vi "UNITEST MAIN v01.1.vi"() -> ()   [LabVIEW 2025]
uses:
  controls/LAB-IQ UI Data.ctl
  HEAVE vi's/Heave Write enum.ctl
  HEAVE vi's/Heave Right enum.ctl
  d081153b-36ca-4bc4-8478-749476f82ba4.vi
  02c5850b-52e8-4ed5-91f8-6f0ad62f4994.vi
  1223eb78-e4c4-4b69-bf80-185c82055158.vi
  e5651a45-6a49-4a3f-b503-ff1eaf449b4a.vi
  4095ce77-506c-41ec-8143-cc58e62a390f.vi
  support/Message Queue/Enqueue Message (Single).vi
  <vilib>/Utility/error.llb/Error Cluster From Error Code.vi
  <vilib>/ErrorRing/Error Ring.xnode
  support/Message Queue/LAB-IQ Message Queue.lvlib
  support/User Event - Stop/LAB-IQ User Event - Stop.lvlib
  SWAY vi's/Sway Write enum.ctl
  1202965f-721d-4349-8d61-5de826f379ef.vi
  SWAY vi's/Sway Right enum.ctl
panel:
  out "HEAVE ENABLE":bool
  in  "SPARE  5":u8
  in  "Manual Write SWAY":bool
  out "SWAY WRITE":string
  in  "SPARE  4":u8
  in  "SPARE  3":u8
  in  "SPARE 2":u8
  in  "SPARE 1":u8
  out "Spare 15":u8
  out "Spare 14":u8
  out "Spare 13":u8
  out "Spare 12":u8
  out "Spare 11":u8
  out "Spare 10":u8
  out "Spare 9":u8
  out "Spare 8":u8
  out "Spare 7":u8
  out "Spare 6":u8
  out "Spare 5":u8
  out "Spare 4":u8
  out "Spare 3":u8
  out "Spare 2":u8
  out "Spare 1":u8
  out "Node Id":u8
  out "Read SWAY Temp":bool
  out "fwMinor":u8
  out "fwMajor":u8
  out "faultCode":u16
  out "Rotary POSE":sgl format="%#.6f"
  out "SWAY POSE":sgl format="%#.6f"
  out "Homed":u8
  out "State":u8
  out "Ack ID":u16
  in  "SPEED":sgl=10000.0
  in  "Distance":sgl=10000.0
  in  "Mode Command":u8=2
  out "Sequence ID":u16
  out "error out Read SWAY":errorcluster
  out "error out Write  SWAY":errorcluster
  out "SWAY READ":string
  in  "min_finetune_floor":dbl=0.15
  in  "min_deadband_floor":dbl=0.05
  in  "fine_tune_pct":dbl=100.0
  out "Start Test Temp":bool
  in  "STOP":bool
  in  "AppLoadSeq scratch":bool
  out "Pulse delta":dbl
  in  "Fine Tune Zone":dbl=10.0
  in  "PID Delay (sec)":dbl=1.0 format="%#_6p"
  in  "Max_pos_limit":dbl=50000000.0
  in  "Min_pos_limit":dbl
  in  "i_limit":dbl=10.0
  in  "Max Step Linit":dbl=10.0
  in  "Init Step":dbl=10.0
  in  "pct_scale":dbl=100.0
  in  "Deadband":dbl=0.1
  in  "Kd":dbl
  in  "Ki":dbl
  in  "Kp":dbl=1.0
  out "Current Position":dbl
  in  "Set Load":dbl
  in  "Current Load":dbl
  in  "Manual Write Heave & Surge":bool
  out "Heave and Surge Write":string
  in  "Heave Loop Delay":dbl
  in  "Heave PID Speed":dbl=15.0
  in  "Surge Jog Speed":dbl=1.0 format="%.4f"
  in  "Heave Jog Speed":dbl=15.0
  in  "SPARE 4":u8
  in  "SPARE 3":u8
  in  "SPARE 2":u8
  in  "SPARE 1":u8
  out "Spare 15":u8
  out "Spare 14":u8
  out "Spare 13":u8
  out "Spare 12":u8
  out "Spare 11":u8
  out "Spare 10":u8
  out "Spare 9":u8
  out "Spare 8":u8
  out "Spare 7":u8
  out "Spare 6":u8
  out "Spare 5":u8
  out "Spare 4":u8
  out "Spare 3":u8
  out "Spare 2":u8
  out "Spare 1":u8
  out "Node Id":u8
  out "Read Heave Temp":bool
  out "fwMinor":u8
  out "fwMajor":u8
  out "faultCode":u16
  out "SURGE POSE":sgl format="%#.6f"
  out "HEAVE POSE":sgl format="%#.6f"
  out "Homed":u8
  out "State":u8
  out "Ack ID":u16
  in  "SPEED":sgl=10000.0
  in  "Distance":sgl=10000.0
  in  "Mode Command":u8=2
  out "Sequence ID":u16
  out "error out Read":errorcluster
  out "error out Write":errorcluster
  out "Heave and Surge Read":string
  out "Load Cell Temp":bool
  in  "Stop Scratch":bool
  in  "Enter Fixed SRR 2":dbl min=0.0 max=0.0 format="%.3f"
  in  "E.Velocity 2":bool=TRUE caption="SRR"
  out "Message":string="Load Entered is out of range!!!"
  in  "Tab Control 3":T1(tab)
  in  "Tab Control 5":enum32{""}(tab)
  in  "Tab Control 14":T2(tab)=enum."Motor Load"
  in  "Ramp MulFac":dbl=2.0
  in  "pulses LoadDiffRamp(2..10)":dbl=9.0
  in  "PulseControlRamp(diff<=3N)":dbl=5.0 min=1.0 max=1000.0 step=1.0 format="%#.1f"
  in  "SetLoadDeadband(%) Load(0-10N)":dbl=0.1 min=0.0001 max=100.0 step=0.0001 format="%#.6f"
  in  "PID gains out delay (microForce)":T3={"proportional gain (Kc)"=300.0, "integral time (Ti, min)"=0.00011, "derivative time (Td, min)"=0.0} {"derivative time (Td, min)" format="%.3f"; "integral time (Ti, min)" min=1e-05 max=100.0 step=1e-06 format="%.6f"; "proportional gain (Kc)" format="%.3f"}
  in  "Ramp":bool
  in  "Gain 2":dbl=0.016
  in  "pulses LoadDiff(2..10)":dbl=10.0
  in  "pulses LoadDiff(11..50)":dbl=40.0
  in  "PulseControl(diff<=3N)":dbl=1.0 min=1.0 max=1000.0 step=1.0 format="%#.1f"
  out "SetLoadDeadband(%)  2":dbl=1.0 min=0.001 max=100.0 step=0.001 format="%#.6f"
  in  "Dummy Run":bool
  out "Vertical load (N)":dbl format="%#.3f"
  in  "AutoTune":bool
  in  "Offset  3":dbl=1.5
  in  "apply load":bool
  in  "Enter ByPass Load":dbl
  in  "reinit 3":bool=TRUE
  in  "output range delay":cluster{"output high":dbl, "output low":dbl}={"output high"=100.0, "output low"=-100.0} {"output low" format="%.2f"; "output high" format="%.2f"}
  in  "PID gains out delay":T3={"proportional gain (Kc)"=30.0, "integral time (Ti, min)"=0.00101, "derivative time (Td, min)"=0.0} {"derivative time (Td, min)" format="%.3f"; "integral time (Ti, min)" min=1e-05 max=100.0 step=0.0001 format="%.4f"; "proportional gain (Kc)" format="%.3f"}
  in  "Bypass Load":bool
  in  "pulsesSent":dbl=200.0
  out "pulses":dbl
  out "actpid":dbl
  out "gFF Rot 7":cluster{dbl, dbl, dbl}(graph)
  in  "pulses LoadDiff(21..1000)":dbl=40.0
  in  "Delay":dbl=1.5 min=0.001 max=5.0 step=0.001 format="%#.6f"
  in  "deadband":dbl=0.2
  in  "Tab Control 26":enum32{"Page 1", "Page 2"}(tab)
  in  "ClearAll":bool
  out "Mz(Nm)":dbl[](array[numeric])
  out "My(Nm)":dbl[](array[numeric])
  out "Mx(Nm)":dbl[](array[numeric])
  in  "Save Dwell":dbl=0.015 caption="Save Dwell (sec)" min=0.0 max=5.0 step=0.001 format="%.3f"
  out "Mx":dbl[](graph)
  out "My":dbl[](graph)
  out "Mz":dbl[](graph)
  out "Fx(N)":dbl[](graph)
  out "Fy(N)":dbl[](graph)
  out "Fz(N)":dbl[](graph)
  in  "ZeroAll":bool
  in  "Acq Delay (ms)":dbl=10.0
  in  "Burst Delay (ms)":dbl=10.0
  out "model":string
  out "SN":i32
  out "FFx(N)":dbl[](array[numeric])
  in  "Sensor IP":string="192.168.1.100"
  in  "Port":i32=8080
  out "FFy(N)":dbl[](array[numeric])
  out "Load(N)":dbl[](array[numeric])
  out "AE":bool
  in  "delete Handle":bool
  in  "Create Handle":bool=TRUE
  out "ft_data":dbl[](array[numeric])=[1.0, 1.0, 1.0, 1.0, 1.0, 1.0]
  out "ft_range":dbl[](array[numeric])=[1.0, 1.0, 1.0, 1.0, 1.0, 1.0]
  in  "stop 6":bool
  out "running_flag":bool
  out "ft_udp_handle":i32
  out "get-data-return":i32
  out "get-range-return":i32
  out "zero-return":i32
  out "filter-return":i32
  out "initial-return":i32
  out "deleteHandle-result":i32
  in  "Tab Control 19":enum32{"Platform COM", "Config ", "DevInfo"}(tab)=enum."Config "
  in  "SAMPLES":dbl=100.0
  in  "Re-initilaize":bool
  in  "Filter ON/OFF":bool=TRUE
  in  "TracHomeSurgeOffsetCounts 10MM":dbl=505100.0
  in  "TracHomeSwayOffsetCounts 10MM":dbl=1432.0
  in  "Acoustic Emission:":dbl=1.0 min=0.0001 max=200.0 step=0.0001 format="%.4f"
  in  "Apply Filter (FF)":bool
  in  "Filter% 2":dbl=50.0 min=50.0 max=100.0 step=0.1 format="%.1f"
  in  "Apply Filter (Load)":bool=TRUE
  in  "Filter%":dbl=80.0 min=50.0 max=100.0 step=0.1 format="%.1f"
  in  "Sway distance (mm)":dbl=245.0
  in  "Surge distance (mm)":dbl=370.0
  in  "DataSavingLoopDelay(ms)":dbl=15.0
  in  "SAVE  2":bool
  in  "Enter Distance":bool caption="Enter Counts"
  in  "Sway Counts:":dbl=100.0 min=0.0 max=100000000.0 step=1.0 format="%.2f"
  in  "Distance (mm): 3":dbl=100.0 caption="Distance (mm):" min=0.0 max=1500.0 step=0.001 format="%.5f"
  in  "Surge Counts:":dbl=100.0 min=0.0 max=100000000.0 step=1.0 format="%.1f"
  in  "Distance (mm): 2":dbl=100.0 caption="Distance (mm):" min=0.0 max=1500.0 step=0.0001 format="%.3f"
  in  "Distance (mm):":dbl=100.0 min=0.0 max=1500.0 step=0.001 format="%.5f"
  in  "Heave Counts:":dbl=100.0 min=0.0 max=100000000.0 step=1.0
  in  "LRMHomeSurgeOffsetCounts":dbl=307197.0
  in  "LRMHomeSwayOffsetCounts":dbl=26880.0
  in  "TracHomeSurgeOffsetCounts 20MM":dbl=505100.0
  in  "TracHomeSwayOffsetCounts 20MM":dbl=1432.0
  in  "RotHomeSwayOffsetCounts":dbl=14656.0
  in  "RotHomeSurgeOffsetCounts":dbl=311465.0
  in  "Heave distance":dbl=340.0
  out "Zmm":dbl=1600.0
  out "Heave Pulses/mm":dbl=1600.0
  out "Surge Pulses/mm":dbl=1600.0
  out "Sway Pulses/mm":dbl=320.0
  in  "Heave Pitch":dbl=4.0
  in  "Surge Pitch":dbl=3.0
  in  "Sway Pitch":dbl=2.0
  in  "Heave PPR":dbl=6400.0
  in  "Surge PPR":dbl=6400.0
  in  "Sway PPR":dbl=6400.0
  in  "GUI":T4(tab)
  in  "Platform Settings":bool caption="Password"
  in  "Configure":bool caption="Password"
  in  "Home":bool caption="Password"
  in  "EXIT":bool
  in  "Analysis":bool caption="Password"
  in  "service 2":bool caption="Password"
  in  "MainPage":T5(tab)=enum."HOME"
  in  "Select Load Head":bool
  in  "Notes :":string
  in  "FILE":string
  in  "Sample ID :":string
  in  "Operator ID :":string
  in  "Operator Name :":string
  in  "Auto":bool caption="Power Status"
  out "mm/s  Surge":dbl=7.0 caption="Jog" min=0.001 max=50.0 step=0.0001 format="%.2f"
  in  "Update Surge Speed":bool
  out "Drive Error":string
  in  "Disable Axis Jog Soft Limits":bool
  out "mm/s  Sway":dbl=7.0 caption="Jog" min=0.001 max=50.0 step=0.0001 format="%.2f"
  out "Sway and Surge COM Status":bool=TRUE caption="Load COM Status"
  out "Heave COM Status":bool=TRUE caption="Load COM Status"
  in  "Enable Platform":bool
  in  "Surge Forward Main":bool
  in  "Surge Backward Main":bool
  in  "Sway Right Main":bool
  in  "Sway Left Main":bool
  in  "Heave Down Main":bool
  in  "Heave Up main":bool
  in  "Update Sway Speed":bool
  in  "Update Heave Speed":bool
  out "mm/s Heave":dbl=7.0 caption="Jog" min=0.001 max=30.0 step=0.0001 format="%.2f"
  in  "mm/sec":dbl=1.0 caption="Jog" min=0.001 max=50.0 step=0.001 format="%.2f"
  in  "mm":dbl=0.001 caption="Jog" min=0.001 max=200.0 step=0.0001 format="%#.3f"
  in  "Surface Analysis":bool
  in  "Imaging":bool
  in  "Image Analysis":bool
  in  "Post Analysis":bool
  in  "SSP 0.75":bool
  in  "SSP 0.5":bool
  in  "SSP 0.3":bool
  in  "Warning":enum32{"Page 2"}(tab)
  in  "gui GIF":enum32{"Check", "Deca", "kilo", "Micro"}(tab)
  out "Communication is established":bool=TRUE caption="Load COM Status"
  in  "Reference Sample":u16(ring) items=["None", "Brass", "Aluminium", "Mild Steel"]
  out "Load Cell Communication Slide":u8(slide)=1 min=1 max=10 step=1 scale=0.0..10.0
  in  "com 3":bool
  out "com":bool
  out "DecaForce COM Status":bool caption="Load COM Status"
  in  "Loading Mode":u16(ring) items=["Constant", "Ramp", "Steps", "Indentation"]
  in  "Enter the CoF Trip":dbl=1.0
  in  "Enter the Friction Force Trip":dbl=520.0 min=500.0 max=500.0 step=1.0 format="%#.1f"
  in  "Enter the Normal load Trip":dbl=520.0 min=500.0 max=500.0 step=0.001 format="%.3f"
  in  "KiloForce":bool
  in  "DecaForce":bool
  in  "MicroForce":bool
  in  "LHBack":bool
  in  "LHNext":bool
  in  "Load Selection":T6(tab)
  in  "Enter the Load  (N)":dbl=2.0 caption="Enter the Load (N)" min=2.0 max=50.0 step=0.1 format="%#.4f"
  in  "Enter the Final Load (N)":dbl=1.0 min=0.0 max=500.0 step=1.0 format="%#.0f"
  in  "Update":bool
  in  "Enter the Loading Rate (N/min)":dbl=60.0 min=60.0 max=1200.0 step=0.1 format="%.2f"
  out "Warning 2":bool
  in  "Stribeck Table  For loading":string[][](table)=[["", "", ""], ["", "", ""], ["", "", ""], ["", "", ""]]
  in  "Stribeck table":bool
  in  "seq":bool=TRUE
  in  "Clear 3":bool
  in  "Indentation":string[][](table)=[["Detection", "5", "2"], ["Unload", "0", "5"], ["Load", "10", "2"], ["Unload", "0", "5"], ["Detection", "5", "2"], ["Unload", "0", "5"]]
  in  "Multipoint":bool caption="Singlepoint"
  in  "AppLoad 4":bool
  in  "zNL":bool
  out "NL disp":dbl caption="Normal Load ( N )" min=-2000.0 max=2000.0 step=0.0001 format="%.1f"
  in  "Traction":bool
  in  "Surge Forward MM":bool
  in  "Surge Backward MM":bool
  in  "M3 Image":enum32{"Page 1", "Page 2"}(tab)
  in  "String 39":string="Jog heave to bring the upper sample closer to the lower sample within 1mm."
  in  "Sway Left MM":bool
  in  "Sway Right MM":bool
  in  "Disable Axis Jog Soft Limits":bool
  in  "mm":dbl=0.001 caption="Jog" min=0.001 max=5.0 step=0.0001 format="%#.3f"
  in  "Heave Down MM":bool
  in  "Heave Up MM":bool
  in  "Wear Track Diameter (mm)":dbl=5.0 caption="Wear Track Diameter (mm):" min=1.0 max=30.0 step=1.0 format="%.2f"
  in  "Set WTD":bool
  in  "HomeScratch":bool
  in  "HomeRot":bool
  in  "PlaceModule":bool
  in  "Motion Mode:":u16(ring) items=["Uniform Rotation", "Angular Oscillation", "Stribeck ", "Steps"]
  in  "LR Sway":bool
  in  "Rot Hor":bool
  in  "Rot Ver":bool
  in  "Scratch":bool
  in  "LR Cam":bool
  in  "MMBack":bool
  in  "MMNext":bool
  in  "Rotary Module Selection":T7(tab)
  in  "SPEED SELECTION :":enum32{"Speed in RPM", "Speed in m/sec"}(radio)=enum."Speed in m/sec"
  in  "TEST SELECTION":enum32{"Time", "Cycle"}(radio)
  in  "Enter the Speed(mm/sec)":dbl=1.0 min=0.1 max=10.0 step=0.1 format="%.1f"
  in  "Enter the Speed(RPM)":dbl=45.0 min=5.0 max=300.0 step=1.0
  in  "Enter the Frequency (Hz)":dbl=1.0 min=0.1 max=10.0 step=0.1 format="%.1f"
  in  "Enter the Angle (Deg)":dbl=45.0 min=5.0 max=300.0 step=1.0
  in  "Angular Oscillation Set":bool
  in  "Rotary Tab":enum32{"Page 1", "Page 2"}(tab)
  out "e.v/ssr 2":enum32{"E.V", "SSR"}(tab)
  in  "Enter the Final E.Velocity (m/s) 2":dbl=1.0 min=0.001 max=4.0 step=0.001 format="%.3f"
  in  "Enter initial E.Velocity (m/s) 2":dbl=2.0 min=0.001 max=4.0 step=0.001 format="%.3f"
  in  "Enter Fixed E.Velocity 2":dbl=1.0 min=0.001 max=2.0 step=0.001 format="%.3f"
  in  "Enter Final SRR 2":dbl=1.0 min=0.001 max=1.0 step=0.001 format="%.2f"
  in  "Enter initial SRR 2":dbl=1.0 min=0.001 max=1.0 step=0.001 format="%.2f"
  out "Final Speed (RPM) 3":dbl=1.0 min=0.1 max=3000.0 step=0.1 format="%.1f"
  out "Initial Speed (RPM) 2":dbl=100.0 min=0.1 max=3000.0 step=0.1 format="%.1f"
  in  "Enter the Final Velocity (m/s) 3":dbl=1.0 min=0.001 max=2.0 step=0.001 format="%.3f"
  in  "Enter initial Velocity (m/s)  3":dbl=2.0 min=0.001 max=2.0 step=0.001 format="%.3f"
  out "Ramp Up 2":bool caption="Ramp Down"
  in  "File Path :  2":path
  in  "Import 2":bool
  in  "Save 2":bool
  in  "SPEED SELECTION : rotary":enum32{"Speed in Rpm", "Speed in m/sec"}(radio)=enum."Speed in m/sec"
  in  "calculate rotary":bool
  in  "String 45":string="File Path Location : C:-->LAB-IQ 150 --> User Defined\n                                       Protocol-->File.txt"
  in  "Step Speed":enum32{"Step Speed", "Step (load-Speed)"}(tab)
  in  "StepTable For Speed":string[][](table)=[["", "", ""], ["", "", ""], ["", "", ""], ["", "", ""]]
  in  "StepTable For Load-Speed":string[][](table)=[["", "", ""], ["", "", ""], ["", "", ""], ["", "", ""]]
  in  "StepTable For Speed 3":string[][](table)=[["", "", ""], ["", "", ""], ["", "", ""], ["", "", ""]]
  in  "Motion Direction:  3":u16(ring) items=["Clockwise", "Counter Clockwise"]
  out "Humidity  Status  3":bool caption="Communication Status"
  out "Low Temp  Status  2":bool caption="Communication Status"
  out "TK4 status 2":bool caption="Communication Status"
  in  "String 40":string="Before selecting Acoustic make sure the sensor output pin is connected to A4."
  in  "Stage Temperature":dbl[](array[numeric])=[150.0, 230.0, 300.0, 350.0, 400.0, 450.0, 500.0]
  in  "Sample Temperature":dbl[](array[numeric])=[100.0, 150.0, 200.0, 250.0, 300.0, 350.0, 400.0]
  in  "Humidity (Amb)":bool
  in  "Clear List":bool
  out "Sensors Picked":string
  in  "Add to list":bool
  in  "Wear":bool
  in  "Vibration":bool
  in  "Humidity (Chamber)":bool
  in  "Temperature (Chamber)":bool
  in  "ECR":bool
  in  "Temperature (Amb)":bool
  in  "Microphone":bool
  in  "Acoustic Emission 3":bool
  in  "SNext":bool
  in  "APBack":bool
  in  "Enter the Temperature (°C):":dbl
  in  "Enter the Stage \nTemperature (°C):":dbl=20.0 min=20.0 max=150.0 step=1.0 format="%#.0f"
  in  "Enter the Humidity (%Rh):":dbl=30.0 min=30.0 max=85.0 step=1.0
  in  "Low Temp":bool
  in  "High Temp":bool
  in  "Humidity":bool
  in  "Main Screen Tab":T8(tab)
  in  "ClrLog":bool
  out "Trip Log":string
  in  "Start Test":bool
  out "Test status":bool caption="Test Status"
  out "AR Led":bool caption="AR"
  out "Data":bool=TRUE
  out "Health":bool=TRUE
  out "Sway COM Status":bool=TRUE caption="Load COM Status"
  out "Heave COM Status":bool=TRUE caption="Load COM Status"
  in  "Grp Tab":enum32{"Rot/LRM", "FBT"}(tab)
  in  "Sub Graph":T9(tab)
  in  "Speed Reset Graph":bool
  in  "Speed Tab":enum32{" Rotary Disc", "MTM Ball", "MTM Disc"}(tab)
  out "speed mm/sec":dbl(graph)=0.13298760003255525
  out "MTM BALL SPEED":dbl(graph)=0.13298760003255525
  out "MTM DISC  SPEED":dbl(graph)=0.13298760003255525
  in  "Temperature Reset":bool
  out "Temperature (deg c)":dbl(graph)=0.13298760003255525
  in  "ECR RESET":bool
  out "ECR":dbl(graph)=0.13298760003255525
  out "Acoustic Emission (mV)":dbl min=0.0 max=5000.0 step=0.1
  in  "Aqucostic Reset Graph":bool
  out "gACQUOS":dbl(graph)=0.13298760003255525
  in  "Humidity Reset Graph":bool
  out "HumrGp":dbl(graph)=0.13298760003255525
  out "SD (mm)":dbl caption="Sliding Distance ( mm )" min=-200.0 max=200.0 step=0.1 format="%.4f"
  in  "Siliding distance Reset Graph":bool
  out "SDGp":dbl(graph)=0.13298760003255525
  out "Hymidity":bool
  in  "Humidity Disable trip":bool=TRUE
  in  "CoF Trip  2":dbl=540.0 min=100.0 max=540.0 step=1.0
  out "Depth Trip":dbl=600.0
  in  "Depth Trip":bool=TRUE
  out "Weart Deapth":bool
  in  "Depth Reset Graph":bool
  out "Weart":bool
  in  "Depthz":bool
  out "Depth (µm)":dbl min=-200.0 max=200.0 step=0.1 format="%.1f"
  out "WearGp":dbl(graph)=0.13298760003255525
  out "NL Trip 2":dbl=600.0
  out "Load pid":bool
  in  "Load Disable Trip":bool=TRUE
  in  "Load Reset Graph":bool
  out "NL Display 4":dbl caption="Normal Load ( N )" min=-2000.0 max=2000.0 step=0.0001 format="%.1f"
  out "Main Chart 3":cluster{dbl, "NL disp":dbl, dbl}(graph)
  in  "FF Tab":T10(tab)
  in  "COF Reset Graph":bool
  in  "COF Disable Trip":bool=TRUE
  out "COF TRIP":dbl=600.0
  out "COF MAIN CHART":cluster{dbl, "NL disp":dbl, dbl}(graph)
  out "Friction Force (N)":dbl min=-2000.0 max=2000.0 step=0.0001 format="%.1f"
  in  "FF Reset Graph":bool
  in  "FF Disable Trip":bool=TRUE
  out "FF TRIP":dbl=600.0
  out "FF MAIN CHART":cluster{dbl, "NL disp":dbl, dbl}(graph)
  in  "BACK":bool
  out "Ambient \nTemperature":dbl min=0.0 max=5000.0 step=0.1 format="%.1f"
  out "Ambient\n Humidity":dbl min=0.0 max=5000.0 step=0.1 format="%.2f"
  out "NL disp 2":dbl caption="Normal Load ( N )" min=-2000.0 max=2000.0 step=0.0001 format="%.1f"
  out "Set Humidity":dbl caption="Set Humidity  (% Rh)" min=-2000.0 max=2000.0 step=1.0 format="%.1f"
  out "humidity disp":dbl caption="Humidity (% Rh)" min=-2000.0 max=2000.0 step=1.0 format="%.1f"
  in  "Humidity On":bool
  in  "zNL 2":bool
  out "NLt":bool
  in  "Load En":bool
  out "Freq (Hz)":dbl min=0.0 max=5000.0 step=0.1 format="%.4f"
  out "HumCOMStatus":bool caption="Communication Status"
  out "Load Communication":bool
  in  "Temp Tabs":enum32{"Low Temp", "High Temp"}(tab)=enum."High Temp"
  out "Controller  Status":bool
  out "ChamberTemp":dbl format="%#.1f"
  in  "SetTmp":dbl=-190.0 caption="Set Temperature (Deg C)" min=-190.0 max=100.0 step=1.0 format="%.1f"
  in  "Cooling":bool
  in  "Heater":bool
  out "TK4 status":bool caption="Controller  Status"
  out "ChamberTemp":dbl format="%#.1f"
  in  "SetTmp":dbl caption="Set Temperature (Deg C)" min=0.0 max=1000.0 step=1.0 format="%.1f"
  in  "Set Load (N)":dbl=100.0 min=0.01 max=1500.0 step=0.01 format="%.1f"
  in  "Time Tab":enum32{"cycles", "duration"}(tab)=enum."duration"
  out "Test Duration 4":dbl=600.0 caption="Test Duration\n(HH:MM:SS)" min=0.0083 max=180000.0 step=0.0001 format="%<%H:%M:%S>t"
  out "TEST CYCLE":dbl min=0.0 max=5000.0 step=0.01 format="%.2f"
  in  "TOTAL CYCLES":dbl min=0.0 max=5000.0 step=0.1 format="%.4f"
  out "Time ( HH:MM:SS ) 2":dbl min=0.0 max=144000.0 step=1.0 format="%<%H:%M:%S>t"
  in  "Test Duration":dbl=600.0 caption="Test Duration\n(HH:MM:SS)" min=0.0083 max=180000.0 step=0.0001 format="%<%H:%M:%S>t"
  in  "Main Speed Tab":enum32{"ROTARY", "TRACTION"}(tab)
  in  "SPEED TAB":enum32{"RPM", "m/sec"}(tab)
  out "Speed (RPM)":dbl min=0.0 max=5000.0 step=0.1 format="%.1f"
  out "Set Speed":dbl caption="Set Speed (RPM)" min=0.0 max=1500.0 step=0.1 format="%.1f"
  out "Speed (m/sec)":dbl min=0.0 max=5000.0 step=0.001 format="%.4f"
  out "Set Speed (m/sec)":dbl min=0.0 max=1500.0 step=0.001 format="%.4f"
  in  "MTM MOTOR DISPLAY":enum32{"MTM RPM", "MTM m/sec"}(tab)
  out "Disc Speed (RPM)":dbl min=0.0 max=1500.0 step=0.1 format="%.1f"
  out "Ball Speed (RPM)":dbl min=0.0 max=1500.0 step=0.1 format="%.1f"
  out "Disc Speed (m/sec)":dbl min=0.0 max=1500.0 step=0.1 format="%.1f"
  out "Ball Speed (m/sec)":dbl min=0.0 max=1500.0 step=0.1 format="%.1f"
  in  "Angle and Frequency":enum32{"angular", "lrm"}(tab)
  out "Angle (Deg)":dbl min=0.0 max=5000.0 step=0.01 format="%.2f"
  out "Stroke (mm)":dbl min=0.0 max=5000.0 step=0.01 format="%.2f"
  in  "Analysis Home":bool
  in  "Password":string
  in  "Home Service":bool
  in  "Advanced Setting":bool
  in  "About Tab":enum32{"Primary"}(tab)
  in  "ECR Port:":refnum<visa-resource-name>="COM10"
  in  "Ramp Port:":refnum<visa-resource-name>="COM10"
  in  "Installation/Replacement completed":bool
  in  "Loahead":bool
  in  "Heave and Surge COM Port:":refnum<visa-resource-name>="COM9"
  in  "Sway COM Port:":refnum<visa-resource-name>="COM10"
  in  "Temp Modbus:":refnum<visa-resource-name>="COM14"
  in  "Humidity Port:":refnum<visa-resource-name>="COM10"
  in  "Edit Gain Constants":bool
  in  "Save Gain Constants":bool
  in  "Service About":bool
  # "load Aquisition off"
  # "load Aquisition On"
  # "Configuration"
  # "Limits for Heave Surge and Sway"
  # "Modules Offset Parameters"
  # "Counts-Distance Calculator"
  # "File Name :"
  # "Ensure the traction module is aligned\n horizontally with the stage before ENABLE."
  # "SET JOG SPEED"
  # "JOG MODE"
  # "Module Selection"
  # "Positioning Control"
  # "Connect the controller\ncable to M3"
  # "Environment"
  # "Sensors"
  # "Data Points"
  # "Data Points"
  # "Data Points"
  # "Data Points"
  # "ohms"
  # "Data Points"
  # "Data Points"
  # "Data Points"
  # "LAB-IQ 150 / UNITEST / WO2456 / UT150  v05 / AUGUST 2025"
  # "NOTE: This operation needs to be done only when the machine is ON."
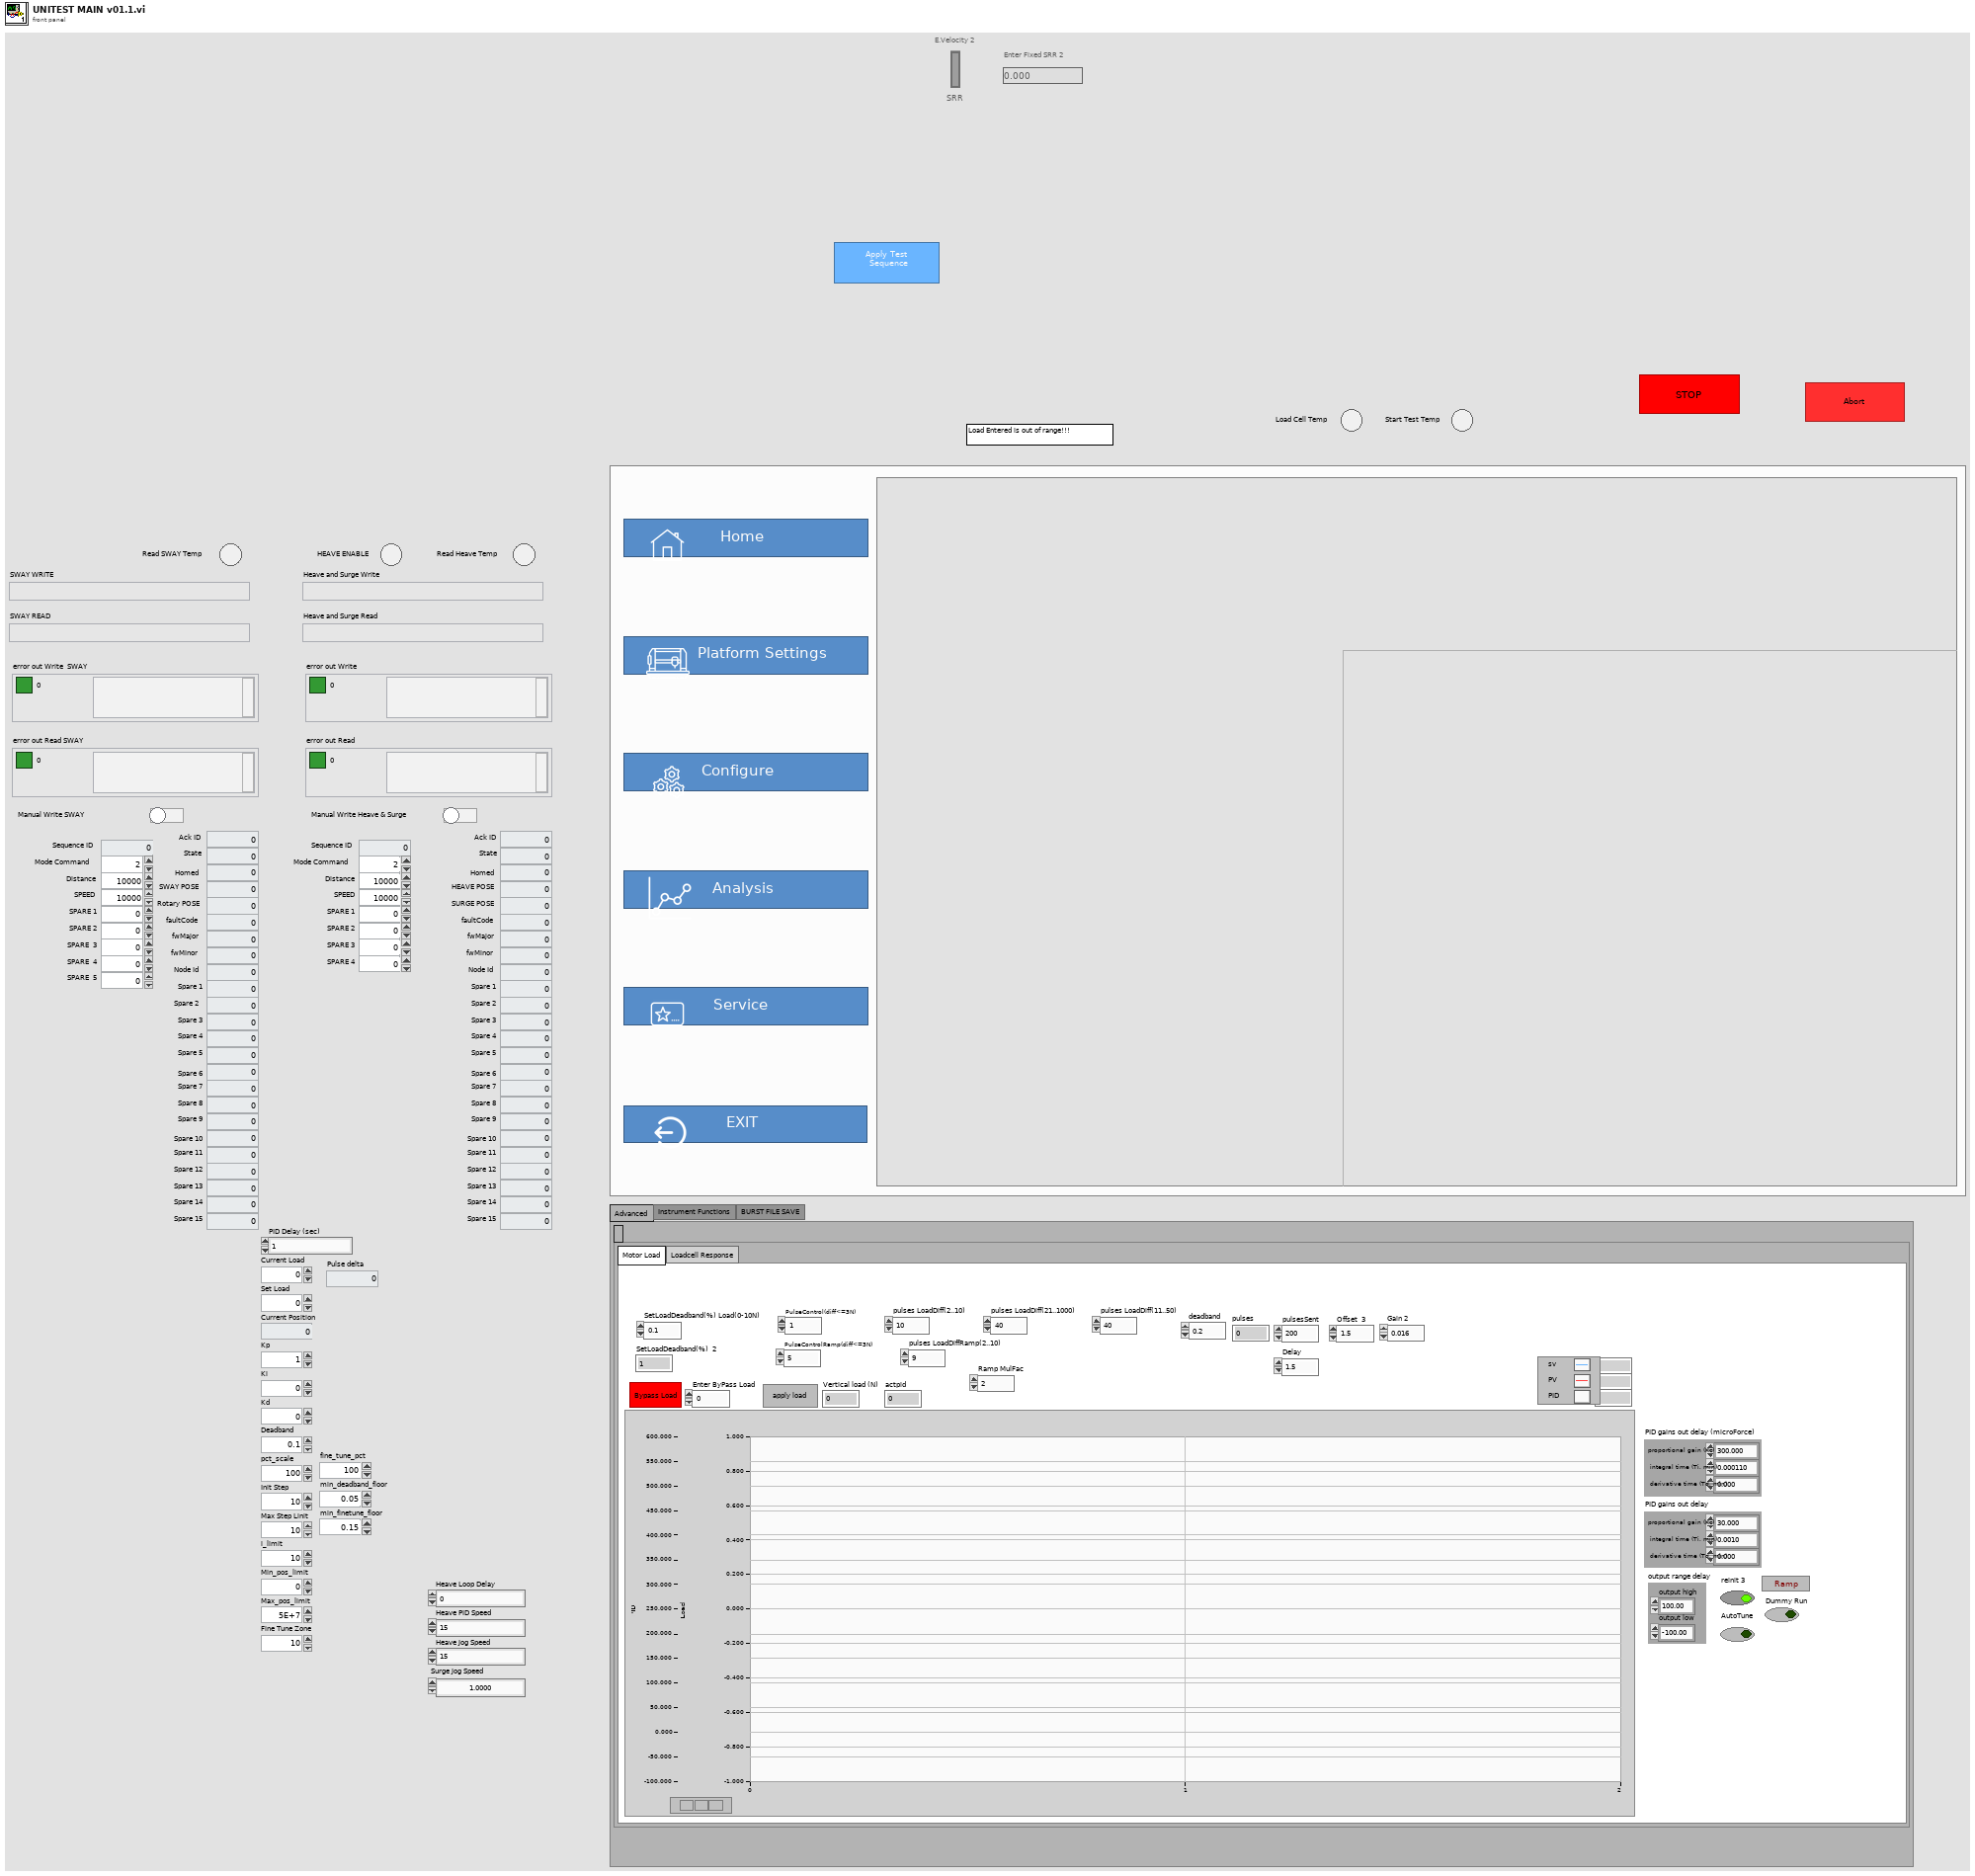
[diagram p1: front panel]
types:
  T1 = enum32{"Advanced", "Motor", "Depth_graph", "UIO Communicator", "Add to list parametrs", "Instrument Functions", "BURST FILE SAVE"}
  T2 = enum32{"LRM heating", "FBT_Heating", "Motor Load", "Loadcell Response", "Voice Load", "Step loading and speed ", "Depth"}
  T3 = cluster{"proportional gain (Kc)":dbl, "integral time (Ti, min)":dbl, "derivative time (Td, min)":dbl}
  T4 = enum32{"Setup", "Load Head", "Motion Module", "Environment", "Begin"}
  T5 = enum32{"Details", "PlatformSetting", "Analysis", "HOME"}
  T6 = enum32{"Constant", "Ramp", "Step", "Indentation"}
  T7 = enum32{"Uniform Rotation", "Angular Oscillation", "Speed Ramp", "Speed Step"}
  T8 = enum32{"  Acquire  ", "Compare Files Rot", "About", "Service"}
  T9 = enum32{"Speed", "Temperature", "ECR", "Acoustic Emission", "Humidity", "Sliding Distance"}
  T10 = enum32{"Coefficient of Friction ", "Friction Force (N)"}
  T11 = typedef "LAB-IQ UI Data.ctl" = cluster{"Main Home Screen":cluster{"GUI":refnum<vi>, "Platform Settings":refnum<vi>, "Configure":refnum<vi>, "Home":refnum<vi>, "EXIT":refnum<vi>, "service 2":refnum<vi>, "MainPage":refnum<vi>, "Analysis":refnum<vi>}, "Platform Settings":cluster{"mm/s  Surge":refnum<vi>, "Update Surge Speed":refnum<vi>, "Drive Error":refnum<vi>, "Disable Axis Jog Soft Limits":refnum<vi>, "mm/s  Sway":refnum<vi>, "Sway and Surge COM Status":refnum<vi>, "Heave COM Status":refnum<vi>, "Enable Platform":refnum<vi>, "Surge Forward Main":refnum<vi>, "Sway Right Main":refnum<vi>, "Sway Left Main":refnum<vi>, "Heave Down Main":refnum<vi>, "Heave Up main":refnum<vi>, "Update Sway Speed":refnum<vi>, "Update Heave Speed":refnum<vi>, "mm/s Heave":refnum<vi>, "mm/sec":refnum<vi>, "mm":refnum<vi>, "Surge Backward Main":refnum<vi>}, "Analysis Screen":cluster{"Analysis Home":refnum<vi>, "Surface Analysis":refnum<vi>, "Imaging":refnum<vi>, "Image Analysis":refnum<vi>, "Post Analysis":refnum<vi>}, "Config Screen":cluster{"Select Load Head":refnum<vi>, "Notes :":refnum<vi>, "FILE":refnum<vi>, "Sample ID :":refnum<vi>, "Operator ID :":refnum<vi>, "Operator Name :":refnum<vi>, "Auto":refnum<vi>}, "Motion Module":cluster{"zNL":refnum<vi>, "NL disp":refnum<vi>, "Rotary Tab":refnum<vi>, "Motion Direction:  3":refnum<vi>, "E.Velocity 2":refnum<vi>, "e.v/ssr 2":refnum<vi>, "Enter Fixed E.Velocity 2":refnum<vi>, "Enter Final SRR 2":refnum<vi>, "Enter initial SRR 2":refnum<vi>, "Enter Fixed SRR 2":refnum<vi>, "Enter the Final E.Velocity (m/s) 2":refnum<vi>, "Enter initial E.Velocity (m/s) 2":refnum<vi>, "Final Speed (RPM) 3":refnum<vi>, "Initial Speed (RPM) 2":refnum<vi>, "Enter the Final Velocity (m/s) 3":refnum<vi>, "Enter initial Velocity (m/s)  3":refnum<vi>, "Ramp Up 2":refnum<vi>, "TEST SELECTION":refnum<vi>, "SPEED SELECTION : ":refnum<vi>, "Angular Oscillation Set":refnum<vi>, "Traction":refnum<vi>, "Step Speed":refnum<vi>, "StepTable For Load-Speed":refnum<vi>, "StepTable For Speed":refnum<vi>, "Surge Forward MM":refnum<vi>, "Surge Backward MM":refnum<vi>, "M3 Image":refnum<vi>, "String 39":refnum<vi>, "Sway Left MM":refnum<vi>, "Sway Right MM":refnum<vi>, "Disable Axis Jog Soft Limits":refnum<vi>, "mm":refnum<vi>, "Heave Down MM":refnum<vi>, "Heave Up MM":refnum<vi>, "Wear Track Diameter (mm)":refnum<vi>, "Set WTD":refnum<vi>, "HomeScratch":refnum<vi>, "HomeRot":refnum<vi>, "PlaceModule":refnum<vi>, "Enter the Angle (Deg)":refnum<vi>, "Enter the Frequency (Hz)":refnum<vi>, "Motion Mode:":refnum<vi>, "LR Sway":refnum<vi>, "Rot Hor":refnum<vi>, "Scratch":refnum<vi>, "LR Cam":refnum<vi>, "MMBack":refnum<vi>, "MMNext":refnum<vi>, "Rot Ver":refnum<vi>, "Rotary Module Selection":refnum<vi>, "calculate rotary":refnum<vi>, "SPEED SELECTION : rotary":refnum<vi>, "Import 2":refnum<vi>, "Save 2":refnum<vi>, "File Path :  2":refnum<vi>, "String 45":refnum<vi>, "StepTable For Speed 3":refnum<vi>, "Enter the Speed(mm/sec)":refnum<vi>, "Enter the Speed(RPM)":refnum<vi>}, "Environmental control":cluster{"Humidity  Status  3":refnum<vi>, "Low Temp  Status  2":refnum<vi>, "TK4 status 2":refnum<vi>, "Stage Temperature":refnum<vi>, "Sample Temperature":refnum<vi>, "Humidity (Amb)":refnum<vi>, "Clear List":refnum<vi>, "Add to list":refnum<vi>, "Wear":refnum<vi>, "Vibration":refnum<vi>, "Humidity (Chamber)":refnum<vi>, "Temperature (Chamber)":refnum<vi>, "ECR ":refnum<vi>, "Temperature (Amb)":refnum<vi>, "Microphone":refnum<vi>, "Acoustic Emission 3":refnum<vi>, "SNext":refnum<vi>, "APBack":refnum<vi>, "Enter the Temperature (°C):":refnum<vi>, "Enter the Stage \nTemperature (°C):":refnum<vi>, "Enter the Humidity (%Rh):":refnum<vi>, "Low Temp":refnum<vi>, "High Temp":refnum<vi>, "Humidity":refnum<vi>, "Sensors Picked":refnum<vi>}, "About Screen":cluster{"Password":refnum<vi>, "Home Service":refnum<vi>, "Advanced Setting":refnum<vi>, "About Tab":refnum<vi>, "ECR Port:":refnum<vi>, "Ramp Port:":refnum<vi>, "Installation/Replacement completed":refnum<vi>, "Loahead":refnum<vi>, "Heave and Surge COM Port:":refnum<vi>, "Sway COM Port:":refnum<vi>, "Temp Modbus:":refnum<vi>, "Humidity Port:":refnum<vi>, "Edit Gain Constants":refnum<vi>, "Save Gain Constants":refnum<vi>}, "Main Screen":cluster{"Main Screen Tab":refnum<vi>, "Angle and Frequency":refnum<vi>, "Stroke (mm)":refnum<vi>, "Angle (Deg)":refnum<vi>, "Main Speed Tab":refnum<vi>, "MTM MOTOR DISPLAY":refnum<vi>, "Disc Speed (m/sec)":refnum<vi>, "Ball Speed (m/sec)":refnum<vi>, "Disc Speed (RPM)":refnum<vi>, "Ball Speed (RPM)":refnum<vi>, "SPEED TAB":refnum<vi>, "Speed (m/sec)":refnum<vi>, "Set Speed (m/sec)":refnum<vi>, "Speed (RPM)":refnum<vi>, "Set Speed":refnum<vi>, "Time Tab":refnum<vi>, "Time ( HH:MM:SS ) 2":refnum<vi>, "Test Duration":refnum<vi>, "Test Duration 4":refnum<vi>, "TEST CYCLE":refnum<vi>, "TOTAL CYCLES":refnum<vi>, "Set Load (N)":refnum<vi>, "Temp Tabs":refnum<vi>, "Heater":refnum<vi>, "TK4 status":refnum<vi>, "ChamberTemp":refnum<vi>, "SetTmp":refnum<vi>, "Controller  Status":refnum<vi>, "ChamberTemp 2":refnum<vi>, "SetTmp 2":refnum<vi>, "Controller  Status 2":refnum<vi>, "ChamberTemp 3":refnum<vi>, "SetTmp 3":refnum<vi>, "Cooling":refnum<vi>, "Load Communication":refnum<vi>, "Ambient \nTemperature":refnum<vi>, "HumCOMStatus":refnum<vi>, "Ambient\n Humidity":refnum<vi>, "Freq (Hz)":refnum<vi>, "Load En":refnum<vi>, "NLt":refnum<vi>, "zNL 2":refnum<vi>, "Humidity On":refnum<vi>, "humidity disp":refnum<vi>, "Set Humidity":refnum<vi>, "NL disp 2":refnum<vi>, "Humidity On 2":refnum<vi>, "humidity disp 2":refnum<vi>, "Set Humidity 2":refnum<vi>, "NL disp 3":refnum<vi>, "AppLoadSeq scratch":refnum<vi>, "Stop Scratch":refnum<vi>, "ClrLog":refnum<vi>, "Trip Log":refnum<vi>, "STOP":refnum<vi>, "Start Test":refnum<vi>, "Test status":refnum<vi>, "AR Led":refnum<vi>, "Data":refnum<vi>, "Health":refnum<vi>, "Sway COM Status":refnum<vi>, "Heave COM Status":refnum<vi>, "Grp Tab":refnum<vi>, "Sub Graph":refnum<vi>, "SD (mm)":refnum<vi>, "Siliding distance Reset Graph":refnum<vi>, "SDGp":refnum<vi>, "Humidity Reset Graph":refnum<vi>, "HumrGp":refnum<vi>, "Acoustic Emission (mV)":refnum<vi>, "Aqucostic Reset Graph":refnum<vi>, "gACQUOS":refnum<vi>, "ECR RESET":refnum<vi>, "ECR":refnum<vi>, "Temperature Reset":refnum<vi>, "Acoustic Emission (mV) 2":refnum<vi>, "Aqucostic Reset Graph 2":refnum<vi>, "gACQUOS 2":refnum<vi>, "ECR RESET 2":refnum<vi>, "ECR 2":refnum<vi>, "Temperature Reset 2":refnum<vi>, "Temperature (deg c)":refnum<vi>, "Speed Reset Graph":refnum<vi>, "Speed Tab":refnum<vi>, "MTM DISC  SPEED":refnum<vi>, "MTM BALL SPEED":refnum<vi>, "speed mm/sec":refnum<vi>, "Hymidity":refnum<vi>, "Humidity Disable trip":refnum<vi>, "CoF Trip  2":refnum<vi>, "Depth Trip":refnum<vi>, "Weart Deapth":refnum<vi>, "Depth Reset Graph":refnum<vi>, "Weart":refnum<vi>, "Depthz":refnum<vi>, "Depth (µm)":refnum<vi>, "WearGp":refnum<vi>, "NL Trip 2":refnum<vi>, "Load pid":refnum<vi>, "Load Disable Trip":refnum<vi>, "Load Reset Graph":refnum<vi>, "NL Display 4":refnum<vi>, "Main Chart 3":refnum<vi>, "BACK":refnum<vi>, "Depth Trip 2":refnum<vi>, "COF TRIP ":refnum<vi>, "Friction Force (N)":refnum<vi>, "FF Reset Graph":refnum<vi>, "FF Disable Trip":refnum<vi>, "FF TRIP":refnum<vi>, "FF MAIN CHART":refnum<vi>, "COF Disable Trip":refnum<vi>, "COF Reset Graph":refnum<vi>, "COF MAIN CHART":refnum<vi>, "FF Tab":refnum<vi>, "Start Test Temp":refnum<vi>}, "Loading":cluster{"Indentation":refnum<vi>, "Reference Sample":refnum<vi>, "Load Cell Communication Slide":refnum<vi>, "com 3":refnum<vi>, "com":refnum<vi>, "DecaForce COM Status":refnum<vi>, "Update":refnum<vi>, "Clear 3":refnum<vi>, "seq":refnum<vi>, "Stribeck table":refnum<vi>, "Stribeck Table  For loading":refnum<vi>, "Loading Mode":refnum<vi>, "Enter the Final Load (N)":refnum<vi>, "Enter the CoF Trip":refnum<vi>, "Enter the Friction Force Trip":refnum<vi>, "Enter the Normal load Trip":refnum<vi>, "Enter the Load  (N)":refnum<vi>, "KiloForce":refnum<vi>, "DecaForce ":refnum<vi>, "MicroForce":refnum<vi>, "LHBack":refnum<vi>, "LHNext":refnum<vi>, "Enter the Loading Rate (N/min)":refnum<vi>, "Message":refnum<vi>, "Warning 2":refnum<vi>, "SSP 0.75":refnum<vi>, "SSP 0.5":refnum<vi>, "SSP 0.3":refnum<vi>, "Warning":refnum<vi>, "gui GIF":refnum<vi>, "Communication is established":refnum<vi>, "AppLoad 4":refnum<vi>, "Multipoint":refnum<vi>, "Load Selection":refnum<vi>}, "PID":cluster{"Ramp MulFac":refnum<vi>, "pulses LoadDiffRamp(2..10)":refnum<vi>, "PulseControlRamp(diff<=3N)":refnum<vi>, "SetLoadDeadband(%) Load(0-10N)":refnum<vi>, "PID gains out delay (microForce)":refnum<vi>, "Ramp":refnum<vi>, "Gain 2":refnum<vi>, "pulses LoadDiff(2..10)":refnum<vi>, "pulses LoadDiff(11..50)":refnum<vi>, "PulseControl(diff<=3N)":refnum<vi>, "SetLoadDeadband(%)  2":refnum<vi>, "Dummy Run":refnum<vi>, "Vertical load (N)":refnum<vi>, "AutoTune":refnum<vi>, "Offset 3 ":refnum<vi>, "apply load":refnum<vi>, "Offset  3":refnum<vi>, "apply load 2":refnum<vi>, "Enter ByPass Load":refnum<vi>, "reinit 3":refnum<vi>, "output range delay":refnum<vi>, "PID gains out delay":refnum<vi>, "Bypass Load":refnum<vi>, "pulsesSent":refnum<vi>, "pulses ":refnum<vi>, "actpid":refnum<vi>, "gFF Rot":refnum<vi>, "pulses LoadDiff(21..1000)":refnum<vi>, "Delay":refnum<vi>, "deadband":refnum<vi>}, "Config Parameters":cluster{"Tab Control 3":refnum<vi>, "Tab Control 19":refnum<vi>, "SAMPLES":refnum<vi>, "Re-initilaize":refnum<vi>, "Filter ON/OFF":refnum<vi>, "TracHomeSurgeOffsetCounts 10MM":refnum<vi>, "TracHomeSwayOffsetCounts 10MM":refnum<vi>, "Acoustic Emission:":refnum<vi>, "Apply Filter (FF)":refnum<vi>, "Filter% 2":refnum<vi>, "Apply Filter (Load)":refnum<vi>, "Filter% ":refnum<vi>, "Sway distance (mm)":refnum<vi>, "Surge distance (mm)":refnum<vi>, "DataSavingLoopDelay(ms)":refnum<vi>, "SAVE 2":refnum<vi>, "Enter Distance":refnum<vi>, "Sway Counts:":refnum<vi>, "Distance (mm): 3":refnum<vi>, "Surge Counts:":refnum<vi>, "Distance (mm): 2":refnum<vi>, "Distance (mm):":refnum<vi>, "Heave Counts:":refnum<vi>, "LRMHomeSurgeOffsetCounts":refnum<vi>, "LRMHomeSwayOffsetCounts":refnum<vi>, "TracHomeSurgeOffsetCounts 20MM":refnum<vi>, "TracHomeSwayOffsetCounts 20MM":refnum<vi>, "RotHomeSwayOffsetCounts":refnum<vi>, "RotHomeSurgeOffsetCounts":refnum<vi>, "Heave distance":refnum<vi>, "Zmm":refnum<vi>, "Heave Pulses/mm":refnum<vi>, "Surge Pulses/mm":refnum<vi>, "Sway Pulses/mm":refnum<vi>, "Heave Pitch":refnum<vi>, "Surge Pitch":refnum<vi>, "Sway Pitch":refnum<vi>, "Heave PPR":refnum<vi>, "Surge PPR":refnum<vi>, "Sway PPR":refnum<vi>, "Tab Control 5":refnum<vi>, "Tab Control 14":refnum<vi>, "Tab Control 26":refnum<vi>, "AE":refnum<vi>, "Heave Loop Delay":refnum<vi>, "Heave PID Speed":refnum<vi>, "Surge Jog Speed":refnum<vi>, "Heave Jog Speed":refnum<vi>}, "Loading Com Port":cluster{"ClearAll":refnum<vi>, "Mz(Nm)":refnum<vi>, "My(Nm)":refnum<vi>, "Mx(Nm)":refnum<vi>, "Save Dwell":refnum<vi>, "Mx ":refnum<vi>, "My ":refnum<vi>, "Mz":refnum<vi>, "Fx(N)":refnum<vi>, "Fy(N)":refnum<vi>, "Fz(N)":refnum<vi>, "ZeroAll":refnum<vi>, "Acq Delay (ms)":refnum<vi>, "Burst Delay (ms)":refnum<vi>, "model":refnum<vi>, "SN":refnum<vi>, "FFx(N)":refnum<vi>, "Sensor IP":refnum<vi>, "Port":refnum<vi>, "FFy(N)":refnum<vi>, "Load(N)":refnum<vi>, "delete Handle":refnum<vi>, "Create Handle":refnum<vi>, "ft_data":refnum<vi>, "ft_range":refnum<vi>, "ft_data 2":refnum<vi>, "stop 6":refnum<vi>, "running_flag":refnum<vi>, "ft_udp_handle":refnum<vi>, "get-data-return":refnum<vi>, "get-range-return":refnum<vi>, "zero-return":refnum<vi>, "filter-return":refnum<vi>, "initial-return":refnum<vi>, "deleteHandle-result":refnum<vi>, "Load Cell Temp":refnum<vi>}, "Heave AND Surge":cluster{"SURGE POSE":refnum<vi>, "error out Read":refnum<vi>, "HEAVE POSE":refnum<vi>, "State":refnum<vi>, "Homed":refnum<vi>, "Sequence ID":refnum<vi>, "error out Write":refnum<vi>, "faultCode":refnum<vi>, "Ack ID":refnum<vi>, "SPEED":refnum<vi>, "Distance":refnum<vi>, "Mode Command":refnum<vi>, "Heave and Surge Read":refnum<vi>, "Read Heave Temp":refnum<vi>, "Spare 15":refnum<vi>, "Spare 14":refnum<vi>, "Spare 13":refnum<vi>, "Spare 12":refnum<vi>, "Spare 11":refnum<vi>, "Spare 10":refnum<vi>, "Spare 9":refnum<vi>, "Spare 8":refnum<vi>, "Spare 7":refnum<vi>, "Spare 6":refnum<vi>, "Spare 5":refnum<vi>, "Spare 4":refnum<vi>, "Spare 2":refnum<vi>, "Spare 1":refnum<vi>, "Node Id":refnum<vi>, "Spare 3":refnum<vi>, "SPARE 4":refnum<vi>, "SPARE 3":refnum<vi>, "SPARE 2":refnum<vi>, "SPARE 1":refnum<vi>, "fwMajor":refnum<vi>, "fwMinor":refnum<vi>, "Manual Write":refnum<vi>, "Heave and Surge Write":refnum<vi>}, "New PID LOGIC":cluster{"Fine Tune Zone":refnum<vi>, "PID SDelay":refnum<vi>, "Max_pos_limit":refnum<vi>, "Min_pos_limit":refnum<vi>, "i_limit":refnum<vi>, "pct_scale":refnum<vi>, "Deadband":refnum<vi>, "Kd":refnum<vi>, "Ki":refnum<vi>, "Kp":refnum<vi>, "Current Position":refnum<vi>, "Set Load":refnum<vi>, "Current Load":refnum<vi>, "Pulse delta":refnum<vi>, "Init Step":refnum<vi>, "Max Step Linit":refnum<vi>}, "SWAY ":cluster{"fwMajor":refnum<vi>, "Homed":refnum<vi>, "Rotary POSE":refnum<vi>, "State":refnum<vi>, "SWAY POSE":refnum<vi>, "Ack ID":refnum<vi>, "faultCode":refnum<vi>, "Node Id":refnum<vi>, "fwMinor":refnum<vi>, "Spare 6":refnum<vi>, "Spare 5":refnum<vi>, "Spare 4":refnum<vi>, "Spare 3":refnum<vi>, "Spare 2":refnum<vi>, "Spare 1":refnum<vi>, "Spare 7":refnum<vi>, "SPARE  5":refnum<vi>, "error out Write  SWAY ":refnum<vi>, "error out Read SWAY ":refnum<vi>, "Manual Write SWAY ":refnum<vi>, "SWAY WRITE":refnum<vi>, "SPARE  4":refnum<vi>, "SPARE  3":refnum<vi>, "SPARE 2":refnum<vi>, "SPARE 1":refnum<vi>, "Spare 15":refnum<vi>, "Spare 14":refnum<vi>, "Spare 13":refnum<vi>, "Spare 12":refnum<vi>, "Spare 11":refnum<vi>, "Spare 9":refnum<vi>, "Spare 8":refnum<vi>, "SPEED":refnum<vi>, "Distance":refnum<vi>, "Mode Command":refnum<vi>, "Sequence ID":refnum<vi>, "SWAY READ":refnum<vi>, "Spare 10":refnum<vi>, "Read SWAY Temp":refnum<vi>}}
  T12 = typedef "init queue out loop.ctl" = cluster{"UI Loop":refnum<queue>, "LOAD COM LOOP ":refnum<queue>, "SWAY MOTOR COM LOOP":refnum<queue>, "HEAVE MOTOR COM LOOP":refnum<queue>, "TEMPERATURE COM LOOP":refnum<queue>, "RAMP MOTOR COM LOOP":refnum<queue>, "ECR PORT":refnum<queue>, "HUMIDITY COM PORT":refnum<queue>, "PROGRAM LOOP":refnum<queue>, "MONITOR LOOP":refnum<queue>, "REPORT":refnum<queue>, "LOAD PID":refnum<queue>}
  T13 = enum8{"Enabled", "Disabled", "Disabled and Grayed Out"}
  T14 = enum16{"INIT", "SETLOWPASSFILTER", "SETZERO", "GETSENSORINFO", "GETRANGE", "ZEROALL", "READDATA", "UNINITIAL", "DELETEHANDLE"}
  T15 = typedef "Heave Write enum.ctl" = enum16{"INIT", "WRITE", "CLOSE", "REINIT"}
  T16 = typedef "Sway Write enum.ctl" = enum16{"INIT", "WRITE", "CLOSE", "REINIT"}
  T17 = typedef "Sway Right enum.ctl" = enum16{"INIT", "READ", "CLOSE", "REINIT", ""}
  T18 = typedef "Heave Right enum.ctl" = enum16{"INIT", "READ", "CLOSE", "REINIT", ""}
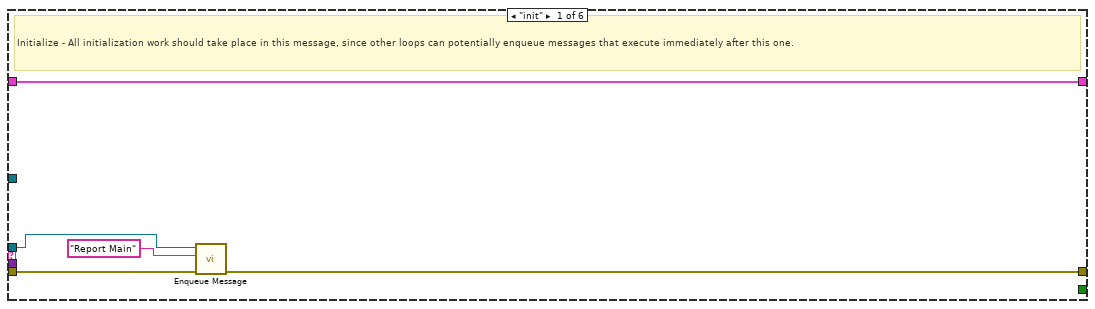
[diagram p2: hidden frame]
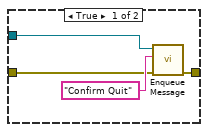
[diagram p3: hidden frame]
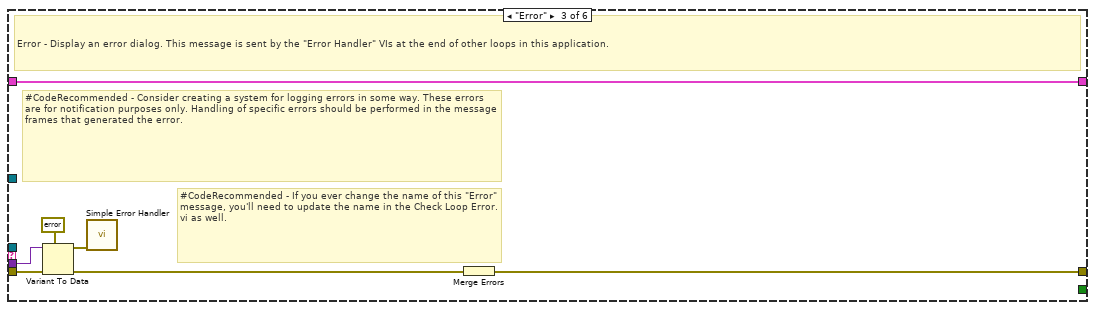
[diagram p4: hidden frame]
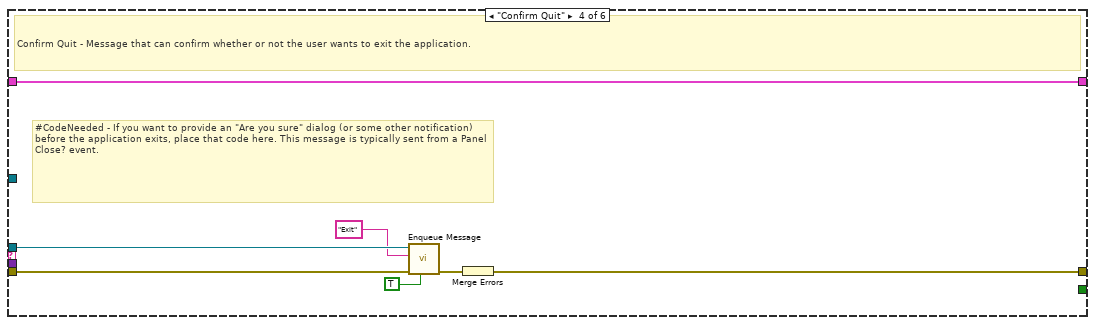
[diagram p5: hidden frame]
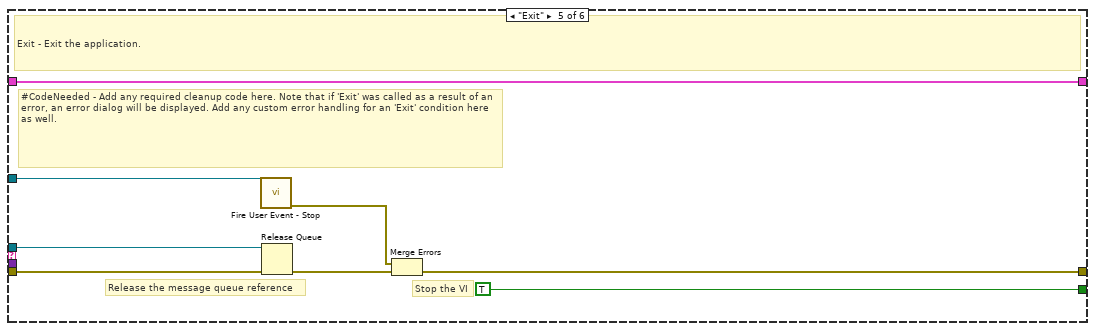
[diagram p6: hidden frame]
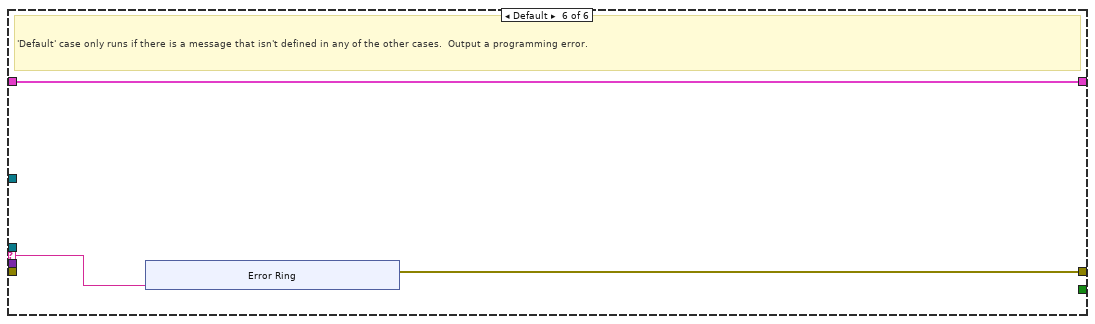
[diagram p7: hidden frame]
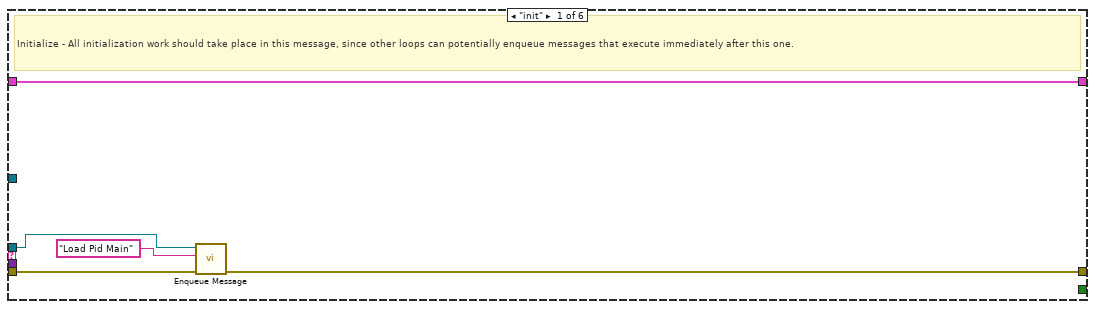
[diagram p8: hidden frame]
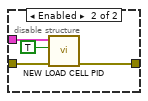
[diagram p10: hidden frame]
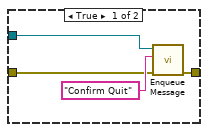
[diagram p11: hidden frame]
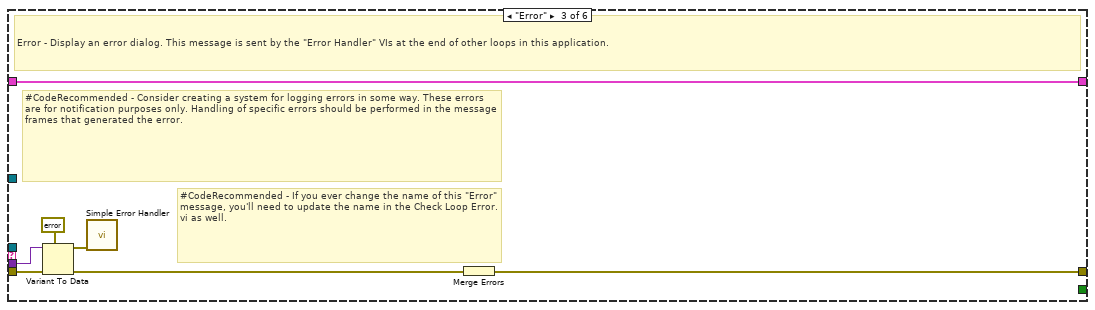
[diagram p12: hidden frame]
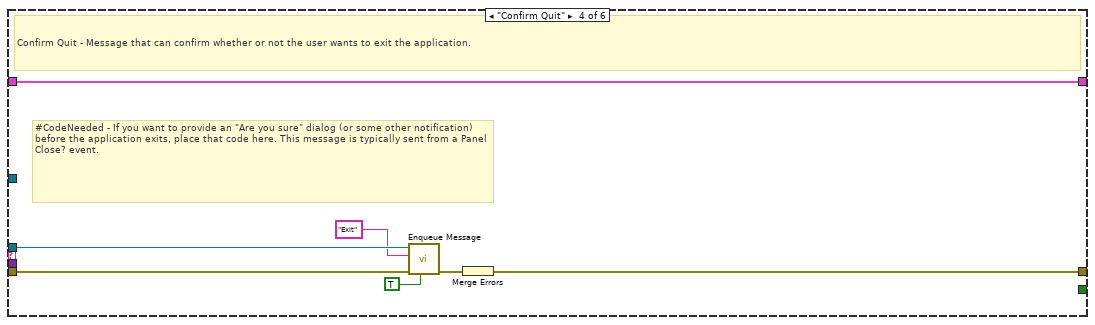
[diagram p13: hidden frame]
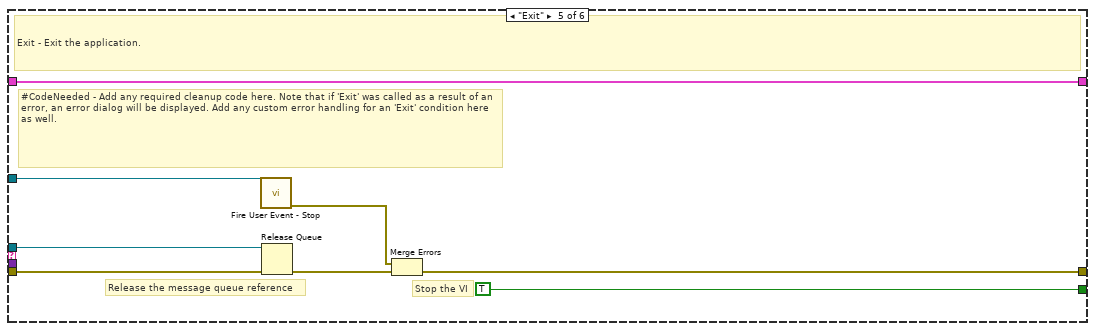
[diagram p14: hidden frame]
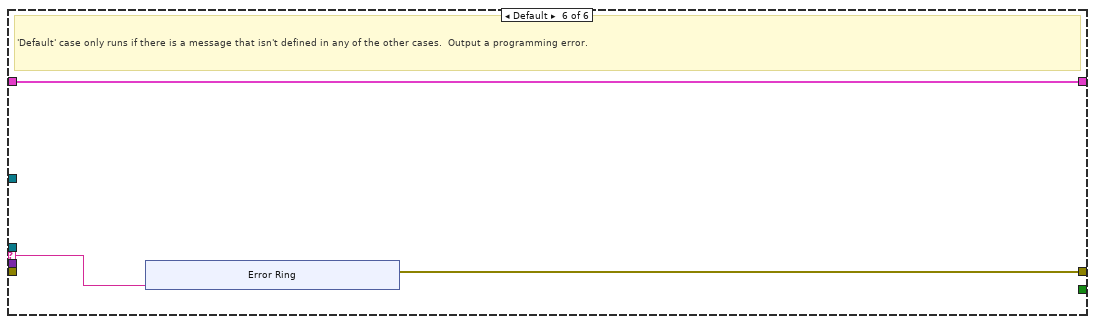
[diagram p15: hidden frame]
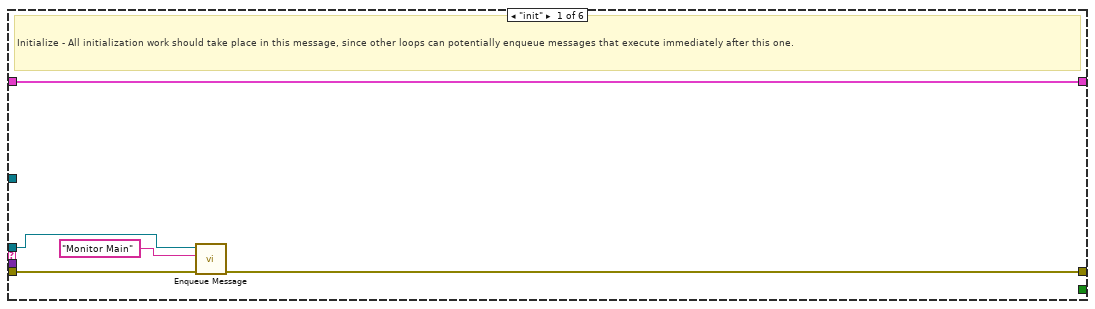
[diagram p16: hidden frame]
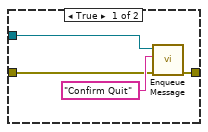
[diagram p17: hidden frame]
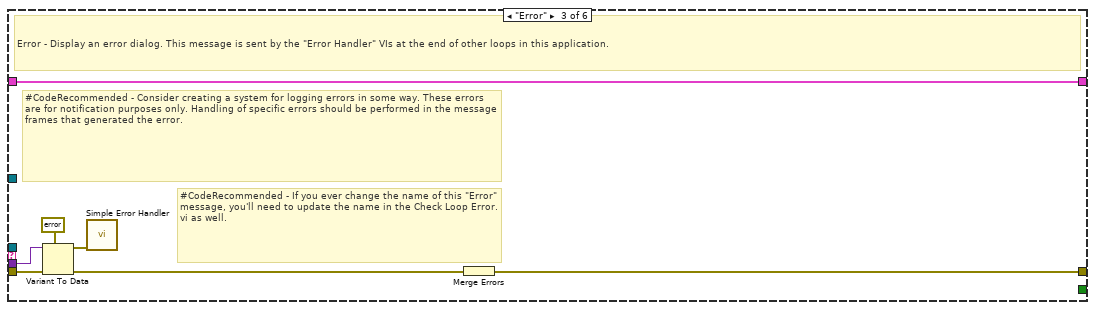
[diagram p18: hidden frame]
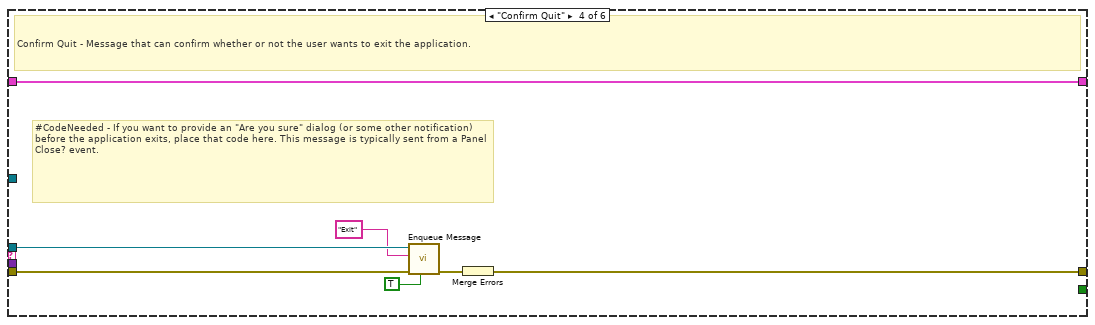
[diagram p19: hidden frame]
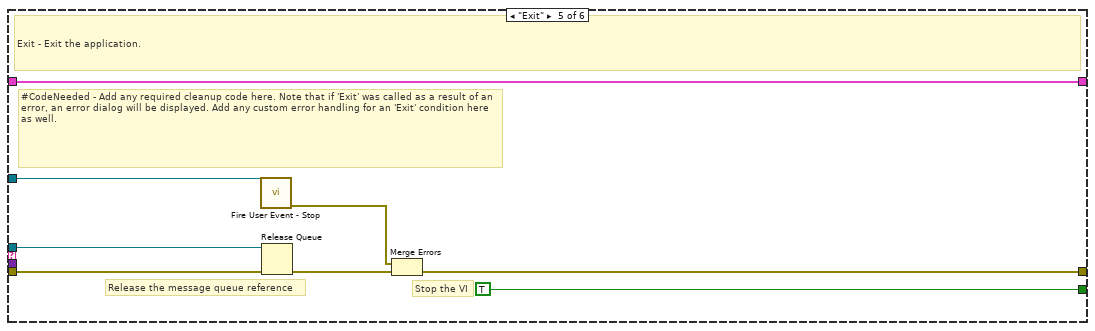
[diagram p20: hidden frame]
diagram:
  n1 = flat-sequence {
    tunnel: [w55] -> w42
    tunnel: T11 {"Main Home Screen"={"GUI"=refnum, "Platform Settings"=refnum, "Configure"=refnum, "Home"=refnum, "EXIT"=refnum, "service 2"=refnum, "MainPage"=refnum, "Analysis"=refnum}, "Platform Settings"={"mm/s  Surge"=refnum, "Update Surge Speed"=refnum, "Drive Error"=refnum, "Disable Axis Jog Soft Limits"=refnum, "mm/s  Sway"=refnum, "Sway and Surge COM Status"=refnum, "Heave COM Status"=refnum, "Enable Platform"=refnum, "Surge Forward Main"=refnum, "Sway Right Main"=refnum, "Sway Left Main"=refnum, "Heave Down Main"=refnum, "Heave Up main"=refnum, "Update Sway Speed"=refnum, "Update Heave Speed"=refnum, "mm/s Heave"=refnum, "mm/sec"=refnum, "mm"=refnum, "Surge Backward Main"=refnum}, "Analysis Screen"={"Analysis Home"=refnum, "Surface Analysis"=refnum, "Imaging"=refnum, "Image Analysis"=refnum, "Post Analysis"=refnum}, "Config Screen"={"Select Load Head"=refnum, "Notes :"=refnum, "FILE"=refnum, "Sample ID :"=refnum, "Operator ID :"=refnum, "Operator Name :"=refnum, "Auto"=refnum}, "Motion Module"={"zNL"=refnum, "NL disp"=refnum, "Rotary Tab"=refnum, "Motion Direction:  3"=refnum, "E.Velocity 2"=refnum, "e.v/ssr 2"=refnum, "Enter Fixed E.Velocity 2"=refnum, "Enter Final SRR 2"=refnum, "Enter initial SRR 2"=refnum, "Enter Fixed SRR 2"=refnum, "Enter the Final E.Velocity (m/s) 2"=refnum, "Enter initial E.Velocity (m/s) 2"=refnum, "Final Speed (RPM) 3"=refnum, "Initial Speed (RPM) 2"=refnum, "Enter the Final Velocity (m/s) 3"=refnum, "Enter initial Velocity (m/s)  3"=refnum, "Ramp Up 2"=refnum, "TEST SELECTION"=refnum, "SPEED SELECTION : "=refnum, "Angular Oscillation Set"=refnum, "Traction"=refnum, "Step Speed"=refnum, "StepTable For Load-Speed"=refnum, "StepTable For Speed"=refnum, "Surge Forward MM"=refnum, "Surge Backward MM"=refnum, "M3 Image"=refnum, "String 39"=refnum, "Sway Left MM"=refnum, "Sway Right MM"=refnum, "Disable Axis Jog Soft Limits"=refnum, "mm"=refnum, "Heave Down MM"=refnum, "Heave Up MM"=refnum, "Wear Track Diameter (mm)"=refnum, "Set WTD"=refnum, "HomeScratch"=refnum, "HomeRot"=refnum, "PlaceModule"=refnum, "Enter the Angle (Deg)"=refnum, "Enter the Frequency (Hz)"=refnum, "Motion Mode:"=refnum, "LR Sway"=refnum, "Rot Hor"=refnum, "Scratch"=refnum, "LR Cam"=refnum, "MMBack"=refnum, "MMNext"=refnum, "Rot Ver"=refnum, "Rotary Module Selection"=refnum, "calculate rotary"=refnum, "SPEED SELECTION : rotary"=refnum, "Import 2"=refnum, "Save 2"=refnum, "File Path :  2"=refnum, "String 45"=refnum, "StepTable For Speed 3"=refnum, "Enter the Speed(mm/sec)"=refnum, "Enter the Speed(RPM)"=refnum}, "Environmental control"={"Humidity  Status  3"=refnum, "Low Temp  Status  2"=refnum, "TK4 status 2"=refnum, "Stage Temperature"=refnum, "Sample Temperature"=refnum, "Humidity (Amb)"=refnum, "Clear List"=refnum, "Add to list"=refnum, "Wear"=refnum, "Vibration"=refnum, "Humidity (Chamber)"=refnum, "Temperature (Chamber)"=refnum, "ECR "=refnum, "Temperature (Amb)"=refnum, "Microphone"=refnum, "Acoustic Emission 3"=refnum, "SNext"=refnum, "APBack"=refnum, "Enter the Temperature (°C):"=refnum, "Enter the Stage \nTemperature (°C):"=refnum, "Enter the Humidity (%Rh):"=refnum, "Low Temp"=refnum, "High Temp"=refnum, "Humidity"=refnum, "Sensors Picked"=refnum}, "About Screen"={"Password"=refnum, "Home Service"=refnum, "Advanced Setting"=refnum, "About Tab"=refnum, "ECR Port:"=refnum, "Ramp Port:"=refnum, "Installation/Replacement completed"=refnum, "Loahead"=refnum, "Heave and Surge COM Port:"=refnum, "Sway COM Port:"=refnum, "Temp Modbus:"=refnum, "Humidity Port:"=refnum, "Edit Gain Constants"=refnum, "Save Gain Constants"=refnum}, "Main Screen"={"Main Screen Tab"=refnum, "Angle and Frequency"=refnum, "Stroke (mm)"=refnum, "Angle (Deg)"=refnum, "Main Speed Tab"=refnum, "MTM MOTOR DISPLAY"=refnum, "Disc Speed (m/sec)"=refnum, "Ball Speed (m/sec)"=refnum, "Disc Speed (RPM)"=refnum, "Ball Speed (RPM)"=refnum, "SPEED TAB"=refnum, "Speed (m/sec)"=refnum, "Set Speed (m/sec)"=refnum, "Speed (RPM)"=refnum, "Set Speed"=refnum, "Time Tab"=refnum, "Time ( HH:MM:SS ) 2"=refnum, "Test Duration"=refnum, "Test Duration 4"=refnum, "TEST CYCLE"=refnum, "TOTAL CYCLES"=refnum, "Set Load (N)"=refnum, "Temp Tabs"=refnum, "Heater"=refnum, "TK4 status"=refnum, "ChamberTemp"=refnum, "SetTmp"=refnum, "Controller  Status"=refnum, "ChamberTemp 2"=refnum, "SetTmp 2"=refnum, "Controller  Status 2"=refnum, "ChamberTemp 3"=refnum, "SetTmp 3"=refnum, "Cooling"=refnum, "Load Communication"=refnum, "Ambient \nTemperature"=refnum, "HumCOMStatus"=refnum, "Ambient\n Humidity"=refnum, "Freq (Hz)"=refnum, "Load En"=refnum, "NLt"=refnum, "zNL 2"=refnum, "Humidity On"=refnum, "humidity disp"=refnum, "Set Humidity"=refnum, "NL disp 2"=refnum, "Humidity On 2"=refnum, "humidity disp 2"=refnum, "Set Humidity 2"=refnum, "NL disp 3"=refnum, "AppLoadSeq scratch"=refnum, "Stop Scratch"=refnum, "ClrLog"=refnum, "Trip Log"=refnum, "STOP"=refnum, "Start Test"=refnum, "Test status"=refnum, "AR Led"=refnum, "Data"=refnum, "Health"=refnum, "Sway COM Status"=refnum, "Heave COM Status"=refnum, "Grp Tab"=refnum, "Sub Graph"=refnum, "SD (mm)"=refnum, "Siliding distance Reset Graph"=refnum, "SDGp"=refnum, "Humidity Reset Graph"=refnum, "HumrGp"=refnum, "Acoustic Emission (mV)"=refnum, "Aqucostic Reset Graph"=refnum, "gACQUOS"=refnum, "ECR RESET"=refnum, "ECR"=refnum, "Temperature Reset"=refnum, "Acoustic Emission (mV) 2"=refnum, "Aqucostic Reset Graph 2"=refnum, "gACQUOS 2"=refnum, "ECR RESET 2"=refnum, "ECR 2"=refnum, "Temperature Reset 2"=refnum, "Temperature (deg c)"=refnum, "Speed Reset Graph"=refnum, "Speed Tab"=refnum, "MTM DISC  SPEED"=refnum, "MTM BALL SPEED"=refnum, "speed mm/sec"=refnum, "Hymidity"=refnum, "Humidity Disable trip"=refnum, "CoF Trip  2"=refnum, "Depth Trip"=refnum, "Weart Deapth"=refnum, "Depth Reset Graph"=refnum, "Weart"=refnum, "Depthz"=refnum, "Depth (µm)"=refnum, "WearGp"=refnum, "NL Trip 2"=refnum, "Load pid"=refnum, "Load Disable Trip"=refnum, "Load Reset Graph"=refnum, "NL Display 4"=refnum, "Main Chart 3"=refnum, "BACK"=refnum, "Depth Trip 2"=refnum, "COF TRIP "=refnum, "Friction Force (N)"=refnum, "FF Reset Graph"=refnum, "FF Disable Trip"=refnum, "FF TRIP"=refnum, "FF MAIN CHART"=refnum, "COF Disable Trip"=refnum, "COF Reset Graph"=refnum, "COF MAIN CHART"=refnum, "FF Tab"=refnum, "Start Test Temp"=refnum}, "Loading"={"Indentation"=refnum, "Reference Sample"=refnum, "Load Cell Communication Slide"=refnum, "com 3"=refnum, "com"=refnum, "DecaForce COM Status"=refnum, "Update"=refnum, "Clear 3"=refnum, "seq"=refnum, "Stribeck table"=refnum, "Stribeck Table  For loading"=refnum, "Loading Mode"=refnum, "Enter the Final Load (N)"=refnum, "Enter the CoF Trip"=refnum, "Enter the Friction Force Trip"=refnum, "Enter the Normal load Trip"=refnum, "Enter the Load  (N)"=refnum, "KiloForce"=refnum, "DecaForce "=refnum, "MicroForce"=refnum, "LHBack"=refnum, "LHNext"=refnum, "Enter the Loading Rate (N/min)"=refnum, "Message"=refnum, "Warning 2"=refnum, "SSP 0.75"=refnum, "SSP 0.5"=refnum, "SSP 0.3"=refnum, "Warning"=refnum, "gui GIF"=refnum, "Communication is established"=refnum, "AppLoad 4"=refnum, "Multipoint"=refnum, "Load Selection"=refnum}, "PID"={"Ramp MulFac"=refnum, "pulses LoadDiffRamp(2..10)"=refnum, "PulseControlRamp(diff<=3N)"=refnum, "SetLoadDeadband(%) Load(0-10N)"=refnum, "PID gains out delay (microForce)"=refnum, "Ramp"=refnum, "Gain 2"=refnum, "pulses LoadDiff(2..10)"=refnum, "pulses LoadDiff(11..50)"=refnum, "PulseControl(diff<=3N)"=refnum, "SetLoadDeadband(%)  2"=refnum, "Dummy Run"=refnum, "Vertical load (N)"=refnum, "AutoTune"=refnum, "Offset 3 "=refnum, "apply load"=refnum, "Offset  3"=refnum, "apply load 2"=refnum, "Enter ByPass Load"=refnum, "reinit 3"=refnum, "output range delay"=refnum, "PID gains out delay"=refnum, "Bypass Load"=refnum, "pulsesSent"=refnum, "pulses "=refnum, "actpid"=refnum, "gFF Rot"=refnum, "pulses LoadDiff(21..1000)"=refnum, "Delay"=refnum, "deadband"=refnum}, "Config Parameters"={"Tab Control 3"=refnum, "Tab Control 19"=refnum, "SAMPLES"=refnum, "Re-initilaize"=refnum, "Filter ON/OFF"=refnum, "TracHomeSurgeOffsetCounts 10MM"=refnum, "TracHomeSwayOffsetCounts 10MM"=refnum, "Acoustic Emission:"=refnum, "Apply Filter (FF)"=refnum, "Filter% 2"=refnum, "Apply Filter (Load)"=refnum, "Filter% "=refnum, "Sway distance (mm)"=refnum, "Surge distance (mm)"=refnum, "DataSavingLoopDelay(ms)"=refnum, "SAVE 2"=refnum, "Enter Distance"=refnum, "Sway Counts:"=refnum, "Distance (mm): 3"=refnum, "Surge Counts:"=refnum, "Distance (mm): 2"=refnum, "Distance (mm):"=refnum, "Heave Counts:"=refnum, "LRMHomeSurgeOffsetCounts"=refnum, "LRMHomeSwayOffsetCounts"=refnum, "TracHomeSurgeOffsetCounts 20MM"=refnum, "TracHomeSwayOffsetCounts 20MM"=refnum, "RotHomeSwayOffsetCounts"=refnum, "RotHomeSurgeOffsetCounts"=refnum, "Heave distance"=refnum, "Zmm"=refnum, "Heave Pulses/mm"=refnum, "Surge Pulses/mm"=refnum, "Sway Pulses/mm"=refnum, "Heave Pitch"=refnum, "Surge Pitch"=refnum, "Sway Pitch"=refnum, "Heave PPR"=refnum, "Surge PPR"=refnum, "Sway PPR"=refnum, "Tab Control 5"=refnum, "Tab Control 14"=refnum, "Tab Control 26"=refnum, "AE"=refnum, "Heave Loop Delay"=refnum, "Heave PID Speed"=refnum, "Surge Jog Speed"=refnum, "Heave Jog Speed"=refnum}, "Loading Com Port"={"ClearAll"=refnum, "Mz(Nm)"=refnum, "My(Nm)"=refnum, "Mx(Nm)"=refnum, "Save Dwell"=refnum, "Mx "=refnum, "My "=refnum, "Mz"=refnum, "Fx(N)"=refnum, "Fy(N)"=refnum, "Fz(N)"=refnum, "ZeroAll"=refnum, "Acq Delay (ms)"=refnum, "Burst Delay (ms)"=refnum, "model"=refnum, "SN"=refnum, "FFx(N)"=refnum, "Sensor IP"=refnum, "Port"=refnum, "FFy(N)"=refnum, "Load(N)"=refnum, "delete Handle"=refnum, "Create Handle"=refnum, "ft_data"=refnum, "ft_range"=refnum, "ft_data 2"=refnum, "stop 6"=refnum, "running_flag"=refnum, "ft_udp_handle"=refnum, "get-data-return"=refnum, "get-range-return"=refnum, "zero-return"=refnum, "filter-return"=refnum, "initial-return"=refnum, "deleteHandle-result"=refnum, "Load Cell Temp"=refnum}, "Heave AND Surge"={"SURGE POSE"=refnum, "error out Read"=refnum, "HEAVE POSE"=refnum, "State"=refnum, "Homed"=refnum, "Sequence ID"=refnum, "error out Write"=refnum, "faultCode"=refnum, "Ack ID"=refnum, "SPEED"=refnum, "Distance"=refnum, "Mode Command"=refnum, "Heave and Surge Read"=refnum, "Read Heave Temp"=refnum, "Spare 15"=refnum, "Spare 14"=refnum, "Spare 13"=refnum, "Spare 12"=refnum, "Spare 11"=refnum, "Spare 10"=refnum, "Spare 9"=refnum, "Spare 8"=refnum, "Spare 7"=refnum, "Spare 6"=refnum, "Spare 5"=refnum, "Spare 4"=refnum, "Spare 2"=refnum, "Spare 1"=refnum, "Node Id"=refnum, "Spare 3"=refnum, "SPARE 4"=refnum, "SPARE 3"=refnum, "SPARE 2"=refnum, "SPARE 1"=refnum, "fwMajor"=refnum, "fwMinor"=refnum, "Manual Write"=refnum, "Heave and Surge Write"=refnum}, "New PID LOGIC"={"Fine Tune Zone"=refnum, "PID SDelay"=refnum, "Max_pos_limit"=refnum, "Min_pos_limit"=refnum, "i_limit"=refnum, "pct_scale"=refnum, "Deadband"=refnum, "Kd"=refnum, "Ki"=refnum, "Kp"=refnum, "Current Position"=refnum, "Set Load"=refnum, "Current Load"=refnum, "Pulse delta"=refnum, "Init Step"=refnum, "Max Step Linit"=refnum}, "SWAY "={"fwMajor"=refnum, "Homed"=refnum, "Rotary POSE"=refnum, "State"=refnum, "SWAY POSE"=refnum, "Ack ID"=refnum, "faultCode"=refnum, "Node Id"=refnum, "fwMinor"=refnum, "Spare 6"=refnum, "Spare 5"=refnum, "Spare 4"=refnum, "Spare 3"=refnum, "Spare 2"=refnum, "Spare 1"=refnum, "Spare 7"=refnum, "SPARE  5"=refnum, "error out Write  SWAY "=refnum, "error out Read SWAY "=refnum, "Manual Write SWAY "=refnum, "SWAY WRITE"=refnum, "SPARE  4"=refnum, "SPARE  3"=refnum, "SPARE 2"=refnum, "SPARE 1"=refnum, "Spare 15"=refnum, "Spare 14"=refnum, "Spare 13"=refnum, "Spare 12"=refnum, "Spare 11"=refnum, "Spare 9"=refnum, "Spare 8"=refnum, "SPEED"=refnum, "Distance"=refnum, "Mode Command"=refnum, "Sequence ID"=refnum, "SWAY READ"=refnum, "Spare 10"=refnum, "Read SWAY Temp"=refnum}} ("Data Cluster") -> [w54]
    tunnel: w42 -> [w84]
    tunnel: [w64] -> w41
    tunnel: w41 -> [w91]
    tunnel: [w85] -> w40
    tunnel: w40 -> [w100]
    tunnel: [w99] -> w39
    tunnel: w39 -> [w136]
    tunnel: [w135] -> w37
    tunnel: w37 -> [w197]
    tunnel: [w196] -> w36
    tunnel: w36 -> [w224]
    tunnel: [w223] -> w35
    tunnel: w35 -> [w240]
    tunnel: [w239] -> w34
    tunnel: w34 -> [w345]
    tunnel: [w344] -> w9
    tunnel: w9 -> [w375]
    tunnel: [w374] -> w8
    tunnel: w8 -> [w425]
    tunnel: [w424] -> w7
    tunnel: w7 -> [w462]
    tunnel: [w461] -> w6
    tunnel: w6 -> [w502]
    tunnel: [w501] -> w3
    tunnel: w3 -> [w520]
    tunnel: [w519] -> w2
    tunnel: [w560] -> w14
    tunnel: w2 -> [w561]
    frame #0 {
      n2 = control-ref of="GUI"() -> (w63:refnum<vi>)
      n3 = control-ref of="MainPage"() -> (w57:refnum<vi>)
      n4 = control-ref of="Platform Settings"() -> (w62:refnum<vi>)
      n5 = control-ref of="Configure"() -> (w61:refnum<vi>)
      n6 = control-ref of="Home"() -> (w60:refnum<vi>)
      n7 = control-ref of="EXIT"() -> (w59:refnum<vi>)
      n8 = control-ref of="service 2"() -> (w58:refnum<vi>)
      n9 = control-ref of="Analysis"() -> (w56:refnum<vi>)
      n10 = Bundle By Name(cluster=w54, "Main Home Screen.GUI"=w63, "Main Home Screen.Platform Settings"=w62, "Main Home Screen.Configure"=w61, "Main Home Screen.Home"=w60, "Main Home Screen.EXIT"=w59, "Main Home Screen.service 2"=w58, "Main Home Screen.MainPage"=w57, "Main Home Screen.Analysis"=w56) -> (w55:T11)
    }
    frame #1 {
      n11 = control-ref of="Sway Right Main"() -> (w74:refnum<vi>)
      n12 = control-ref of="Sway Left Main"() -> (w73:refnum<vi>)
      n13 = control-ref of="Heave Down Main"() -> (w72:refnum<vi>)
      n14 = control-ref of="Heave Up main"() -> (w71:refnum<vi>)
      n15 = control-ref of="Update Sway Speed"() -> (w70:refnum<vi>)
      n16 = control-ref of="Update Heave Speed"() -> (w69:refnum<vi>)
      n17 = control-ref of="Surge Backward Main"() -> (w65:refnum<vi>)
      n18 = control-ref of="Update Surge Speed"() -> (w82:refnum<vi>)
      n19 = control-ref of="Disable Axis Jog Soft Limits"() -> (w80:refnum<vi>)
      n20 = control-ref of="Sway and Surge COM Status"() -> (w78:refnum<vi>)
      n21 = control-ref of="Heave COM Status"() -> (w77:refnum<vi>)
      n22 = control-ref of="Enable Platform"() -> (w76:refnum<vi>)
      n23 = control-ref of="Surge Forward Main"() -> (w75:refnum<vi>)
      n24 = control-ref of="mm/s Heave"() -> (w68:refnum<vi>)
      n25 = control-ref of="mm/sec"() -> (w67:refnum<vi>)
      n26 = control-ref of="mm"() -> (w66:refnum<vi>)
      n27 = control-ref of="mm/s  Surge"() -> (w83:refnum<vi>)
      n28 = control-ref of="mm/s  Sway"() -> (w79:refnum<vi>)
      n29 = control-ref of="Drive Error"() -> (w81:refnum<vi>)
      n30 = Bundle By Name(cluster=w84, "Platform Settings.mm/s  Surge"=w83, "Platform Settings.Update Surge Speed"=w82, "Platform Settings.Drive Error"=w81, "Platform Settings.Disable Axis Jog Soft Limits"=w80, "Platform Settings.mm/s  Sway"=w79, "Platform Settings.Sway and Surge COM Status"=w78, "Platform Settings.Heave COM Status"=w77, "Platform Settings.Enable Platform"=w76, "Platform Settings.Surge Forward Main"=w75, "Platform Settings.Sway Right Main"=w74, "Platform Settings.Sway Left Main"=w73, "Platform Settings.Heave Down Main"=w72, "Platform Settings.Heave Up main"=w71, "Platform Settings.Update Sway Speed"=w70, "Platform Settings.Update Heave Speed"=w69, "Platform Settings.mm/s Heave"=w68, "Platform Settings.mm/sec"=w67, "Platform Settings.mm"=w66, "Platform Settings.Surge Backward Main"=w65) -> (w64:T11)
    }
    frame #2 {
      n31 = control-ref of="Analysis Home"() -> (w90:refnum<vi>)
      n32 = control-ref of="Surface Analysis"() -> (w89:refnum<vi>)
      n33 = control-ref of="Imaging"() -> (w88:refnum<vi>)
      n34 = control-ref of="Image Analysis"() -> (w87:refnum<vi>)
      n35 = control-ref of="Post Analysis"() -> (w86:refnum<vi>)
      n36 = Bundle By Name(cluster=w91, "Analysis Screen.Analysis Home"=w90, "Analysis Screen.Surface Analysis"=w89, "Analysis Screen.Imaging"=w88, "Analysis Screen.Image Analysis"=w87, "Analysis Screen.Post Analysis"=w86) -> (w85:T11)
    }
    frame #3 {
      n37 = control-ref of="Select Load Head"() -> (w98:refnum<vi>)
      n38 = control-ref of="Auto"() -> (w92:refnum<vi>)
      n39 = control-ref of="Notes :"() -> (w97:refnum<vi>)
      n40 = control-ref of="FILE"() -> (w96:refnum<vi>)
      n41 = control-ref of="Sample ID :"() -> (w95:refnum<vi>)
      n42 = control-ref of="Operator ID :"() -> (w94:refnum<vi>)
      n43 = control-ref of="Operator Name :"() -> (w93:refnum<vi>)
      n44 = Bundle By Name(cluster=w100, "Config Screen.Select Load Head"=w98, "Config Screen.Notes :"=w97, "Config Screen.FILE"=w96, "Config Screen.Sample ID :"=w95, "Config Screen.Operator ID :"=w94, "Config Screen.Operator Name :"=w93, "Config Screen.Auto"=w92) -> (w99:T11)
    }
    frame #4 {
      n45 = control-ref of="Warning"() -> (w128:refnum<vi>)
      n46 = control-ref of="gui GIF"() -> (w127:refnum<vi>)
      n47 = control-ref of="Load Selection"() -> (w101:refnum<vi>)
      n48 = control-ref of="Warning 2"() -> (w132:refnum<vi>)
      n49 = control-ref of="SSP 0.75"() -> (w131:refnum<vi>)
      n50 = control-ref of="SSP 0.5"() -> (w130:refnum<vi>)
      n51 = control-ref of="SSP 0.3"() -> (w129:refnum<vi>)
      n52 = control-ref of="Communication is established"() -> (w126:refnum<vi>)
      n53 = control-ref of="AppLoad 4"() -> (w125:refnum<vi>)
      n54 = control-ref of="Multipoint"() -> (w124:refnum<vi>)
      n55 = control-ref of="com 3"() -> (w120:refnum<vi>)
      n56 = control-ref of="com"() -> (w119:refnum<vi>)
      n57 = control-ref of="DecaForce COM Status"() -> (w118:refnum<vi>)
      n58 = control-ref of="Update"() -> (w117:refnum<vi>)
      n59 = control-ref of="Clear 3"() -> (w116:refnum<vi>)
      n60 = control-ref of="seq"() -> (w115:refnum<vi>)
      n61 = control-ref of="Stribeck table"() -> (w114:refnum<vi>)
      n62 = control-ref of="KiloForce"() -> (w106:refnum<vi>)
      n63 = control-ref of="DecaForce"() -> (w105:refnum<vi>)
      n64 = control-ref of="MicroForce"() -> (w104:refnum<vi>)
      n65 = control-ref of="LHBack"() -> (w103:refnum<vi>)
      n66 = control-ref of="LHNext"() -> (w102:refnum<vi>)
      n67 = control-ref of="Enter the Loading Rate (N/min)"() -> (w134:refnum<vi>)
      n68 = control-ref of="Enter the Final Load (N)"() -> (w111:refnum<vi>)
      n69 = control-ref of="Enter the CoF Trip"() -> (w110:refnum<vi>)
      n70 = control-ref of="Enter the Friction Force Trip"() -> (w109:refnum<vi>)
      n71 = control-ref of="Enter the Normal load Trip"() -> (w108:refnum<vi>)
      n72 = control-ref of="Enter the Load  (N)"() -> (w107:refnum<vi>)
      n73 = control-ref of="Message"() -> (w133:refnum<vi>)
      n74 = control-ref of="Indentation"() -> (w123:refnum<vi>)
      n75 = control-ref of="Stribeck Table  For loading"() -> (w113:refnum<vi>)
      n76 = control-ref of="Reference Sample"() -> (w122:refnum<vi>)
      n77 = control-ref of="Load Cell Communication Slide"() -> (w121:refnum<vi>)
      n78 = control-ref of="Loading Mode"() -> (w112:refnum<vi>)
      n79 = Bundle By Name(cluster=w136, "Loading.Enter the Loading Rate (N/min)"=w134, "Loading.Message"=w133, "Loading.Warning 2"=w132, "Loading.SSP 0.75"=w131, "Loading.SSP 0.5"=w130, "Loading.SSP 0.3"=w129, "Loading.Warning"=w128, "Loading.gui GIF"=w127, "Loading.Communication is established"=w126, "Loading.AppLoad 4"=w125, "Loading.Multipoint"=w124, "Loading.Indentation"=w123, "Loading.Reference Sample"=w122, "Loading.Load Cell Communication Slide"=w121, "Loading.com 3"=w120, "Loading.com"=w119, "Loading.DecaForce COM Status"=w118, "Loading.Update"=w117, "Loading.Clear 3"=w116, "Loading.seq"=w115, "Loading.Stribeck table"=w114, "Loading.Stribeck Table  For loading"=w113, "Loading.Loading Mode"=w112, "Loading.Enter the Final Load (N)"=w111, "Loading.Enter the CoF Trip"=w110, "Loading.Enter the Friction Force Trip"=w109, "Loading.Enter the Normal load Trip"=w108, "Loading.Enter the Load  (N)"=w107, "Loading.KiloForce"=w106, "Loading.DecaForce"=w105, "Loading.MicroForce"=w104, "Loading.LHBack"=w103, "Loading.LHNext"=w102, "Loading.Load Selection"=w101) -> (w135:T11)
    }
    frame #5 {
      n80 = control-ref of="TEST SELECTION"() -> (w178:refnum<vi>)
      n81 = control-ref of="SPEED SELECTION :"() -> (w177:refnum<vi>)
      n82 = control-ref of="SPEED SELECTION : rotary"() -> (w144:refnum<vi>)
      n83 = control-ref of="Rotary Tab"() -> (w193:refnum<vi>)
      n84 = control-ref of="e.v/ssr 2"() -> (w190:refnum<vi>)
      n85 = control-ref of="Step Speed"() -> (w174:refnum<vi>)
      n86 = control-ref of="M3 Image"() -> (w169:refnum<vi>)
      n87 = control-ref of="Rotary Module Selection"() -> (w146:refnum<vi>)
      n88 = control-ref of="zNL"() -> (w195:refnum<vi>)
      n89 = control-ref of="E.Velocity 2"() -> (w191:refnum<vi>)
      n90 = control-ref of="Ramp Up 2"() -> (w179:refnum<vi>)
      n91 = control-ref of="Angular Oscillation Set"() -> (w176:refnum<vi>)
      n92 = control-ref of="Traction"() -> (w175:refnum<vi>)
      n93 = control-ref of="Surge Forward MM"() -> (w171:refnum<vi>)
      n94 = control-ref of="Surge Backward MM"() -> (w170:refnum<vi>)
      n95 = control-ref of="Sway Left MM"() -> (w167:refnum<vi>)
      n96 = control-ref of="Sway Right MM"() -> (w166:refnum<vi>)
      n97 = control-ref of="Disable Axis Jog Soft Limits"() -> (w165:refnum<vi>)
      n98 = control-ref of="Heave Down MM"() -> (w163:refnum<vi>)
      n99 = control-ref of="Heave Up MM"() -> (w162:refnum<vi>)
      n100 = control-ref of="Set WTD"() -> (w160:refnum<vi>)
      n101 = control-ref of="HomeScratch"() -> (w159:refnum<vi>)
      n102 = control-ref of="HomeRot"() -> (w158:refnum<vi>)
      n103 = control-ref of="PlaceModule"() -> (w157:refnum<vi>)
      n104 = control-ref of="LR Sway"() -> (w153:refnum<vi>)
      n105 = control-ref of="Rot Hor"() -> (w152:refnum<vi>)
      n106 = control-ref of="Scratch"() -> (w151:refnum<vi>)
      n107 = control-ref of="LR Cam"() -> (w150:refnum<vi>)
      n108 = control-ref of="MMBack"() -> (w149:refnum<vi>)
      n109 = control-ref of="MMNext"() -> (w148:refnum<vi>)
      n110 = control-ref of="Rot Ver"() -> (w147:refnum<vi>)
      n111 = control-ref of="calculate rotary"() -> (w145:refnum<vi>)
      n112 = control-ref of="Import 2"() -> (w143:refnum<vi>)
      n113 = control-ref of="Save 2"() -> (w142:refnum<vi>)
      n114 = control-ref of="NL disp"() -> (w194:refnum<vi>)
      n115 = control-ref of="Enter Fixed E.Velocity 2"() -> (w189:refnum<vi>)
      n116 = control-ref of="Enter Final SRR 2"() -> (w188:refnum<vi>)
      n117 = control-ref of="Enter initial SRR 2"() -> (w187:refnum<vi>)
      n118 = control-ref of="Enter Fixed SRR 2"() -> (w186:refnum<vi>)
      n119 = control-ref of="Enter the Final E.Velocity (m/s) 2"() -> (w185:refnum<vi>)
      n120 = control-ref of="Enter initial E.Velocity (m/s) 2"() -> (w184:refnum<vi>)
      n121 = control-ref of="Final Speed (RPM) 3"() -> (w183:refnum<vi>)
      n122 = control-ref of="Initial Speed (RPM) 2"() -> (w182:refnum<vi>)
      n123 = control-ref of="Enter the Final Velocity (m/s) 3"() -> (w181:refnum<vi>)
      n124 = control-ref of="Enter initial Velocity (m/s)  3"() -> (w180:refnum<vi>)
      n125 = control-ref of="mm"() -> (w164:refnum<vi>)
      n126 = control-ref of="Wear Track Diameter (mm)"() -> (w161:refnum<vi>)
      n127 = control-ref of="Enter the Angle (Deg)"() -> (w156:refnum<vi>)
      n128 = control-ref of="Enter the Frequency (Hz)"() -> (w155:refnum<vi>)
      n129 = control-ref of="Enter the Speed(mm/sec)"() -> (w138:refnum<vi>)
      n130 = control-ref of="Enter the Speed(RPM)"() -> (w137:refnum<vi>)
      n131 = control-ref of="String 39"() -> (w168:refnum<vi>)
      n132 = control-ref of="String 45"() -> (w140:refnum<vi>)
      n133 = control-ref of="StepTable For Load-Speed"() -> (w173:refnum<vi>)
      n134 = control-ref of="StepTable For Speed"() -> (w172:refnum<vi>)
      n135 = control-ref of="Motion Direction:  3"() -> (w192:refnum<vi>)
      n136 = control-ref of="Motion Mode:"() -> (w154:refnum<vi>)
      n137 = control-ref of="StepTable For Speed 3"() -> (w139:refnum<vi>)
      n138 = control-ref of="File Path :  2"() -> (w141:refnum<vi>)
      n139 = Bundle By Name(cluster=w197, "Motion Module.zNL"=w195, "Motion Module.NL disp"=w194, "Motion Module.Rotary Tab"=w193, "Motion Module.Motion Direction:  3"=w192, "Motion Module.E.Velocity 2"=w191, "Motion Module.e.v/ssr 2"=w190, "Motion Module.Enter Fixed E.Velocity 2"=w189, "Motion Module.Enter Final SRR 2"=w188, "Motion Module.Enter initial SRR 2"=w187, "Motion Module.Enter Fixed SRR 2"=w186, "Motion Module.Enter the Final E.Velocity (m/s) 2"=w185, "Motion Module.Enter initial E.Velocity (m/s) 2"=w184, "Motion Module.Final Speed (RPM) 3"=w183, "Motion Module.Initial Speed (RPM) 2"=w182, "Motion Module.Enter the Final Velocity (m/s) 3"=w181, "Motion Module.Enter initial Velocity (m/s)  3"=w180, "Motion Module.Ramp Up 2"=w179, "Motion Module.TEST SELECTION"=w178, "Motion Module.SPEED SELECTION :"=w177, "Motion Module.Angular Oscillation Set"=w176, "Motion Module.Traction"=w175, "Motion Module.Step Speed"=w174, "Motion Module.StepTable For Load-Speed"=w173, "Motion Module.StepTable For Speed"=w172, "Motion Module.Surge Forward MM"=w171, "Motion Module.Surge Backward MM"=w170, "Motion Module.M3 Image"=w169, "Motion Module.String 39"=w168, "Motion Module.Sway Left MM"=w167, "Motion Module.Sway Right MM"=w166, "Motion Module.Disable Axis Jog Soft Limits"=w165, "Motion Module.mm"=w164, "Motion Module.Heave Down MM"=w163, "Motion Module.Heave Up MM"=w162, "Motion Module.Wear Track Diameter (mm)"=w161, "Motion Module.Set WTD"=w160, "Motion Module.HomeScratch"=w159, "Motion Module.HomeRot"=w158, "Motion Module.PlaceModule"=w157, "Motion Module.Enter the Angle (Deg)"=w156, "Motion Module.Enter the Frequency (Hz)"=w155, "Motion Module.Motion Mode:"=w154, "Motion Module.LR Sway"=w153, "Motion Module.Rot Hor"=w152, "Motion Module.Scratch"=w151, "Motion Module.LR Cam"=w150, "Motion Module.MMBack"=w149, "Motion Module.MMNext"=w148, "Motion Module.Rot Ver"=w147, "Motion Module.Rotary Module Selection"=w146, "Motion Module.calculate rotary"=w145, "Motion Module.SPEED SELECTION : rotary"=w144, "Motion Module.Import 2"=w143, "Motion Module.Save 2"=w142, "Motion Module.File Path :  2"=w141, "Motion Module.String 45"=w140, "Motion Module.StepTable For Speed 3"=w139, "Motion Module.Enter the Speed(mm/sec)"=w138, "Motion Module.Enter the Speed(RPM)"=w137) -> (w196:T11)
    }
    frame #6 {
      n140 = control-ref of="Add to list"() -> (w215:refnum<vi>)
      n141 = control-ref of="Wear"() -> (w214:refnum<vi>)
      n142 = control-ref of="Vibration"() -> (w213:refnum<vi>)
      n143 = control-ref of="Humidity (Chamber)"() -> (w212:refnum<vi>)
      n144 = control-ref of="Temperature (Chamber)"() -> (w211:refnum<vi>)
      n145 = control-ref of="ECR"() -> (w210:refnum<vi>)
      n146 = control-ref of="Temperature (Amb)"() -> (w209:refnum<vi>)
      n147 = control-ref of="Microphone"() -> (w208:refnum<vi>)
      n148 = control-ref of="Acoustic Emission 3"() -> (w207:refnum<vi>)
      n149 = control-ref of="SNext"() -> (w206:refnum<vi>)
      n150 = control-ref of="APBack"() -> (w205:refnum<vi>)
      n151 = control-ref of="Low Temp"() -> (w201:refnum<vi>)
      n152 = control-ref of="High Temp"() -> (w200:refnum<vi>)
      n153 = control-ref of="Humidity"() -> (w199:refnum<vi>)
      n154 = control-ref of="Humidity  Status  3"() -> (w222:refnum<vi>)
      n155 = control-ref of="Low Temp  Status  2"() -> (w221:refnum<vi>)
      n156 = control-ref of="TK4 status 2"() -> (w220:refnum<vi>)
      n157 = control-ref of="Humidity (Amb)"() -> (w217:refnum<vi>)
      n158 = control-ref of="Clear List"() -> (w216:refnum<vi>)
      n159 = control-ref of="Enter the Temperature (°C):"() -> (w204:refnum<vi>)
      n160 = control-ref of="Enter the Stage \nTemperature (°C):"() -> (w203:refnum<vi>)
      n161 = control-ref of="Enter the Humidity (%Rh):"() -> (w202:refnum<vi>)
      n162 = control-ref of="Sensors Picked"() -> (w198:refnum<vi>)
      n163 = control-ref of="Stage Temperature"() -> (w219:refnum<vi>)
      n164 = control-ref of="Sample Temperature"() -> (w218:refnum<vi>)
      n165 = Bundle By Name(cluster=w224, "Environmental control.Humidity  Status  3"=w222, "Environmental control.Low Temp  Status  2"=w221, "Environmental control.TK4 status 2"=w220, "Environmental control.Stage Temperature"=w219, "Environmental control.Sample Temperature"=w218, "Environmental control.Humidity (Amb)"=w217, "Environmental control.Clear List"=w216, "Environmental control.Add to list"=w215, "Environmental control.Wear"=w214, "Environmental control.Vibration"=w213, "Environmental control.Humidity (Chamber)"=w212, "Environmental control.Temperature (Chamber)"=w211, "Environmental control.ECR"=w210, "Environmental control.Temperature (Amb)"=w209, "Environmental control.Microphone"=w208, "Environmental control.Acoustic Emission 3"=w207, "Environmental control.SNext"=w206, "Environmental control.APBack"=w205, "Environmental control.Enter the Temperature (°C):"=w204, "Environmental control.Enter the Stage \nTemperature (°C):"=w203, "Environmental control.Enter the Humidity (%Rh):"=w202, "Environmental control.Low Temp"=w201, "Environmental control.High Temp"=w200, "Environmental control.Humidity"=w199, "Environmental control.Sensors Picked"=w198) -> (w223:T11)
    }
    frame #7 {
      n166 = control-ref of="ECR Port:"() -> (w234:refnum<vi>)
      n167 = control-ref of="Ramp Port:"() -> (w233:refnum<vi>)
      n168 = control-ref of="Heave and Surge COM Port:"() -> (w230:refnum<vi>)
      n169 = control-ref of="Sway COM Port:"() -> (w229:refnum<vi>)
      n170 = control-ref of="Temp Modbus:"() -> (w228:refnum<vi>)
      n171 = control-ref of="Humidity Port:"() -> (w227:refnum<vi>)
      n172 = control-ref of="About Tab"() -> (w235:refnum<vi>)
      n173 = control-ref of="Home Service"() -> (w237:refnum<vi>)
      n174 = control-ref of="Advanced Setting"() -> (w236:refnum<vi>)
      n175 = control-ref of="Installation/Replacement completed"() -> (w232:refnum<vi>)
      n176 = control-ref of="Loahead"() -> (w231:refnum<vi>)
      n177 = control-ref of="Edit Gain Constants"() -> (w226:refnum<vi>)
      n178 = control-ref of="Save Gain Constants"() -> (w225:refnum<vi>)
      n179 = control-ref of="Password"() -> (w238:refnum<vi>)
      n180 = Bundle By Name(cluster=w240, "About Screen.Password"=w238, "About Screen.Home Service"=w237, "About Screen.Advanced Setting"=w236, "About Screen.About Tab"=w235, "About Screen.ECR Port:"=w234, "About Screen.Ramp Port:"=w233, "About Screen.Installation/Replacement completed"=w232, "About Screen.Loahead"=w231, "About Screen.Heave and Surge COM Port:"=w230, "About Screen.Sway COM Port:"=w229, "About Screen.Temp Modbus:"=w228, "About Screen.Humidity Port:"=w227, "About Screen.Edit Gain Constants"=w226, "About Screen.Save Gain Constants"=w225) -> (w239:T11)
    }
    frame #8 {
      n181 = control-ref of="SDGp"() -> (w284:refnum<vi>)
      n182 = control-ref of="HumrGp"() -> (w282:refnum<vi>)
      n183 = control-ref of="gACQUOS"() -> (w279:refnum<vi>)
      n184 = control-ref of="ECR"() -> (w277:refnum<vi>)
      n185 = control-ref of="Temperature (deg c)"() -> (w275:refnum<vi>)
      n186 = control-ref of="MTM DISC  SPEED"() -> (w272:refnum<vi>)
      n187 = control-ref of="MTM BALL SPEED"() -> (w271:refnum<vi>)
      n188 = control-ref of="speed mm/sec"() -> (w270:refnum<vi>)
      n189 = control-ref of="WearGp"() -> (w260:refnum<vi>)
      n190 = control-ref of="Main Chart 3"() -> (w254:refnum<vi>)
      n191 = control-ref of="FF MAIN CHART"() -> (w246:refnum<vi>)
      n192 = control-ref of="COF MAIN CHART"() -> (w243:refnum<vi>)
      n193 = control-ref of="Main Screen Tab"() -> (w343:refnum<vi>)
      n194 = control-ref of="Angle and Frequency"() -> (w342:refnum<vi>)
      n195 = control-ref of="Main Speed Tab"() -> (w339:refnum<vi>)
      n196 = control-ref of="MTM MOTOR DISPLAY"() -> (w338:refnum<vi>)
      n197 = control-ref of="SPEED TAB"() -> (w333:refnum<vi>)
      n198 = control-ref of="Time Tab"() -> (w328:refnum<vi>)
      n199 = control-ref of="Temp Tabs"() -> (w321:refnum<vi>)
      n200 = control-ref of="Grp Tab"() -> (w288:refnum<vi>)
      n201 = control-ref of="Sub Graph"() -> (w287:refnum<vi>)
      n202 = control-ref of="Speed Tab"() -> (w273:refnum<vi>)
      n203 = control-ref of="FF Tab"() -> (w242:refnum<vi>)
      n204 = control-ref of="Heater"() -> (w320:refnum<vi>)
      n205 = control-ref of="TK4 status"() -> (w319:refnum<vi>)
      n206 = control-ref of="Controller  Status"() -> (w316:refnum<vi>)
      n207 = control-ref of="Cooling"() -> (w313:refnum<vi>)
      n208 = control-ref of="Load Communication"() -> (w312:refnum<vi>)
      n209 = control-ref of="HumCOMStatus"() -> (w310:refnum<vi>)
      n210 = control-ref of="Load En"() -> (w307:refnum<vi>)
      n211 = control-ref of="NLt"() -> (w306:refnum<vi>)
      n212 = control-ref of="zNL 2"() -> (w305:refnum<vi>)
      n213 = control-ref of="Humidity On"() -> (w304:refnum<vi>)
      n214 = control-ref of="AppLoadSeq scratch"() -> (w300:refnum<vi>)
      n215 = control-ref of="Stop Scratch"() -> (w299:refnum<vi>)
      n216 = control-ref of="ClrLog"() -> (w298:refnum<vi>)
      n217 = control-ref of="STOP"() -> (w296:refnum<vi>)
      n218 = control-ref of="Start Test"() -> (w295:refnum<vi>)
      n219 = control-ref of="Test status"() -> (w294:refnum<vi>)
      n220 = control-ref of="AR Led"() -> (w293:refnum<vi>)
      n221 = control-ref of="Data"() -> (w292:refnum<vi>)
      n222 = control-ref of="Health"() -> (w291:refnum<vi>)
      n223 = control-ref of="Sway COM Status"() -> (w290:refnum<vi>)
      n224 = control-ref of="Heave COM Status"() -> (w289:refnum<vi>)
      n225 = control-ref of="Siliding distance Reset Graph"() -> (w285:refnum<vi>)
      n226 = control-ref of="Humidity Reset Graph"() -> (w283:refnum<vi>)
      n227 = control-ref of="Aqucostic Reset Graph"() -> (w280:refnum<vi>)
      n228 = control-ref of="ECR RESET"() -> (w278:refnum<vi>)
      n229 = control-ref of="Temperature Reset"() -> (w276:refnum<vi>)
      n230 = control-ref of="Speed Reset Graph"() -> (w274:refnum<vi>)
      n231 = control-ref of="Hymidity"() -> (w269:refnum<vi>)
      n232 = control-ref of="Humidity Disable trip"() -> (w268:refnum<vi>)
      n233 = control-ref of="Weart Deapth"() -> (w265:refnum<vi>)
      n234 = control-ref of="Depth Reset Graph"() -> (w264:refnum<vi>)
      n235 = control-ref of="Weart"() -> (w263:refnum<vi>)
      n236 = control-ref of="Depthz"() -> (w262:refnum<vi>)
      n237 = control-ref of="Load pid"() -> (w258:refnum<vi>)
      n238 = control-ref of="Load Disable Trip"() -> (w257:refnum<vi>)
      n239 = control-ref of="Load Reset Graph"() -> (w256:refnum<vi>)
      n240 = control-ref of="BACK"() -> (w253:refnum<vi>)
      n241 = control-ref of="FF Reset Graph"() -> (w249:refnum<vi>)
      n242 = control-ref of="FF Disable Trip"() -> (w248:refnum<vi>)
      n243 = control-ref of="COF Disable Trip"() -> (w245:refnum<vi>)
      n244 = control-ref of="COF Reset Graph"() -> (w244:refnum<vi>)
      n245 = control-ref of="Start Test Temp"() -> (w241:refnum<vi>)
      n246 = control-ref of="Depth Trip"() -> (w252:refnum<vi>)
      n247 = control-ref of="Stroke (mm)"() -> (w341:refnum<vi>)
      n248 = control-ref of="Angle (Deg)"() -> (w340:refnum<vi>)
      n249 = control-ref of="Disc Speed (m/sec)"() -> (w337:refnum<vi>)
      n250 = control-ref of="Ball Speed (m/sec)"() -> (w336:refnum<vi>)
      n251 = control-ref of="Disc Speed (RPM)"() -> (w335:refnum<vi>)
      n252 = control-ref of="Ball Speed (RPM)"() -> (w334:refnum<vi>)
      n253 = control-ref of="Speed (m/sec)"() -> (w332:refnum<vi>)
      n254 = control-ref of="Set Speed (m/sec)"() -> (w331:refnum<vi>)
      n255 = control-ref of="Speed (RPM)"() -> (w330:refnum<vi>)
      n256 = control-ref of="Set Speed"() -> (w329:refnum<vi>)
      n257 = control-ref of="Time ( HH:MM:SS ) 2"() -> (w327:refnum<vi>)
      n258 = control-ref of="Test Duration"() -> (w326:refnum<vi>)
      n259 = control-ref of="Test Duration 4"() -> (w325:refnum<vi>)
      n260 = control-ref of="TEST CYCLE"() -> (w324:refnum<vi>)
      n261 = control-ref of="TOTAL CYCLES"() -> (w323:refnum<vi>)
      n262 = control-ref of="Set Load (N)"() -> (w322:refnum<vi>)
      n263 = control-ref of="ChamberTemp"() -> (w318:refnum<vi>)
      n264 = control-ref of="SetTmp"() -> (w317:refnum<vi>)
      n265 = control-ref of="ChamberTemp"() -> (w315:refnum<vi>)
      n266 = control-ref of="SetTmp"() -> (w314:refnum<vi>)
      n267 = control-ref of="Ambient \nTemperature"() -> (w311:refnum<vi>)
      n268 = control-ref of="Ambient\n Humidity"() -> (w309:refnum<vi>)
      n269 = control-ref of="Freq (Hz)"() -> (w308:refnum<vi>)
      n270 = control-ref of="humidity disp"() -> (w303:refnum<vi>)
      n271 = control-ref of="Set Humidity"() -> (w302:refnum<vi>)
      n272 = control-ref of="NL disp 2"() -> (w301:refnum<vi>)
      n273 = control-ref of="SD (mm)"() -> (w286:refnum<vi>)
      n274 = control-ref of="Acoustic Emission (mV)"() -> (w281:refnum<vi>)
      n275 = control-ref of="CoF Trip  2"() -> (w267:refnum<vi>)
      n276 = control-ref of="Depth Trip"() -> (w266:refnum<vi>)
      n277 = control-ref of="Depth (µm)"() -> (w261:refnum<vi>)
      n278 = control-ref of="NL Trip 2"() -> (w259:refnum<vi>)
      n279 = control-ref of="NL Display 4"() -> (w255:refnum<vi>)
      n280 = control-ref of="COF TRIP"() -> (w251:refnum<vi>)
      n281 = control-ref of="Friction Force (N)"() -> (w250:refnum<vi>)
      n282 = control-ref of="FF TRIP"() -> (w247:refnum<vi>)
      n283 = control-ref of="Trip Log"() -> (w297:refnum<vi>)
      n284 = Bundle By Name(cluster=w345, "Main Screen.Main Screen Tab"=w343, "Main Screen.Angle and Frequency"=w342, "Main Screen.Stroke (mm)"=w341, "Main Screen.Angle (Deg)"=w340, "Main Screen.Main Speed Tab"=w339, "Main Screen.MTM MOTOR DISPLAY"=w338, "Main Screen.Disc Speed (m/sec)"=w337, "Main Screen.Ball Speed (m/sec)"=w336, "Main Screen.Disc Speed (RPM)"=w335, "Main Screen.Ball Speed (RPM)"=w334, "Main Screen.SPEED TAB"=w333, "Main Screen.Speed (m/sec)"=w332, "Main Screen.Set Speed (m/sec)"=w331, "Main Screen.Speed (RPM)"=w330, "Main Screen.Set Speed"=w329, "Main Screen.Time Tab"=w328, "Main Screen.Time ( HH:MM:SS ) 2"=w327, "Main Screen.Test Duration"=w326, "Main Screen.Test Duration 4"=w325, "Main Screen.TEST CYCLE"=w324, "Main Screen.TOTAL CYCLES"=w323, "Main Screen.Set Load (N)"=w322, "Main Screen.Temp Tabs"=w321, "Main Screen.Heater"=w320, "Main Screen.TK4 status"=w319, "Main Screen.ChamberTemp"=w318, "Main Screen.SetTmp"=w317, "Main Screen.Controller  Status"=w316, "Main Screen.ChamberTemp 2"=w315, "Main Screen.SetTmp 2"=w314, "Main Screen.Cooling"=w313, "Main Screen.Load Communication"=w312, "Main Screen.Ambient \nTemperature"=w311, "Main Screen.HumCOMStatus"=w310, "Main Screen.Ambient\n Humidity"=w309, "Main Screen.Freq (Hz)"=w308, "Main Screen.Load En"=w307, "Main Screen.NLt"=w306, "Main Screen.zNL 2"=w305, "Main Screen.Humidity On"=w304, "Main Screen.humidity disp"=w303, "Main Screen.Set Humidity"=w302, "Main Screen.NL disp 2"=w301, "Main Screen.AppLoadSeq scratch"=w300, "Main Screen.Stop Scratch"=w299, "Main Screen.ClrLog"=w298, "Main Screen.Trip Log"=w297, "Main Screen.STOP"=w296, "Main Screen.Start Test"=w295, "Main Screen.Test status"=w294, "Main Screen.AR Led"=w293, "Main Screen.Data"=w292, "Main Screen.Health"=w291, "Main Screen.Sway COM Status"=w290, "Main Screen.Heave COM Status"=w289, "Main Screen.Grp Tab"=w288, "Main Screen.Sub Graph"=w287, "Main Screen.SD (mm)"=w286, "Main Screen.Siliding distance Reset Graph"=w285, "Main Screen.SDGp"=w284, "Main Screen.Humidity Reset Graph"=w283, "Main Screen.HumrGp"=w282, "Main Screen.Acoustic Emission (mV)"=w281, "Main Screen.Aqucostic Reset Graph"=w280, "Main Screen.gACQUOS"=w279, "Main Screen.ECR RESET"=w278, "Main Screen.ECR"=w277, "Main Screen.Temperature Reset"=w276, "Main Screen.Temperature (deg c)"=w275, "Main Screen.Speed Reset Graph"=w274, "Main Screen.Speed Tab"=w273, "Main Screen.MTM DISC  SPEED"=w272, "Main Screen.MTM BALL SPEED"=w271, "Main Screen.speed mm/sec"=w270, "Main Screen.Hymidity"=w269, "Main Screen.Humidity Disable trip"=w268, "Main Screen.CoF Trip  2"=w267, "Main Screen.Depth Trip"=w266, "Main Screen.Weart Deapth"=w265, "Main Screen.Depth Reset Graph"=w264, "Main Screen.Weart"=w263, "Main Screen.Depthz"=w262, "Main Screen.Depth (µm)"=w261, "Main Screen.WearGp"=w260, "Main Screen.NL Trip 2"=w259, "Main Screen.Load pid"=w258, "Main Screen.Load Disable Trip"=w257, "Main Screen.Load Reset Graph"=w256, "Main Screen.NL Display 4"=w255, "Main Screen.Main Chart 3"=w254, "Main Screen.BACK"=w253, "Main Screen.Depth Trip 2"=w252, "Main Screen.COF TRIP"=w251, "Main Screen.Friction Force (N)"=w250, "Main Screen.FF Reset Graph"=w249, "Main Screen.FF Disable Trip"=w248, "Main Screen.FF TRIP"=w247, "Main Screen.FF MAIN CHART"=w246, "Main Screen.COF Disable Trip"=w245, "Main Screen.COF Reset Graph"=w244, "Main Screen.COF MAIN CHART"=w243, "Main Screen.FF Tab"=w242, "Main Screen.Start Test Temp"=w241) -> (w344:T11)
    }
    frame #9 {
      n285 = control-ref of="gFF Rot 7"() -> (w349:refnum<vi>)
      n286 = control-ref of="Ramp"() -> (w368:refnum<vi>)
      n287 = control-ref of="Dummy Run"() -> (w362:refnum<vi>)
      n288 = control-ref of="AutoTune"() -> (w360:refnum<vi>)
      n289 = control-ref of="apply load"() -> (w358:refnum<vi>)
      n290 = control-ref of="reinit 3"() -> (w356:refnum<vi>)
      n291 = control-ref of="Bypass Load"() -> (w353:refnum<vi>)
      n292 = control-ref of="PID gains out delay (microForce)"() -> (w369:refnum<vi>)
      n293 = control-ref of="output range delay"() -> (w355:refnum<vi>)
      n294 = control-ref of="PID gains out delay"() -> (w354:refnum<vi>)
      n295 = control-ref of="Ramp MulFac"() -> (w373:refnum<vi>)
      n296 = control-ref of="pulses LoadDiffRamp(2..10)"() -> (w372:refnum<vi>)
      n297 = control-ref of="PulseControlRamp(diff<=3N)"() -> (w371:refnum<vi>)
      n298 = control-ref of="SetLoadDeadband(%) Load(0-10N)"() -> (w370:refnum<vi>)
      n299 = control-ref of="Gain 2"() -> (w367:refnum<vi>)
      n300 = control-ref of="pulses LoadDiff(2..10)"() -> (w366:refnum<vi>)
      n301 = control-ref of="pulses LoadDiff(11..50)"() -> (w365:refnum<vi>)
      n302 = control-ref of="PulseControl(diff<=3N)"() -> (w364:refnum<vi>)
      n303 = control-ref of="SetLoadDeadband(%)  2"() -> (w363:refnum<vi>)
      n304 = control-ref of="Vertical load (N)"() -> (w361:refnum<vi>)
      n305 = control-ref of="Offset  3"() -> (w359:refnum<vi>)
      n306 = control-ref of="Enter ByPass Load"() -> (w357:refnum<vi>)
      n307 = control-ref of="pulsesSent"() -> (w352:refnum<vi>)
      n308 = control-ref of="pulses"() -> (w351:refnum<vi>)
      n309 = control-ref of="actpid"() -> (w350:refnum<vi>)
      n310 = control-ref of="pulses LoadDiff(21..1000)"() -> (w348:refnum<vi>)
      n311 = control-ref of="Delay"() -> (w347:refnum<vi>)
      n312 = control-ref of="deadband"() -> (w346:refnum<vi>)
      n313 = Bundle By Name(cluster=w375, "PID.Ramp MulFac"=w373, "PID.pulses LoadDiffRamp(2..10)"=w372, "PID.PulseControlRamp(diff<=3N)"=w371, "PID.SetLoadDeadband(%) Load(0-10N)"=w370, "PID.PID gains out delay (microForce)"=w369, "PID.Ramp"=w368, "PID.Gain 2"=w367, "PID.pulses LoadDiff(2..10)"=w366, "PID.pulses LoadDiff(11..50)"=w365, "PID.PulseControl(diff<=3N)"=w364, "PID.SetLoadDeadband(%)  2"=w363, "PID.Dummy Run"=w362, "PID.Vertical load (N)"=w361, "PID.AutoTune"=w360, "PID.Offset 3"=w359, "PID.apply load"=w358, "PID.Enter ByPass Load"=w357, "PID.reinit 3"=w356, "PID.output range delay"=w355, "PID.PID gains out delay"=w354, "PID.Bypass Load"=w353, "PID.pulsesSent"=w352, "PID.pulses"=w351, "PID.actpid"=w350, "PID.gFF Rot"=w349, "PID.pulses LoadDiff(21..1000)"=w348, "PID.Delay"=w347, "PID.deadband"=w346) -> (w374:T11)
    }
    frame #10 {
      n314 = control-ref of="Tab Control 3"() -> (w423:refnum<vi>)
      n315 = control-ref of="Tab Control 19"() -> (w422:refnum<vi>)
      n316 = control-ref of="Tab Control 5"() -> (w383:refnum<vi>)
      n317 = control-ref of="Tab Control 14"() -> (w382:refnum<vi>)
      n318 = control-ref of="Tab Control 26"() -> (w381:refnum<vi>)
      n319 = control-ref of="Re-initilaize"() -> (w420:refnum<vi>)
      n320 = control-ref of="Filter ON/OFF"() -> (w419:refnum<vi>)
      n321 = control-ref of="Apply Filter (FF)"() -> (w415:refnum<vi>)
      n322 = control-ref of="Apply Filter (Load)"() -> (w413:refnum<vi>)
      n323 = control-ref of="SAVE  2"() -> (w408:refnum<vi>)
      n324 = control-ref of="Enter Distance"() -> (w407:refnum<vi>)
      n325 = control-ref of="AE"() -> (w380:refnum<vi>)
      n326 = control-ref of="Heave Loop Delay"() -> (w379:refnum<vi>)
      n327 = control-ref of="Heave PID Speed"() -> (w378:refnum<vi>)
      n328 = control-ref of="Surge Jog Speed"() -> (w377:refnum<vi>)
      n329 = control-ref of="Heave Jog Speed"() -> (w376:refnum<vi>)
      n330 = control-ref of="SAMPLES"() -> (w421:refnum<vi>)
      n331 = control-ref of="TracHomeSurgeOffsetCounts 10MM"() -> (w418:refnum<vi>)
      n332 = control-ref of="TracHomeSwayOffsetCounts 10MM"() -> (w417:refnum<vi>)
      n333 = control-ref of="Acoustic Emission:"() -> (w416:refnum<vi>)
      n334 = control-ref of="Filter% 2"() -> (w414:refnum<vi>)
      n335 = control-ref of="Filter%"() -> (w412:refnum<vi>)
      n336 = control-ref of="Sway distance (mm)"() -> (w411:refnum<vi>)
      n337 = control-ref of="Surge distance (mm)"() -> (w410:refnum<vi>)
      n338 = control-ref of="DataSavingLoopDelay(ms)"() -> (w409:refnum<vi>)
      n339 = control-ref of="Sway Counts:"() -> (w406:refnum<vi>)
      n340 = control-ref of="Distance (mm): 3"() -> (w405:refnum<vi>)
      n341 = control-ref of="Surge Counts:"() -> (w404:refnum<vi>)
      n342 = control-ref of="Distance (mm): 2"() -> (w403:refnum<vi>)
      n343 = control-ref of="Distance (mm):"() -> (w402:refnum<vi>)
      n344 = control-ref of="Heave Counts:"() -> (w401:refnum<vi>)
      n345 = control-ref of="LRMHomeSurgeOffsetCounts"() -> (w400:refnum<vi>)
      n346 = control-ref of="LRMHomeSwayOffsetCounts"() -> (w399:refnum<vi>)
      n347 = control-ref of="TracHomeSurgeOffsetCounts 20MM"() -> (w398:refnum<vi>)
      n348 = control-ref of="TracHomeSwayOffsetCounts 20MM"() -> (w397:refnum<vi>)
      n349 = control-ref of="RotHomeSwayOffsetCounts"() -> (w396:refnum<vi>)
      n350 = control-ref of="RotHomeSurgeOffsetCounts"() -> (w395:refnum<vi>)
      n351 = control-ref of="Heave distance"() -> (w394:refnum<vi>)
      n352 = control-ref of="Zmm"() -> (w393:refnum<vi>)
      n353 = control-ref of="Heave Pulses/mm"() -> (w392:refnum<vi>)
      n354 = control-ref of="Surge Pulses/mm"() -> (w391:refnum<vi>)
      n355 = control-ref of="Sway Pulses/mm"() -> (w390:refnum<vi>)
      n356 = control-ref of="Heave Pitch"() -> (w389:refnum<vi>)
      n357 = control-ref of="Surge Pitch"() -> (w388:refnum<vi>)
      n358 = control-ref of="Sway Pitch"() -> (w387:refnum<vi>)
      n359 = control-ref of="Heave PPR"() -> (w386:refnum<vi>)
      n360 = control-ref of="Surge PPR"() -> (w385:refnum<vi>)
      n361 = control-ref of="Sway PPR"() -> (w384:refnum<vi>)
      n362 = Bundle By Name(cluster=w425, "Config Parameters.Tab Control 3"=w423, "Config Parameters.Tab Control 19"=w422, "Config Parameters.SAMPLES"=w421, "Config Parameters.Re-initilaize"=w420, "Config Parameters.Filter ON/OFF"=w419, "Config Parameters.TracHomeSurgeOffsetCounts 10MM"=w418, "Config Parameters.TracHomeSwayOffsetCounts 10MM"=w417, "Config Parameters.Acoustic Emission:"=w416, "Config Parameters.Apply Filter (FF)"=w415, "Config Parameters.Filter% 2"=w414, "Config Parameters.Apply Filter (Load)"=w413, "Config Parameters.Filter%"=w412, "Config Parameters.Sway distance (mm)"=w411, "Config Parameters.Surge distance (mm)"=w410, "Config Parameters.DataSavingLoopDelay(ms)"=w409, "Config Parameters.SAVE 2"=w408, "Config Parameters.Enter Distance"=w407, "Config Parameters.Sway Counts:"=w406, "Config Parameters.Distance (mm): 3"=w405, "Config Parameters.Surge Counts:"=w404, "Config Parameters.Distance (mm): 2"=w403, "Config Parameters.Distance (mm):"=w402, "Config Parameters.Heave Counts:"=w401, "Config Parameters.LRMHomeSurgeOffsetCounts"=w400, "Config Parameters.LRMHomeSwayOffsetCounts"=w399, "Config Parameters.TracHomeSurgeOffsetCounts 20MM"=w398, "Config Parameters.TracHomeSwayOffsetCounts 20MM"=w397, "Config Parameters.RotHomeSwayOffsetCounts"=w396, "Config Parameters.RotHomeSurgeOffsetCounts"=w395, "Config Parameters.Heave distance"=w394, "Config Parameters.Zmm"=w393, "Config Parameters.Heave Pulses/mm"=w392, "Config Parameters.Surge Pulses/mm"=w391, "Config Parameters.Sway Pulses/mm"=w390, "Config Parameters.Heave Pitch"=w389, "Config Parameters.Surge Pitch"=w388, "Config Parameters.Sway Pitch"=w387, "Config Parameters.Heave PPR"=w386, "Config Parameters.Surge PPR"=w385, "Config Parameters.Sway PPR"=w384, "Config Parameters.Tab Control 5"=w383, "Config Parameters.Tab Control 14"=w382, "Config Parameters.Tab Control 26"=w381, "Config Parameters.AE"=w380, "Config Parameters.Heave Loop Delay"=w379, "Config Parameters.Heave PID Speed"=w378, "Config Parameters.Surge Jog Speed"=w377, "Config Parameters.Heave Jog Speed"=w376) -> (w424:T11)
    }
    frame #11 {
      n363 = control-ref of="Mx"() -> (w455:refnum<vi>)
      n364 = control-ref of="My"() -> (w454:refnum<vi>)
      n365 = control-ref of="Mz"() -> (w453:refnum<vi>)
      n366 = control-ref of="Fx(N)"() -> (w452:refnum<vi>)
      n367 = control-ref of="Fy(N)"() -> (w451:refnum<vi>)
      n368 = control-ref of="Fz(N)"() -> (w450:refnum<vi>)
      n369 = control-ref of="Load Cell Temp"() -> (w426:refnum<vi>)
      n370 = control-ref of="ClearAll"() -> (w460:refnum<vi>)
      n371 = control-ref of="ZeroAll"() -> (w449:refnum<vi>)
      n372 = control-ref of="delete Handle"() -> (w439:refnum<vi>)
      n373 = control-ref of="Create Handle"() -> (w438:refnum<vi>)
      n374 = control-ref of="stop 6"() -> (w435:refnum<vi>)
      n375 = control-ref of="running_flag"() -> (w434:refnum<vi>)
      n376 = control-ref of="Save Dwell"() -> (w456:refnum<vi>)
      n377 = control-ref of="Acq Delay (ms)"() -> (w448:refnum<vi>)
      n378 = control-ref of="Burst Delay (ms)"() -> (w447:refnum<vi>)
      n379 = control-ref of="SN"() -> (w445:refnum<vi>)
      n380 = control-ref of="Port"() -> (w442:refnum<vi>)
      n381 = control-ref of="ft_udp_handle"() -> (w433:refnum<vi>)
      n382 = control-ref of="get-data-return"() -> (w432:refnum<vi>)
      n383 = control-ref of="get-range-return"() -> (w431:refnum<vi>)
      n384 = control-ref of="zero-return"() -> (w430:refnum<vi>)
      n385 = control-ref of="filter-return"() -> (w429:refnum<vi>)
      n386 = control-ref of="initial-return"() -> (w428:refnum<vi>)
      n387 = control-ref of="deleteHandle-result"() -> (w427:refnum<vi>)
      n388 = control-ref of="model"() -> (w446:refnum<vi>)
      n389 = control-ref of="Sensor IP"() -> (w443:refnum<vi>)
      n390 = control-ref of="Mz(Nm)"() -> (w459:refnum<vi>)
      n391 = control-ref of="My(Nm)"() -> (w458:refnum<vi>)
      n392 = control-ref of="Mx(Nm)"() -> (w457:refnum<vi>)
      n393 = control-ref of="FFx(N)"() -> (w444:refnum<vi>)
      n394 = control-ref of="FFy(N)"() -> (w441:refnum<vi>)
      n395 = control-ref of="Load(N)"() -> (w440:refnum<vi>)
      n396 = control-ref of="ft_data"() -> (w437:refnum<vi>)
      n397 = control-ref of="ft_range"() -> (w436:refnum<vi>)
      n398 = Bundle By Name(cluster=w462, "Loading Com Port.ClearAll"=w460, "Loading Com Port.Mz(Nm)"=w459, "Loading Com Port.My(Nm)"=w458, "Loading Com Port.Mx(Nm)"=w457, "Loading Com Port.Save Dwell"=w456, "Loading Com Port.Mx"=w455, "Loading Com Port.My"=w454, "Loading Com Port.Mz"=w453, "Loading Com Port.Fx(N)"=w452, "Loading Com Port.Fy(N)"=w451, "Loading Com Port.Fz(N)"=w450, "Loading Com Port.ZeroAll"=w449, "Loading Com Port.Acq Delay (ms)"=w448, "Loading Com Port.Burst Delay (ms)"=w447, "Loading Com Port.model"=w446, "Loading Com Port.SN"=w445, "Loading Com Port.FFx(N)"=w444, "Loading Com Port.Sensor IP"=w443, "Loading Com Port.Port"=w442, "Loading Com Port.FFy(N)"=w441, "Loading Com Port.Load(N)"=w440, "Loading Com Port.delete Handle"=w439, "Loading Com Port.Create Handle"=w438, "Loading Com Port.ft_data"=w437, "Loading Com Port.ft_range"=w436, "Loading Com Port.stop 6"=w435, "Loading Com Port.running_flag"=w434, "Loading Com Port.ft_udp_handle"=w433, "Loading Com Port.get-data-return"=w432, "Loading Com Port.get-range-return"=w431, "Loading Com Port.zero-return"=w430, "Loading Com Port.filter-return"=w429, "Loading Com Port.initial-return"=w428, "Loading Com Port.deleteHandle-result"=w427, "Loading Com Port.Load Cell Temp"=w426) -> (w461:T11)
    }
    frame #12 {
      n399 = control-ref of="Manual Write Heave & Surge"() -> (w464:refnum<vi>)
      n400 = control-ref of="Read Heave Temp"() -> (w487:refnum<vi>)
      n401 = control-ref of="error out Read"() -> (w499:refnum<vi>)
      n402 = control-ref of="error out Write"() -> (w494:refnum<vi>)
      n403 = control-ref of="SURGE POSE"() -> (w500:refnum<vi>)
      n404 = control-ref of="HEAVE POSE"() -> (w498:refnum<vi>)
      n405 = control-ref of="State"() -> (w497:refnum<vi>)
      n406 = control-ref of="Homed"() -> (w496:refnum<vi>)
      n407 = control-ref of="Sequence ID"() -> (w495:refnum<vi>)
      n408 = control-ref of="faultCode"() -> (w493:refnum<vi>)
      n409 = control-ref of="Ack ID"() -> (w492:refnum<vi>)
      n410 = control-ref of="SPEED"() -> (w491:refnum<vi>)
      n411 = control-ref of="Distance"() -> (w490:refnum<vi>)
      n412 = control-ref of="Mode Command"() -> (w489:refnum<vi>)
      n413 = control-ref of="SPARE 2"() -> (w486:refnum<vi>)
      n414 = control-ref of="SPARE 1"() -> (w485:refnum<vi>)
      n415 = control-ref of="Spare 15"() -> (w484:refnum<vi>)
      n416 = control-ref of="Spare 14"() -> (w483:refnum<vi>)
      n417 = control-ref of="Spare 13"() -> (w482:refnum<vi>)
      n418 = control-ref of="Spare 12"() -> (w481:refnum<vi>)
      n419 = control-ref of="Spare 11"() -> (w480:refnum<vi>)
      n420 = control-ref of="Spare 10"() -> (w479:refnum<vi>)
      n421 = control-ref of="Spare 9"() -> (w478:refnum<vi>)
      n422 = control-ref of="Spare 8"() -> (w477:refnum<vi>)
      n423 = control-ref of="Spare 7"() -> (w476:refnum<vi>)
      n424 = control-ref of="Spare 6"() -> (w475:refnum<vi>)
      n425 = control-ref of="Spare 5"() -> (w474:refnum<vi>)
      n426 = control-ref of="Spare 4"() -> (w473:refnum<vi>)
      n427 = control-ref of="Spare 3"() -> (w472:refnum<vi>)
      n428 = control-ref of="Spare 2"() -> (w471:refnum<vi>)
      n429 = control-ref of="Spare 1"() -> (w470:refnum<vi>)
      n430 = control-ref of="Node Id"() -> (w469:refnum<vi>)
      n431 = control-ref of="SPARE 3"() -> (w468:refnum<vi>)
      n432 = control-ref of="SPARE 4"() -> (w467:refnum<vi>)
      n433 = control-ref of="fwMajor"() -> (w466:refnum<vi>)
      n434 = control-ref of="fwMinor"() -> (w465:refnum<vi>)
      n435 = control-ref of="Heave and Surge Write"() -> (w463:refnum<vi>)
      n436 = control-ref of="Heave and Surge Read"() -> (w488:refnum<vi>)
      n437 = Bundle By Name(cluster=w502, "Heave AND Surge.SURGE POSE"=w500, "Heave AND Surge.error out Read"=w499, "Heave AND Surge.HEAVE POSE"=w498, "Heave AND Surge.State"=w497, "Heave AND Surge.Homed"=w496, "Heave AND Surge.Sequence ID"=w495, "Heave AND Surge.error out Write"=w494, "Heave AND Surge.faultCode"=w493, "Heave AND Surge.Ack ID"=w492, "Heave AND Surge.SPEED"=w491, "Heave AND Surge.Distance"=w490, "Heave AND Surge.Mode Command"=w489, "Heave AND Surge.Heave and Surge Read"=w488, "Heave AND Surge.Read Heave Temp"=w487, "Heave AND Surge.SPARE 2"=w486, "Heave AND Surge.SPARE 1"=w485, "Heave AND Surge.Spare 15"=w484, "Heave AND Surge.Spare 14"=w483, "Heave AND Surge.Spare 13"=w482, "Heave AND Surge.Spare 12"=w481, "Heave AND Surge.Spare 11"=w480, "Heave AND Surge.Spare 10"=w479, "Heave AND Surge.Spare 9"=w478, "Heave AND Surge.Spare 8"=w477, "Heave AND Surge.Spare 7"=w476, "Heave AND Surge.Spare 6"=w475, "Heave AND Surge.Spare 5"=w474, "Heave AND Surge.Spare 4"=w473, "Heave AND Surge.Spare 3"=w472, "Heave AND Surge.Spare 2"=w471, "Heave AND Surge.Spare 1"=w470, "Heave AND Surge.Node Id"=w469, "Heave AND Surge.SPARE 3"=w468, "Heave AND Surge.SPARE 4"=w467, "Heave AND Surge.fwMajor"=w466, "Heave AND Surge.fwMinor"=w465, "Heave AND Surge.Manual Write"=w464, "Heave AND Surge.Heave and Surge Write"=w463) -> (w501:T11)
    }
    frame #13 {
      n438 = control-ref of="Fine Tune Zone"() -> (w518:refnum<vi>)
      n439 = control-ref of="PID Delay (sec)"() -> (w517:refnum<vi>)
      n440 = control-ref of="Max_pos_limit"() -> (w516:refnum<vi>)
      n441 = control-ref of="Min_pos_limit"() -> (w515:refnum<vi>)
      n442 = control-ref of="i_limit"() -> (w514:refnum<vi>)
      n443 = control-ref of="pct_scale"() -> (w505:refnum<vi>)
      n444 = control-ref of="Deadband"() -> (w513:refnum<vi>)
      n445 = control-ref of="Kd"() -> (w512:refnum<vi>)
      n446 = control-ref of="Ki"() -> (w511:refnum<vi>)
      n447 = control-ref of="Kp"() -> (w510:refnum<vi>)
      n448 = control-ref of="Current Position"() -> (w509:refnum<vi>)
      n449 = control-ref of="Set Load"() -> (w508:refnum<vi>)
      n450 = control-ref of="Current Load"() -> (w507:refnum<vi>)
      n451 = control-ref of="Pulse delta"() -> (w506:refnum<vi>)
      n452 = control-ref of="Init Step"() -> (w504:refnum<vi>)
      n453 = control-ref of="Max Step Linit"() -> (w503:refnum<vi>)
      n454 = Bundle By Name(cluster=w520, "New PID LOGIC.Fine Tune Zone"=w518, "New PID LOGIC.PID SDelay"=w517, "New PID LOGIC.Max_pos_limit"=w516, "New PID LOGIC.Min_pos_limit"=w515, "New PID LOGIC.i_limit"=w514, "New PID LOGIC.pct_scale"=w505, "New PID LOGIC.Deadband"=w513, "New PID LOGIC.Kd"=w512, "New PID LOGIC.Ki"=w511, "New PID LOGIC.Kp"=w510, "New PID LOGIC.Current Position"=w509, "New PID LOGIC.Set Load"=w508, "New PID LOGIC.Current Load"=w507, "New PID LOGIC.Pulse delta"=w506, "New PID LOGIC.Init Step"=w504, "New PID LOGIC.Max Step Linit"=w503) -> (w519:T11)
    }
    frame #14 {
      n455 = control-ref of="Manual Write SWAY"() -> (w540:refnum<vi>)
      n456 = control-ref of="Read SWAY Temp"() -> (w521:refnum<vi>)
      n457 = control-ref of="error out Write  SWAY"() -> (w542:refnum<vi>)
      n458 = control-ref of="error out Read SWAY"() -> (w541:refnum<vi>)
      n459 = control-ref of="fwMajor"() -> (w559:refnum<vi>)
      n460 = control-ref of="Homed"() -> (w558:refnum<vi>)
      n461 = control-ref of="Rotary POSE"() -> (w557:refnum<vi>)
      n462 = control-ref of="State"() -> (w556:refnum<vi>)
      n463 = control-ref of="SWAY POSE"() -> (w555:refnum<vi>)
      n464 = control-ref of="Ack ID"() -> (w554:refnum<vi>)
      n465 = control-ref of="faultCode"() -> (w553:refnum<vi>)
      n466 = control-ref of="Node Id"() -> (w552:refnum<vi>)
      n467 = control-ref of="fwMinor"() -> (w551:refnum<vi>)
      n468 = control-ref of="Spare 6"() -> (w550:refnum<vi>)
      n469 = control-ref of="Spare 5"() -> (w549:refnum<vi>)
      n470 = control-ref of="Spare 4"() -> (w548:refnum<vi>)
      n471 = control-ref of="Spare 3"() -> (w547:refnum<vi>)
      n472 = control-ref of="Spare 2"() -> (w546:refnum<vi>)
      n473 = control-ref of="Spare 1"() -> (w545:refnum<vi>)
      n474 = control-ref of="Spare 7"() -> (w544:refnum<vi>)
      n475 = control-ref of="SPARE  5"() -> (w543:refnum<vi>)
      n476 = control-ref of="SPARE  4"() -> (w538:refnum<vi>)
      n477 = control-ref of="SPARE  3"() -> (w537:refnum<vi>)
      n478 = control-ref of="SPARE 2"() -> (w536:refnum<vi>)
      n479 = control-ref of="SPARE 1"() -> (w535:refnum<vi>)
      n480 = control-ref of="Spare 15"() -> (w534:refnum<vi>)
      n481 = control-ref of="Spare 14"() -> (w533:refnum<vi>)
      n482 = control-ref of="Spare 13"() -> (w532:refnum<vi>)
      n483 = control-ref of="Spare 12"() -> (w531:refnum<vi>)
      n484 = control-ref of="Spare 11"() -> (w530:refnum<vi>)
      n485 = control-ref of="Spare 9"() -> (w529:refnum<vi>)
      n486 = control-ref of="Spare 8"() -> (w528:refnum<vi>)
      n487 = control-ref of="SPEED"() -> (w527:refnum<vi>)
      n488 = control-ref of="Distance"() -> (w526:refnum<vi>)
      n489 = control-ref of="Mode Command"() -> (w525:refnum<vi>)
      n490 = control-ref of="Sequence ID"() -> (w524:refnum<vi>)
      n491 = control-ref of="Spare 10"() -> (w522:refnum<vi>)
      n492 = control-ref of="SWAY WRITE"() -> (w539:refnum<vi>)
      n493 = control-ref of="SWAY READ"() -> (w523:refnum<vi>)
      n494 = Bundle By Name(cluster=w561, "SWAY.fwMajor"=w559, "SWAY.Homed"=w558, "SWAY.Rotary POSE"=w557, "SWAY.State"=w556, "SWAY.SWAY POSE"=w555, "SWAY.Ack ID"=w554, "SWAY.faultCode"=w553, "SWAY.Node Id"=w552, "SWAY.fwMinor"=w551, "SWAY.Spare 6"=w550, "SWAY.Spare 5"=w549, "SWAY.Spare 4"=w548, "SWAY.Spare 3"=w547, "SWAY.Spare 2"=w546, "SWAY.Spare 1"=w545, "SWAY.Spare 7"=w544, "SWAY.SPARE  5"=w543, "SWAY.error out Write  SWAY"=w542, "SWAY.error out Read SWAY"=w541, "SWAY.Manual Write SWAY"=w540, "SWAY.SWAY WRITE"=w539, "SWAY.SPARE  4"=w538, "SWAY.SPARE  3"=w537, "SWAY.SPARE 2"=w536, "SWAY.SPARE 1"=w535, "SWAY.Spare 15"=w534, "SWAY.Spare 14"=w533, "SWAY.Spare 13"=w532, "SWAY.Spare 12"=w531, "SWAY.Spare 11"=w530, "SWAY.Spare 9"=w529, "SWAY.Spare 8"=w528, "SWAY.SPEED"=w527, "SWAY.Distance"=w526, "SWAY.Mode Command"=w525, "SWAY.Sequence ID"=w524, "SWAY.SWAY READ"=w523, "SWAY.Spare 10"=w522, "SWAY.Read SWAY Temp"=w521) -> (w560:T11)
    }
  }
  n495 = call <userlib>:"Fit VI window to Largest Dec.vi"() -> ("error out"=w30:errorcluster, "dup VI Ref"=w27:refnum<vi>)  [unwired: 6 in]
  n496 = invoke on="Invoke Node" class="VI" method="FP.Run-Time Position.Maximized"(reference=w27, error in=w30) -> (error out=w29:errorcluster)  [unwired: 2 in, 3 out]
  n497 = call <vilib>:"Clear Errors.vi"("error in (no error)"=w29) -> ("error out"=w28:errorcluster)  [unwired: 5 in, 1 out]
  n498 = control-ref of="This VI"() -> (w33:refnum<vi>)
  n499 = invoke on="Invoke Node" class="VI" method="Default Vals.Reinit All"(reference=w33, error in=w28) -> (reference out=w31:refnum<vi>, error out=w32:errorcluster)  [unwired: 1 in, 1 out]
  n500 = Close Reference(reference=w31, error in (no error)=w32) -> (error out=w26:errorcluster)
  n501 = call "Create User Event - Stop.vi"("error in (no error)"=w26) -> ("error out"=w4:errorcluster, "User Event - Stop"=w13:refnum<user-event>)  [unwired: 9 in]
  n502 = call "main screen queue out Unitest.vi"("error in (no error)"=w4) -> ("error out"=w53:errorcluster, "output Queue"=w25:T12)  [unwired: 9 in]
  n503 = Unbundle By Name(w25) -> ("UI Loop"=w51:refnum<queue>)
  n504 = Unbundle By Name(w25) -> ("LOAD COM LOOP"=w23:refnum<queue>)
  n505 = Unbundle By Name(w25) -> ("SWAY MOTOR COM LOOP"=w22:refnum<queue>)
  n506 = Unbundle By Name(w25) -> ("HEAVE MOTOR COM LOOP"=w5:refnum<queue>)
  n507 = Unbundle By Name(w25) -> ("TEMPERATURE COM LOOP"=w20:refnum<queue>)
  n508 = Unbundle By Name(w25) -> ("RAMP MOTOR COM LOOP"=w18:refnum<queue>)
  n509 = Unbundle By Name(w25) -> ("ECR PORT"=w17:refnum<queue>)
  n510 = Unbundle By Name(w25) -> ("HUMIDITY COM PORT"=w16:refnum<queue>)
  n511 = Unbundle By Name(w25) -> ("PROGRAM LOOP"=w15:refnum<queue>)
  n512 = Unbundle By Name(w25) -> ("MONITOR LOOP"=w12:refnum<queue>)
  n513 = Unbundle By Name(w25) -> ("LOAD PID"=w11:refnum<queue>)
  n514 = Unbundle By Name(w25) -> ("REPORT"=w10:refnum<queue>)
  n515 = register-events(w13) -> (reference out=w45:refnum<event-registration>, error out=w43:errorcluster)  [unwired: 2 in]
  n516 = Merge Errors(w43, w53) -> (w44:errorcluster)
  n517 = while {
    tunnel: w51 -> [w569]
    shift-right: [w567] -> w48
    shift-left: w45 -> [w568]
    tunnel: [w563] -> w46
    stop <- w565 stop-if-true
    # "Event Handling Loop"
    n518 = event shown="[32] \"Surge Backward MM\": Value Change" {
      selector: w568 -> [_ _ _ _ _ _ _ _ _ _ _ _ _ _ _ _ _ _ _ _ _ _ _ _ _ _ _ _ _ _ _ _ _ _ _ _ _ _ _ _ _ _]
      dyn-events: [_ _ _ _ _ _ _ _ _ _ _ _ _ _ _ _ _ _ _ _ _ _ _ _ _ _ _ _ _ _ _ _ _ _ _ _ _ _ _ _ _ _] -> w567
      timeout: 100 -> [_ _ _ _ _ _ _ _ _ _ _ _ _ _ _ _ _ _ _ _ _ _ _ _ _ _ _ _ _ _ _ _ _ _ _ _ _ _ _ _ _ _]
      tunnel: [_ _ _ _ _ _ _ _ _ _ _ _ _ _ _ _ _ _ _ _ _ _ _ _ _ _ _ _ _ _ _ _ _ _ _ _ _ _ _ _ _ TRUE ("Discard?")] -> w565
      tunnel: w569 -> [w574 w578 w583 w588 w593 w598 w603 w608 w613 w618 w623 w628 w633 w638 w643 w648 w653 w658 w663 w668 w673 w678 w683 w688 w693 w698 w703 w708 w713 w718 w723 w728 w733 w738 w743 w748 w753 w758 w763 w766 w771 w773]
      tunnel: [w573 w576 w581 w586 w591 w596 w601 w606 w611 w616 w621 w626 w631 w636 w641 w646 w651 w656 w661 w666 w671 w676 w681 w686 w691 w696 w701 w706 w711 w716 w721 w726 w731 w736 w741 w746 w751 w756 w761 _ w770 _] -> w566
      tunnel: [w572 w577 w582 w587 w592 w597 w602 w607 w612 w617 w622 w627 w632 w637 w642 w647 w652 w657 w662 w667 w672 w677 w682 w687 w692 w697 w702 w707 w712 w717 w722 w727 w732 w737 w742 w747 w752 w757 w762 w766 w769 w773] -> w564
      event Panel Close? {
        n519 = event-data() -> ()  [unwired: 1 in, 1 out]
        n520 = call-poly "Enqueue Message.vi"("Priority Message? (F)"=TRUE, "Message"="Confirm Quit", "Message Queue"=w574) -> ("error out"=w573:errorcluster, "dup Message Queue"=w572:refnum<queue>)  [unwired: 7 in]
        n521 = event-data("Discard?"=TRUE) -> ()  [unwired: 1 in, 1 out]
      }
      event Timeout {
        n522 = event-data() -> ()  [unwired: 1 in, 1 out]
        n523 = call-poly "Enqueue Message.vi"("Priority Message? (F)"=TRUE, "Message"="Time Out", "Message Queue"=w578) -> ("error out"=w576:errorcluster, "dup Message Queue"=w577:refnum<queue>)  [unwired: 7 in]
      }
      event "SAVE  2": Value Change {
        n524 = event-data() -> ()  [unwired: 1 in, 1 out]
        n525 = call-poly "Enqueue Message.vi"("Priority Message? (F)"=TRUE, "Message"="Service Save", "Message Queue"=w583) -> ("error out"=w581:errorcluster, "dup Message Queue"=w582:refnum<queue>)  [unwired: 7 in]
      }
      event "Home": Value Change {
        n526 = event-data() -> ()  [unwired: 1 in, 1 out]
        n527 = call-poly "Enqueue Message.vi"("Priority Message? (F)"=TRUE, "Message"="HOME", "Message Queue"=w588) -> ("error out"=w586:errorcluster, "dup Message Queue"=w587:refnum<queue>)  [unwired: 7 in]
      }
      event "Platform Settings": Value Change {
        n528 = event-data() -> ()  [unwired: 1 in, 1 out]
        n529 = call-poly "Enqueue Message.vi"("Priority Message? (F)"=TRUE, "Message"="Platform Setting", "Message Queue"=w593) -> ("error out"=w591:errorcluster, "dup Message Queue"=w592:refnum<queue>)  [unwired: 7 in]
      }
      event "Configure": Value Change {
        n530 = event-data() -> ()  [unwired: 1 in, 1 out]
        n531 = call-poly "Enqueue Message.vi"("Priority Message? (F)"=TRUE, "Message"="Configure", "Message Queue"=w598) -> ("error out"=w596:errorcluster, "dup Message Queue"=w597:refnum<queue>)  [unwired: 7 in]
      }
      event "Analysis": Value Change {
        n532 = event-data() -> ()  [unwired: 1 in, 1 out]
        n533 = call-poly "Enqueue Message.vi"("Priority Message? (F)"=TRUE, "Message"="Analysis", "Message Queue"=w603) -> ("error out"=w601:errorcluster, "dup Message Queue"=w602:refnum<queue>)  [unwired: 7 in]
      }
      event "service 2": Value Change {
        n534 = event-data() -> ()  [unwired: 1 in, 1 out]
        n535 = call-poly "Enqueue Message.vi"("Priority Message? (F)"=TRUE, "Message"="service 2", "Message Queue"=w608) -> ("error out"=w606:errorcluster, "dup Message Queue"=w607:refnum<queue>)  [unwired: 7 in]
      }
      event "Auto": Value Change {
        n536 = event-data() -> ()  [unwired: 1 in, 1 out]
        n537 = call-poly "Enqueue Message.vi"("Priority Message? (F)"=TRUE, "Message"="Auto", "Message Queue"=w613) -> ("error out"=w611:errorcluster, "dup Message Queue"=w612:refnum<queue>)  [unwired: 7 in]
      }
      event "Select Load Head": Value Change {
        n538 = event-data() -> ()  [unwired: 1 in, 1 out]
        n539 = call-poly "Enqueue Message.vi"("Priority Message? (F)"=TRUE, "Message"="Select Load Head", "Message Queue"=w618) -> ("error out"=w616:errorcluster, "dup Message Queue"=w617:refnum<queue>)  [unwired: 7 in]
      }
      event "com 3": Value Change {
        n540 = event-data() -> ()  [unwired: 1 in, 1 out]
        n541 = call-poly "Enqueue Message.vi"("Priority Message? (F)"=TRUE, "Message"="com 3", "Message Queue"=w623) -> ("error out"=w621:errorcluster, "dup Message Queue"=w622:refnum<queue>)  [unwired: 7 in]
      }
      event "Loading Mode": Value Change {
        n542 = event-data() -> ()  [unwired: 1 in, 1 out]
        n543 = call-poly "Enqueue Message.vi"("Priority Message? (F)"=TRUE, "Message"="Loading Mode", "Message Queue"=w628) -> ("error out"=w626:errorcluster, "dup Message Queue"=w627:refnum<queue>)  [unwired: 7 in]
      }
      event "SSP 0.3": Value Change {
        n544 = event-data() -> ()  [unwired: 1 in, 1 out]
        n545 = call-poly "Enqueue Message.vi"("Priority Message? (F)"=TRUE, "Message"="SSP 0.3", "Message Queue"=w633) -> ("error out"=w631:errorcluster, "dup Message Queue"=w632:refnum<queue>)  [unwired: 7 in]
      }
      event "SSP 0.5": Value Change {
        n546 = event-data() -> ()  [unwired: 1 in, 1 out]
        n547 = call-poly "Enqueue Message.vi"("Priority Message? (F)"=TRUE, "Message"="SSP 0.5", "Message Queue"=w638) -> ("error out"=w636:errorcluster, "dup Message Queue"=w637:refnum<queue>)  [unwired: 7 in]
      }
      event "SSP 0.75": Value Change {
        n548 = event-data() -> ()  [unwired: 1 in, 1 out]
        n549 = call-poly "Enqueue Message.vi"("Priority Message? (F)"=TRUE, "Message"="SSP 0.75", "Message Queue"=w643) -> ("error out"=w641:errorcluster, "dup Message Queue"=w642:refnum<queue>)  [unwired: 7 in]
      }
      event "LHBack": Value Change {
        n550 = event-data() -> ()  [unwired: 1 in, 1 out]
        n551 = call-poly "Enqueue Message.vi"("Priority Message? (F)"=TRUE, "Message"="LHBack", "Message Queue"=w648) -> ("error out"=w646:errorcluster, "dup Message Queue"=w647:refnum<queue>)  [unwired: 7 in]
      }
      event "LHNext": Value Change {
        n552 = event-data() -> ()  [unwired: 1 in, 1 out]
        n553 = call-poly "Enqueue Message.vi"("Priority Message? (F)"=TRUE, "Message"="LHNext", "Message Queue"=w653) -> ("error out"=w651:errorcluster, "dup Message Queue"=w652:refnum<queue>)  [unwired: 7 in]
      }
      event "Rot Ver": Value Change {
        n554 = event-data() -> ()  [unwired: 1 in, 1 out]
        n555 = call-poly "Enqueue Message.vi"("Priority Message? (F)"=TRUE, "Message"="Rot Ver", "Message Queue"=w658) -> ("error out"=w656:errorcluster, "dup Message Queue"=w657:refnum<queue>)  [unwired: 7 in]
      }
      event "Scratch": Value Change {
        n556 = event-data() -> ()  [unwired: 1 in, 1 out]
        n557 = call-poly "Enqueue Message.vi"("Priority Message? (F)"=TRUE, "Message"="Scratch", "Message Queue"=w663) -> ("error out"=w661:errorcluster, "dup Message Queue"=w662:refnum<queue>)  [unwired: 7 in]
      }
      event "Motion Mode:": Value Change {
        n558 = event-data() -> ()  [unwired: 1 in, 1 out]
        n559 = call-poly "Enqueue Message.vi"("Priority Message? (F)"=TRUE, "Message"="Motion Mode:", "Message Queue"=w668) -> ("error out"=w666:errorcluster, "dup Message Queue"=w667:refnum<queue>)  [unwired: 7 in]
      }
      event "MMBack": Value Change {
        n560 = event-data() -> ()  [unwired: 1 in, 1 out]
        n561 = call-poly "Enqueue Message.vi"("Priority Message? (F)"=TRUE, "Message"="MMBack", "Message Queue"=w673) -> ("error out"=w671:errorcluster, "dup Message Queue"=w672:refnum<queue>)  [unwired: 7 in]
      }
      event "MMNext": Value Change {
        n562 = event-data() -> ()  [unwired: 1 in, 1 out]
        n563 = call-poly "Enqueue Message.vi"("Priority Message? (F)"=TRUE, "Message"="MMNext", "Message Queue"=w678) -> ("error out"=w676:errorcluster, "dup Message Queue"=w677:refnum<queue>)  [unwired: 7 in]
      }
      event "APBack": Value Change {
        n564 = event-data() -> ()  [unwired: 1 in, 1 out]
        n565 = call-poly "Enqueue Message.vi"("Priority Message? (F)"=TRUE, "Message"="APBack", "Message Queue"=w683) -> ("error out"=w681:errorcluster, "dup Message Queue"=w682:refnum<queue>)  [unwired: 7 in]
      }
      event "SNext": Value Change {
        n566 = event-data() -> ()  [unwired: 1 in, 1 out]
        n567 = call-poly "Enqueue Message.vi"("Priority Message? (F)"=TRUE, "Message"="SNext", "Message Queue"=w688) -> ("error out"=w686:errorcluster, "dup Message Queue"=w687:refnum<queue>)  [unwired: 7 in]
      }
      event "ZeroAll": Value Change {
        n568 = event-data() -> ()  [unwired: 1 in, 1 out]
        n569 = call-poly "Enqueue Message.vi"("Priority Message? (F)"=TRUE, "Message"="ZeroAll", "Message Queue"=w693) -> ("error out"=w691:errorcluster, "dup Message Queue"=w692:refnum<queue>)  [unwired: 7 in]
      }
      event "Enable Platform": Value Change {
        n570 = event-data() -> ()  [unwired: 1 in, 1 out]
        n571 = call-poly "Enqueue Message.vi"("Priority Message? (F)"=TRUE, "Message"="Enable Platform", "Message Queue"=w698) -> ("error out"=w696:errorcluster, "dup Message Queue"=w697:refnum<queue>)  [unwired: 7 in]
      }
      event "Heave Up main": Value Change {
        n572 = event-data() -> ()  [unwired: 1 in, 1 out]
        n573 = call-poly "Enqueue Message.vi"("Priority Message? (F)"=TRUE, "Message"="Heave Up main", "Message Queue"=w703) -> ("error out"=w701:errorcluster, "dup Message Queue"=w702:refnum<queue>)  [unwired: 7 in]
      }
      event "Heave Up MM": Value Change {
        n574 = event-data() -> ()  [unwired: 1 in, 1 out]
        n575 = call-poly "Enqueue Message.vi"("Priority Message? (F)"=TRUE, "Message"="Heave Up MM", "Message Queue"=w708) -> ("error out"=w706:errorcluster, "dup Message Queue"=w707:refnum<queue>)  [unwired: 7 in]
      }
      event "Heave Down Main": Value Change {
        n576 = event-data() -> ()  [unwired: 1 in, 1 out]
        n577 = call-poly "Enqueue Message.vi"("Priority Message? (F)"=TRUE, "Message"="Heave Down Main", "Message Queue"=w713) -> ("error out"=w711:errorcluster, "dup Message Queue"=w712:refnum<queue>)  [unwired: 7 in]
      }
      event "Heave Down MM": Value Change {
        n578 = event-data() -> ()  [unwired: 1 in, 1 out]
        n579 = call-poly "Enqueue Message.vi"("Priority Message? (F)"=TRUE, "Message"="Heave Down MM", "Message Queue"=w718) -> ("error out"=w716:errorcluster, "dup Message Queue"=w717:refnum<queue>)  [unwired: 7 in]
      }
      event "Manual Write Heave & Surge": Value Change {
        n580 = event-data() -> ()  [unwired: 1 in, 1 out]
        n581 = call-poly "Enqueue Message.vi"("Priority Message? (F)"=TRUE, "Message"="Manual Write Heave & Surge", "Message Queue"=w723) -> ("error out"=w721:errorcluster, "dup Message Queue"=w722:refnum<queue>)  [unwired: 7 in]
      }
      event "Surge Backward Main": Value Change {
        n582 = event-data() -> ()  [unwired: 1 in, 1 out]
        n583 = call-poly "Enqueue Message.vi"("Priority Message? (F)"=TRUE, "Message"="Surge Backward Main", "Message Queue"=w728) -> ("error out"=w726:errorcluster, "dup Message Queue"=w727:refnum<queue>)  [unwired: 7 in]
      }
      event "Surge Backward MM": Value Change {
        n584 = event-data() -> ()  [unwired: 1 in, 1 out]
        n585 = call-poly "Enqueue Message.vi"("Priority Message? (F)"=TRUE, "Message"="Surge Backward MM", "Message Queue"=w733) -> ("error out"=w731:errorcluster, "dup Message Queue"=w732:refnum<queue>)  [unwired: 7 in]
      }
      event "Surge Forward Main": Value Change {
        n586 = event-data() -> ()  [unwired: 1 in, 1 out]
        n587 = call-poly "Enqueue Message.vi"("Priority Message? (F)"=TRUE, "Message"="Surge Forward Main", "Message Queue"=w738) -> ("error out"=w736:errorcluster, "dup Message Queue"=w737:refnum<queue>)  [unwired: 7 in]
      }
      event "Load En": Value Change {
        n588 = event-data() -> ()  [unwired: 1 in, 1 out]
        n589 = call-poly "Enqueue Message.vi"("Priority Message? (F)"=TRUE, "Message"="Load En", "Message Queue"=w743) -> ("error out"=w741:errorcluster, "dup Message Queue"=w742:refnum<queue>)  [unwired: 7 in]
      }
      event "apply load": Value Change {
        n590 = event-data() -> ()  [unwired: 1 in, 1 out]
        n591 = call-poly "Enqueue Message.vi"("Priority Message? (F)"=TRUE, "Message"="apply load", "Message Queue"=w748) -> ("error out"=w746:errorcluster, "dup Message Queue"=w747:refnum<queue>)  [unwired: 7 in]
      }
      event "BACK": Value Change {
        n592 = event-data() -> ()  [unwired: 1 in, 1 out]
        n593 = call-poly "Enqueue Message.vi"("Priority Message? (F)"=TRUE, "Message"="BACK", "Message Queue"=w753) -> ("error out"=w751:errorcluster, "dup Message Queue"=w752:refnum<queue>)  [unwired: 7 in]
      }
      event "Start Test": Value Change {
        n594 = event-data() -> ()  [unwired: 1 in, 1 out]
        n595 = call-poly "Enqueue Message.vi"("Priority Message? (F)"=TRUE, "Message"="Start Test", "Message Queue"=w758) -> ("error out"=w756:errorcluster, "dup Message Queue"=w757:refnum<queue>)  [unwired: 7 in]
      }
      event "STOP": Value Change {
        n596 = event-data() -> ()  [unwired: 1 in, 1 out]
        n597 = call-poly "Enqueue Message.vi"("Priority Message? (F)"=TRUE, "Message"="STOP", "Message Queue"=w763) -> ("error out"=w761:errorcluster, "dup Message Queue"=w762:refnum<queue>)  [unwired: 7 in]
      }
      event Application Instance Close {
        # "#CodeRecommended - When a project closes, all VIs within that project are aborted and leave memory. However, any code placed in this event frame is guaranteed to run to completion, so add any cleanup code that absolutely must happen here."
        n598 = event-data() -> ()  [unwired: 1 in, 1 out]
      }
      event "EXIT": Value Change {
        n599 = event-data() -> ()  [unwired: 1 in, 1 out]
        n600 = call-poly "Enqueue Message.vi"("Priority Message? (F)"=TRUE, "Message"="Exit", "Message Queue"=w771) -> ("error out"=w770:errorcluster, "dup Message Queue"=w769:refnum<queue>)  [unwired: 7 in]
      }
      event User Event {
        # "The Message Handling Loop processed an \"Exit\" message, which fired this event to stop the Event Handling Loop."
        n601 = event-data() -> ()  [unwired: 1 in, 1 out]
      }
    }
    n602 = call "LAB-IQ Error Handler - Event Handling Loop.vi"("error in (no error)"=w566, "Message Queue"=w564) -> ("dup error in"=w563:errorcluster)  [unwired: 8 in, 1 out]
  }
  n603 = while {
    tunnel: w51 -> [w788]
    shift-right: [w795] -> _
    shift-left: w14 -> [w796]
    tunnel: w13 -> [w793]
    tunnel: w44 -> [w792]
    tunnel: [w786] -> w52
    tunnel: w23 -> [w784]
    tunnel: w22 -> [w783]
    tunnel: w5 -> [w782]
    tunnel: w20 -> [w781]
    tunnel: w18 -> [w780]
    tunnel: w17 -> [w779]
    tunnel: w16 -> [w778]
    tunnel: w15 -> [w777]
    tunnel: w12 -> [w776]
    tunnel: w11 -> [w775]
    tunnel: w10 -> [w774]
    stop <- w794 stop-if-true
    # "Message Handling Loop"
    n604 = call "Dequeue Message.vi"("error in (no error)"=w792, "Message Queue"=w788) -> ("error out"=w791:errorcluster, "Message Data"=w789:variant, "Message"=w790:string, "dup Message Queue"=w787:refnum<queue>)  [unwired: 6 in]
    n605 = case "Message Cases" shown="\"Heave Down MM\"" w790 {
      selector: w790 -> [_ _ _ _ _ _ _ _ _ _ _ _ _ _ _ _ _ _ _ _ _ _ _ _ _ _ _ _ _ _ _ _ _ _ _ _ _ _ _ _ _ _ w1790]
      tunnel: w787 -> [_ w831 _ _ _ _ _ _ _ _ _ _ _ _ _ _ _ _ _ _ _ _ _ _ _ _ _ _ _ _ _ _ _ _ _ _ _ _ _ _ w1778 w1789 _]
      tunnel: w791 -> [w798 w833 w847 w876 w897 w914 w931 w948 w969 w981 w1031 w1036 w1043 w1048 w1113 w1139 w1165 w1196 w1208 w1256 w1276 w1365 w1442 w1481 w1493 w1518 w1548 w1567 w1578 w1589 w1600 w1611 w1622 w1632 w1644 w1666 w1706 w1733 w1763 w1770 w1781 w1782 _]
      tunnel: [w799 w830 w846 w877 w892 w909 w926 w943 w964 w973 w1009 w1034 w1041 w1052 w1109 w1135 w1161 w1197 w1209 w1220 w1267 w1356 w1441 w1480 w1492 w1517 w1535 w1569 w1580 w1591 w1602 w1613 w1624 w1634 w1643 w1665 w1704 w1731 w1740 w1764 w1773 w1785 w1791] -> w785
      tunnel: w796 -> [w797 w801 w848 w875 w883 w900 w917 w934 w952 w971 w986 w1033 w1039 w1047 w1111 w1137 w1163 w1187 w1199 w1211 w1260 w1348 w1436 w1479 w1491 w1503 w1530 w1565 w1576 w1587 w1598 w1609 w1620 w1631 w1642 w1664 w1685 w1710 w1739 w1769 w1771 w1788 w1792]
      tunnel: [w797 w801 w848 w875 w883 w900 w917 w934 w952 w971 w986 w1033 w1039 w1047 w1111 w1137 w1163 w1187 w1199 w1211 w1260 w1348 w1436 w1479 w1491 w1503 w1530 w1565 w1576 w1587 w1598 w1609 w1620 w1631 w1642 w1664 w1685 w1710 w1739 w1769 w1771 w1788 w1792] -> w795
      tunnel: [_ _ _ _ _ _ _ _ _ _ _ _ _ _ _ _ _ _ _ _ _ _ _ _ _ _ _ _ _ _ _ _ _ _ _ _ _ _ _ _ _ TRUE _] -> w794
      tunnel: w789 -> [_ _ _ _ _ _ _ _ _ _ _ _ _ _ _ _ _ _ _ _ _ _ _ _ _ _ _ _ _ _ _ _ _ _ _ _ _ _ _ w1768 _ _ _]
      tunnel: w793 -> [_ _ _ _ _ _ _ _ _ _ _ _ _ _ _ _ _ _ _ _ _ _ _ _ _ _ _ _ _ _ _ _ _ _ _ _ _ _ _ _ _ w1784 _]
      tunnel: w784 -> [_ _ w845 _ _ _ _ _ _ _ _ _ _ _ _ _ _ _ _ _ _ _ _ _ _ _ _ _ _ _ _ _ _ _ _ _ _ _ _ _ _ _ _]
      tunnel: w783 -> [_ _ w844 _ _ _ _ _ _ _ _ _ _ _ _ _ _ _ _ _ _ _ _ _ _ _ _ _ _ _ _ _ _ _ _ _ _ _ _ _ _ _ _]
      tunnel: w782 -> [_ _ w843 _ _ _ _ _ _ _ _ _ _ _ _ _ _ _ _ _ _ _ _ _ _ _ _ _ _ _ _ _ _ _ _ _ _ _ _ _ _ _ _]
      tunnel: w781 -> [_ _ w842 _ _ _ _ _ _ _ _ _ _ _ _ _ _ _ _ _ _ _ _ _ _ _ _ _ _ _ _ _ _ _ _ _ _ _ _ _ _ _ _]
      tunnel: w780 -> [_ _ w841 _ _ _ _ _ _ _ _ _ _ _ _ _ _ _ _ _ _ _ _ _ _ _ _ _ _ _ _ _ _ _ _ _ _ _ _ _ _ _ _]
      tunnel: w779 -> [_ _ w840 _ _ _ _ _ _ _ _ _ _ _ _ _ _ _ _ _ _ _ _ _ _ _ _ _ _ _ _ _ _ _ _ _ _ _ _ _ _ _ _]
      tunnel: w778 -> [_ _ w839 _ _ _ _ _ _ _ _ _ _ _ _ _ _ _ _ _ _ _ _ _ _ _ _ _ _ _ _ _ _ _ _ _ _ _ _ _ _ _ _]
      tunnel: w777 -> [_ _ w838 _ _ _ _ _ _ _ _ _ _ _ _ _ _ _ _ _ _ _ _ _ _ _ _ _ _ _ _ _ _ _ _ _ _ _ _ _ _ _ _]
      tunnel: w776 -> [_ _ w837 _ _ _ _ _ _ _ _ _ _ _ _ _ _ _ _ _ _ _ _ _ _ _ _ _ _ _ _ _ _ _ _ _ _ _ _ _ _ _ _]
      tunnel: w775 -> [_ _ w836 _ _ _ _ _ _ _ _ _ _ _ _ _ _ _ _ _ _ _ _ _ _ _ _ _ _ _ _ _ _ _ _ _ _ _ _ _ _ _ _]
      tunnel: w774 -> [_ _ w835 _ _ _ _ _ _ _ _ _ _ _ _ _ _ _ _ _ _ _ _ _ _ _ _ _ _ _ _ _ _ _ _ _ _ _ _ _ _ _ _]
      frame "Time Out" {
        n606 = call "Pulse_mm conversion loop.vi"("error in (no error)"=w798, "main ref"=w797) -> ("error out"=w799:errorcluster)  [unwired: 9 in]
        n607 = call "Load Commiunication Error.vi"("error in (no error)"=w798, "main ref"=w797) -> ()  [unwired: 9 in, 1 out]
      }
      frame "init" {
        # "Initialize - All initialization work should take place in this message, since other loops can potentially enqueue messages that execute immediately after this one."
        n608 = call-poly "Enqueue Message.vi"("error in (no error)"=w833, "Message"="Init Other Loop", "Message Queue"=w831) -> ("error out"=w834:errorcluster)  [unwired: 7 in, 1 out]
        n609 = Unbundle By Name(w801) -> ("Loading.Communication is established"=w806:refnum<vi>)
        n610 = Unbundle By Name(w801) -> ("Loading Com Port.Load Cell Temp"=w825:refnum<vi>)
        n611 = Unbundle By Name(w801) -> ("Loading.SSP 0.3"=w819:refnum<vi>)
        n612 = Unbundle By Name(w801) -> ("Loading.SSP 0.5"=w816:refnum<vi>)
        n613 = Unbundle By Name(w801) -> ("Loading.SSP 0.75"=w811:refnum<vi>)
        n614 = call "Read Config Unitest.vi"("error in (no error)"=w834, "main ref"=w801) -> ("error out"=w829:errorcluster)  [unwired: 9 in]
        n615 = Unbundle By Name(w801) -> ("PID.Ramp"=w803:refnum<vi>)
        n616 = call "Encrypt file path creation.vi"("error in (no error)"=w829) -> ("error out"=w828:errorcluster, "File Path"=w827:path)  [unwired: 9 in]
        n617 = property class="Bool (strict)"(reference=w825, "Value"=FALSE) -> (reference out=w823:refnum<vi>, error out=w824:errorcluster)  [unwired: 1 in]
        n618 = property class="Bool (strict)"(reference=w816, "Visible"=FALSE) -> (reference out=w814:refnum<vi>, error out=w815:errorcluster)  [unwired: 1 in]
        n619 = property class="Bool (strict)"(reference=w819, "Visible"=FALSE) -> (reference out=w821:refnum<vi>, error out=w820:errorcluster)  [unwired: 1 in]
        n620 = property class="Bool (strict)"(reference=w811, "Visible"=FALSE) -> (reference out=w813:refnum<vi>, error out=w812:errorcluster)  [unwired: 1 in]
        n621 = property class="Bool (strict)"(reference=w803, "Value"=FALSE) -> (reference out=w805:refnum<vi>, error out=w804:errorcluster)  [unwired: 1 in]
        n622 = property class="Bool (strict)"(reference=w806, "Visible"=FALSE ("Value")) -> (reference out=w808:refnum<vi>, error out=w807:errorcluster)  [unwired: 1 in]
        n623 = call "DATA ENCRYPT STRING FILE WRITE.vi"("file path (dialog if empty)"=w827, "error in (no error)"=w828, "User Action"="System Booted", "main ref"=w801) -> ("error out"=w830:errorcluster)  [unwired: 5 in, 1 out]
        n624 = Close Reference(reference=w814, error in (no error)=w815) -> ()  [unwired: 1 out]
        n625 = Close Reference(reference=w821, error in (no error)=w820) -> ()  [unwired: 1 out]
        n626 = Close Reference(reference=w813, error in (no error)=w812) -> ()  [unwired: 1 out]
        n627 = Close Reference(reference=w805, error in (no error)=w804) -> ()  [unwired: 1 out]
        n628 = Close Reference(reference=w823, error in (no error)=w824) -> ()  [unwired: 1 out]
        n629 = Close Reference(reference=w808, error in (no error)=w807) -> ()  [unwired: 1 out]
        n630 = local write "HEAVE ENABLE"(TRUE ("HEAVE ENABLE")) -> ()
      }
      frame "Init Other Loop" {
        n631 = disable-structure shown="Disabled" {
          disable-tunnel: w847 -> [w872 w873]
          disable-tunnel: [w861 w873] -> w846
          disable-tunnel: w845 -> [w859 _]
          disable-tunnel: w844 -> [w858 _]
          disable-tunnel: w843 -> [w857 _]
          disable-tunnel: w842 -> [w856 _]
          disable-tunnel: w841 -> [w855 _]
          disable-tunnel: w840 -> [w854 _]
          disable-tunnel: w839 -> [w853 _]
          disable-tunnel: w838 -> [w852 _]
          disable-tunnel: w837 -> [w851 _]
          disable-tunnel: w836 -> [w850 _]
          disable-tunnel: w835 -> [w849 _]
          frame Disabled {
            w860 = "Init" ("Message")
            n632 = call-poly "Enqueue Message.vi"("error in (no error)"=w872, "Message"=w860, "Message Queue"=w859) -> ("error out"=w871:errorcluster)  [unwired: 7 in, 1 out]
            n633 = call-poly "Enqueue Message.vi"("error in (no error)"=w871, "Message"=w860, "Message Queue"=w858) -> ("error out"=w870:errorcluster)  [unwired: 7 in, 1 out]
            n634 = call-poly "Enqueue Message.vi"("error in (no error)"=w870, "Message"=w860, "Message Queue"=w857) -> ("error out"=w869:errorcluster)  [unwired: 7 in, 1 out]
            n635 = call-poly "Enqueue Message.vi"("error in (no error)"=w869, "Message"=w860, "Message Queue"=w856) -> ("error out"=w868:errorcluster)  [unwired: 7 in, 1 out]
            n636 = call-poly "Enqueue Message.vi"("error in (no error)"=w868, "Message"=w860, "Message Queue"=w855) -> ("error out"=w867:errorcluster)  [unwired: 7 in, 1 out]
            n637 = call-poly "Enqueue Message.vi"("error in (no error)"=w867, "Message"=w860, "Message Queue"=w854) -> ("error out"=w866:errorcluster)  [unwired: 7 in, 1 out]
            n638 = call-poly "Enqueue Message.vi"("error in (no error)"=w866, "Message"=w860, "Message Queue"=w853) -> ("error out"=w865:errorcluster)  [unwired: 7 in, 1 out]
            n639 = call-poly "Enqueue Message.vi"("error in (no error)"=w865, "Message"=w860, "Message Queue"=w852) -> ("error out"=w864:errorcluster)  [unwired: 7 in, 1 out]
            n640 = call-poly "Enqueue Message.vi"("error in (no error)"=w864, "Message"=w860, "Message Queue"=w851) -> ("error out"=w863:errorcluster)  [unwired: 7 in, 1 out]
            n641 = call-poly "Enqueue Message.vi"("error in (no error)"=w863, "Message"=w860, "Message Queue"=w850) -> ("error out"=w862:errorcluster)  [unwired: 7 in, 1 out]
            n642 = call-poly "Enqueue Message.vi"("error in (no error)"=w862, "Message"=w860, "Message Queue"=w849) -> ("error out"=w861:errorcluster)  [unwired: 7 in, 1 out]
          }
          frame Enabled {
          }
        }
      }
      frame "Service Save" {
        n643 = call "Write Config Unitest.vi"("error in (no error)"=w876, "main ref"=w875) -> ("error out"=w881:errorcluster)  [unwired: 9 in]
        n644 = call "Stall Data Flow.vim"("value in"=w881, "milliseconds to wait"=u32 2000) -> ("value out"=w880:errorcluster)  [unwired: 1 out]
        n645 = call "Read Config Unitest.vi"("error in (no error)"=w880, "main ref"=w875) -> ("error out"=w878:errorcluster)  [unwired: 9 in]
        n646 = call "DATA ENCRYPT STRING FILE WRITE.vi"("error in (no error)"=w878, "User Action"="Service Parameter Saved", "main ref"=w875) -> ("error out"=w877:errorcluster)  [unwired: 6 in, 1 out]
      }
      frame "HOME" {
        n647 = call "DATA ENCRYPT STRING FILE WRITE.vi"("error in (no error)"=w897, "User Action"="User Pressed Home", "main ref"=w883) -> ("error out"=w893:errorcluster)  [unwired: 6 in, 1 out]
        n648 = Unbundle By Name(w883) -> ("Main Home Screen.MainPage"=w888:refnum<vi>)
        n649 = Unbundle By Name(w883) -> ("Main Home Screen.Home"=w896:refnum<vi>)
        n650 = Unbundle By Name(w883) -> ("Main Home Screen.GUI"=w886:refnum<vi>)
        n651 = property class="Bool (strict)"(reference=w896, error in=w893, "Value"=FALSE) -> (reference out=w894:refnum<vi>, error out=w895:errorcluster)
        n652 = property class="TabCtl (strict)"(reference=w888, "Value"=T5."HOME") -> (reference out=w890:refnum<vi>, error out=w889:errorcluster)  [unwired: 1 in]
        n653 = property class="TabCtl (strict)"(reference=w886, "Value"=T4."Setup") -> (reference out=w884:refnum<vi>, error out=w885:errorcluster)  [unwired: 1 in]
        n654 = Close Reference(reference=w894, error in (no error)=w895) -> (error out=w892:errorcluster)
        n655 = Close Reference(reference=w890, error in (no error)=w889) -> ()  [unwired: 1 out]
        n656 = Close Reference(reference=w884, error in (no error)=w885) -> ()  [unwired: 1 out]
      }
      frame "Platform Setting" {
        n657 = call "DATA ENCRYPT STRING FILE WRITE.vi"("error in (no error)"=w914, "User Action"="User Pressed Platform Setting", "main ref"=w900) -> ("error out"=w910:errorcluster)  [unwired: 6 in, 1 out]
        n658 = Unbundle By Name(w900) -> ("Main Home Screen.Platform Settings"=w913:refnum<vi>)
        n659 = Unbundle By Name(w900) -> ("Main Home Screen.MainPage"=w905:refnum<vi>)
        n660 = Unbundle By Name(w900) -> ("Main Home Screen.GUI"=w903:refnum<vi>)
        n661 = property class="TabCtl (strict)"(reference=w905, "Value"=T5."PlatformSetting") -> (reference out=w907:refnum<vi>, error out=w906:errorcluster)  [unwired: 1 in]
        n662 = property class="TabCtl (strict)"(reference=w903, "Value"=T4."Setup") -> (reference out=w901:refnum<vi>, error out=w902:errorcluster)  [unwired: 1 in]
        n663 = property class="Bool (strict)"(reference=w913, error in=w910, "Value"=FALSE) -> (reference out=w911:refnum<vi>, error out=w912:errorcluster)
        n664 = Close Reference(reference=w907, error in (no error)=w906) -> ()  [unwired: 1 out]
        n665 = Close Reference(reference=w901, error in (no error)=w902) -> ()  [unwired: 1 out]
        n666 = Close Reference(reference=w911, error in (no error)=w912) -> (error out=w909:errorcluster)
      }
      frame "Configure" {
        n667 = call "DATA ENCRYPT STRING FILE WRITE.vi"("error in (no error)"=w931, "User Action"="User Pressed Configure", "main ref"=w917) -> ("error out"=w927:errorcluster)  [unwired: 6 in, 1 out]
        n668 = Unbundle By Name(w917) -> ("Main Home Screen.Configure"=w930:refnum<vi>)
        n669 = Unbundle By Name(w917) -> ("Main Home Screen.MainPage"=w922:refnum<vi>)
        n670 = Unbundle By Name(w917) -> ("Main Home Screen.GUI"=w920:refnum<vi>)
        n671 = property class="Bool (strict)"(reference=w930, error in=w927, "Value"=FALSE) -> (reference out=w928:refnum<vi>, error out=w929:errorcluster)
        n672 = property class="TabCtl (strict)"(reference=w922, "Value"=T5."Details") -> (reference out=w924:refnum<vi>, error out=w923:errorcluster)  [unwired: 1 in]
        n673 = property class="TabCtl (strict)"(reference=w920, "Value"=T4."Setup") -> (reference out=w918:refnum<vi>, error out=w919:errorcluster)  [unwired: 1 in]
        n674 = Close Reference(reference=w928, error in (no error)=w929) -> (error out=w926:errorcluster)
        n675 = Close Reference(reference=w924, error in (no error)=w923) -> ()  [unwired: 1 out]
        n676 = Close Reference(reference=w918, error in (no error)=w919) -> ()  [unwired: 1 out]
      }
      frame "Analysis" {
        n677 = call "DATA ENCRYPT STRING FILE WRITE.vi"("error in (no error)"=w948, "User Action"="User Pressed Analysis", "main ref"=w934) -> ("error out"=w944:errorcluster)  [unwired: 6 in, 1 out]
        n678 = Unbundle By Name(w934) -> ("Main Home Screen.MainPage"=w939:refnum<vi>)
        n679 = Unbundle By Name(w934) -> ("Main Home Screen.Analysis"=w947:refnum<vi>)
        n680 = Unbundle By Name(w934) -> ("Main Home Screen.GUI"=w937:refnum<vi>)
        n681 = property class="Bool (strict)"(reference=w947, error in=w944, "Value"=FALSE) -> (reference out=w945:refnum<vi>, error out=w946:errorcluster)
        n682 = property class="TabCtl (strict)"(reference=w939, "Value"=T5."Analysis") -> (reference out=w941:refnum<vi>, error out=w940:errorcluster)  [unwired: 1 in]
        n683 = property class="TabCtl (strict)"(reference=w937, "Value"=T4."Setup") -> (reference out=w935:refnum<vi>, error out=w936:errorcluster)  [unwired: 1 in]
        n684 = Close Reference(reference=w945, error in (no error)=w946) -> (error out=w943:errorcluster)
        n685 = Close Reference(reference=w941, error in (no error)=w940) -> ()  [unwired: 1 out]
        n686 = Close Reference(reference=w935, error in (no error)=w936) -> ()  [unwired: 1 out]
      }
      frame "service 2" {
        n687 = call "DATA ENCRYPT STRING FILE WRITE.vi"("error in (no error)"=w969, "User Action"="User Pressed service", "main ref"=w952) -> ("error out"=w965:errorcluster)  [unwired: 6 in, 1 out]
        n688 = Unbundle By Name(w952) -> ("Main Screen.Main Screen Tab"=w953:refnum<vi>)
        n689 = Unbundle By Name(w952) -> ("Main Home Screen.MainPage"=w960:refnum<vi>)
        n690 = Unbundle By Name(w952) -> ("Main Home Screen.Analysis"=w968:refnum<vi>)
        n691 = Unbundle By Name(w952) -> ("Main Home Screen.GUI"=w958:refnum<vi>)
        n692 = property class="Bool (strict)"(reference=w968, error in=w965, "Value"=FALSE) -> (reference out=w966:refnum<vi>, error out=w967:errorcluster)
        n693 = property class="TabCtl (strict)"(reference=w960, "Value"=T5."HOME") -> (reference out=w962:refnum<vi>, error out=w961:errorcluster)  [unwired: 1 in]
        n694 = property class="TabCtl (strict)"(reference=w958, "Value"=T4."Begin") -> (reference out=w956:refnum<vi>, error out=w957:errorcluster)  [unwired: 1 in]
        n695 = property class="TabCtl (strict)"(reference=w953, "Value"=T8."About") -> (reference out=w950:refnum<vi>, error out=w954:errorcluster)  [unwired: 1 in]
        n696 = Close Reference(reference=w966, error in (no error)=w967) -> (error out=w964:errorcluster)
        n697 = Close Reference(reference=w962, error in (no error)=w961) -> ()  [unwired: 1 out]
        n698 = Close Reference(reference=w956, error in (no error)=w957) -> ()  [unwired: 1 out]
        n699 = Close Reference(reference=w950, error in (no error)=w954) -> ()  [unwired: 1 out]
      }
      frame "Auto" {
        n700 = call "DATA ENCRYPT STRING FILE WRITE.vi"("error in (no error)"=w981, "User Action"="User Pressed Auto File Name", "main ref"=w971) -> ("error out"=w978:errorcluster)  [unwired: 6 in, 1 out]
        n701 = Get Date/Time In Seconds() -> (seconds since 1Jan1904=w979:timestamp)
        n702 = Format Into String(format string="%<%I_%M_%S_%p_%d_%B_%Y>T", error in=w978, w979) -> (resulting string=w972:string, error out=w974:errorcluster)  [unwired: 1 in]
        n703 = Unbundle By Name(w971) -> ("Config Screen.FILE"=w977:refnum<vi>)
        n704 = property class="Str"(reference=w977, error in=w974, "Value"=w972) -> (reference out=w975:refnum<vi>, error out=w976:errorcluster)
        n705 = Close Reference(reference=w975, error in (no error)=w976) -> (error out=w973:errorcluster)
      }
      frame "Select Load Head" {
        n706 = Unbundle By Name(w986) -> ("Loading.Enter the Loading Rate (N/min)"=w1007:refnum<vi>)
        n707 = Unbundle By Name(w986) -> ("Loading.Communication is established"=w992:refnum<vi>)
        n708 = call "DATA ENCRYPT STRING FILE WRITE.vi"("error in (no error)"=w1031, "User Action"="User Pressed Select Load Head", "main ref"=w986) -> ("error out"=w1027:errorcluster)  [unwired: 6 in, 1 out]
        n709 = Unbundle By Name(w986) -> ("Loading.Enter the Final Load (N)"=w1002:refnum<vi>)
        n710 = Unbundle By Name(w986) -> ("Loading.DecaForce COM Status"=w988:refnum<vi>)
        n711 = Unbundle By Name(w986) -> ("Loading.Loading Mode"=w1030:refnum<vi>)
        n712 = Unbundle By Name(w986) -> ("Config Screen.Select Load Head"=w1014:refnum<vi>)
        n713 = Unbundle By Name(w986) -> ("Loading.Warning"=w997:refnum<vi>)
        n714 = Unbundle By Name(w986) -> ("Loading.Load Selection"=w1023:refnum<vi>)
        n715 = property class="Bool (strict)"(reference=w1014, "Value"=FALSE) -> (reference out=w1012:refnum<vi>, error out=w1013:errorcluster)  [unwired: 1 in]
        n716 = property class="TabCtl (strict)"(reference=w1023, "Value"=T6."Constant") -> (reference out=w1025:refnum<vi>, error out=w1024:errorcluster)  [unwired: 1 in]
        n717 = property class="Ring (strict)"(reference=w1030, error in=w1027, "Value"=u16 0) -> (reference out=w1028:refnum<vi>, error out=w1029:errorcluster)
        n718 = property class="DigNum (strict)"(reference=w1007, "DisabledEnum"=T13."Disabled and Grayed Out" ("Disabled")) -> (reference out=w1006:refnum<vi>, error out=w1008:errorcluster)  [unwired: 1 in]
        n719 = property class="DigNum (strict)"(reference=w1002, "DisabledEnum"=T13."Disabled and Grayed Out" ("Disabled")) -> (reference out=w1003:refnum<vi>, error out=w1001:errorcluster)  [unwired: 1 in]
        n720 = property class="TabCtl (strict)"(reference=w997, "Visible"=FALSE) -> (reference out=w996:refnum<vi>, error out=w998:errorcluster)  [unwired: 1 in]
        n721 = property class="Bool (strict)"(reference=w992, "Visible"=FALSE) -> (reference out=w990:refnum<vi>, error out=w991:errorcluster)  [unwired: 1 in]
        n722 = property class="Bool (strict)"(reference=w988, "Visible"=FALSE) -> (reference out=w983:refnum<vi>, error out=w989:errorcluster)  [unwired: 1 in]
        n723 = Close Reference(reference=w1012, error in (no error)=w1013) -> (error out=w1010:errorcluster)
        n724 = Close Reference(reference=w1025, error in (no error)=w1024) -> (error out=w1016:errorcluster)
        n725 = Close Reference(reference=w1028, error in (no error)=w1029) -> (error out=w1018:errorcluster)
        n726 = Close Reference(reference=w1006, error in (no error)=w1008) -> (error out=w1000:errorcluster)
        n727 = Close Reference(reference=w1003, error in (no error)=w1001) -> (error out=w999:errorcluster)
        n728 = Close Reference(reference=w996, error in (no error)=w998) -> (error out=w995:errorcluster)
        n729 = Close Reference(reference=w990, error in (no error)=w991) -> (error out=w985:errorcluster)
        n730 = Close Reference(reference=w983, error in (no error)=w989) -> (error out=w984:errorcluster)
        n731 = Merge Errors(w1018, w1016, w1010, w1000, w999, w995, w985, w984) -> (w1017:errorcluster)
        n732 = Unbundle By Name(w986) -> ("Main Home Screen.GUI"=w1019:refnum<vi>)
        n733 = property class="TabCtl (strict)"(reference=w1019, error in=w1017, "Value"=T4."Load Head") -> (reference out=w1021:refnum<vi>, error out=w1020:errorcluster)
        n734 = Close Reference(reference=w1021, error in (no error)=w1020) -> (error out=w1009:errorcluster)
      }
      frame "com 3" {
        n735 = call "DATA ENCRYPT STRING FILE WRITE.vi"("error in (no error)"=w1036, "User Action"="User Pressed Check Load Communication", "main ref"=w1033) -> ("error out"=w1035:errorcluster)  [unwired: 6 in, 1 out]
        n736 = call "SET LOAD PARAMETERS.vi"("error in (no error)"=w1035, "main ref"=w1033) -> ("error out"=w1034:errorcluster)  [unwired: 9 in]
      }
      frame "ZeroAll" {
        n737 = call "DATA ENCRYPT STRING FILE WRITE.vi"("error in (no error)"=w1043, "User Action"="User Pressed Zero All", "main ref"=w1039) -> ("error out"=w1042:errorcluster)  [unwired: 6 in, 1 out]
        n738 = local write "ZeroAll"(FALSE ("ZeroAll")) -> ()
        n739 = call "LOAD CELL FGV MAIN.vi"("Enum"=T14."ZEROALL", "error in (no error)"=w1042, "main ref"=w1039) -> ("error IO"=w1041:errorcluster)  [unwired: 8 in]
      }
      frame "Loading Mode" {
        n740 = Unbundle By Name(w1047) -> ("Loading.Loading Mode"=w1049:refnum<vi>)
        n741 = property class="Ring (strict)"(reference=w1049, error in=w1048) -> (reference out=w1051:refnum<vi>, error out=w1050:errorcluster, "Value"=w1045:u16)
        n742 = Close Reference(reference=w1051, error in (no error)=w1050) -> (error out=w1046:errorcluster)
        n743 = case shown="1" w1045 {
          tunnel: [w1066 w1083 w1095 w1107] -> w1052
          tunnel: w1047 -> [w1053 w1069 w1087 w1099]
          tunnel: w1046 -> [w1067 w1082 w1094 w1106]
          frame 0, Default {
            n744 = Unbundle By Name(w1053) -> ("Loading.Enter the Loading Rate (N/min)"=w1060:refnum<vi>)
            n745 = Unbundle By Name(w1053) -> ("Loading.Load Selection"=w1063:refnum<vi>)
            n746 = Unbundle By Name(w1053) -> ("Loading.Enter the Final Load (N)"=w1055:refnum<vi>)
            n747 = property class="TabCtl (strict)"(reference=w1063, "Value"=T6."Constant") -> (reference out=w1065:refnum<vi>, error out=w1064:errorcluster)  [unwired: 1 in]
            n748 = property class="DigNum (strict)"(reference=w1060, "DisabledEnum"=T13."Disabled and Grayed Out" ("Disabled")) -> (reference out=w1059:refnum<vi>, error out=w1061:errorcluster)  [unwired: 1 in]
            n749 = property class="DigNum (strict)"(reference=w1055, "DisabledEnum"=T13."Disabled and Grayed Out" ("Disabled")) -> (reference out=w1056:refnum<vi>, error out=w1054:errorcluster)  [unwired: 1 in]
            n750 = call "DATA ENCRYPT STRING FILE WRITE.vi"("error in (no error)"=w1067, "User Action"="User selected Constant Mode", "main ref"=w1053) -> ("error out"=w1066:errorcluster)  [unwired: 6 in, 1 out]
            n751 = Close Reference(reference=w1065, error in (no error)=w1064) -> ()  [unwired: 1 out]
            n752 = Close Reference(reference=w1059, error in (no error)=w1061) -> ()  [unwired: 1 out]
            n753 = Close Reference(reference=w1056, error in (no error)=w1054) -> ()  [unwired: 1 out]
          }
          frame 1 {
            n754 = Unbundle By Name(w1069) -> ("Loading.Enter the Loading Rate (N/min)"=w1080:refnum<vi>)
            n755 = Unbundle By Name(w1069) -> ("Loading.Enter the Final Load (N)"=w1075:refnum<vi>)
            n756 = Unbundle By Name(w1069) -> ("Loading.Load Selection"=w1071:refnum<vi>)
            n757 = property class="TabCtl (strict)"(reference=w1071, "Value"=T6."Constant") -> (reference out=w1073:refnum<vi>, error out=w1072:errorcluster)  [unwired: 1 in]
            n758 = property class="DigNum (strict)"(reference=w1080, "DisabledEnum"=T13."Enabled" ("Disabled")) -> (reference out=w1079:refnum<vi>, error out=w1081:errorcluster)  [unwired: 1 in]
            n759 = property class="DigNum (strict)"(reference=w1075, "DisabledEnum"=T13."Enabled" ("Disabled")) -> (reference out=w1076:refnum<vi>, error out=w1074:errorcluster)  [unwired: 1 in]
            n760 = call "DATA ENCRYPT STRING FILE WRITE.vi"("error in (no error)"=w1082, "User Action"="User selected Ramp Mode", "main ref"=w1069) -> ("error out"=w1083:errorcluster)  [unwired: 6 in, 1 out]
            n761 = Close Reference(reference=w1073, error in (no error)=w1072) -> ()  [unwired: 1 out]
            n762 = Close Reference(reference=w1079, error in (no error)=w1081) -> ()  [unwired: 1 out]
            n763 = Close Reference(reference=w1076, error in (no error)=w1074) -> ()  [unwired: 1 out]
          }
          frame 2 {
            n764 = Unbundle By Name(w1087) -> ("Loading.Load Selection"=w1091:refnum<vi>)
            n765 = Unbundle By Name(w1087) -> ("Loading.Warning 2"=w1089:refnum<vi>)
            n766 = property class="TabCtl (strict)"(reference=w1091, "Value"=T6."Step") -> (reference out=w1093:refnum<vi>, error out=w1092:errorcluster)  [unwired: 1 in]
            n767 = property class="Bool (strict)"(reference=w1089, "Visible"=FALSE) -> (reference out=w1085:refnum<vi>, error out=w1088:errorcluster)  [unwired: 1 in]
            n768 = call "DATA ENCRYPT STRING FILE WRITE.vi"("error in (no error)"=w1094, "User Action"="User selected Step Mode", "main ref"=w1087) -> ("error out"=w1095:errorcluster)  [unwired: 6 in, 1 out]
            n769 = Close Reference(reference=w1093, error in (no error)=w1092) -> ()  [unwired: 1 out]
            n770 = Close Reference(reference=w1085, error in (no error)=w1088) -> ()  [unwired: 1 out]
          }
          frame 3 {
            n771 = Unbundle By Name(w1099) -> ("Loading.Load Selection"=w1103:refnum<vi>)
            n772 = Unbundle By Name(w1099) -> ("Loading.Warning 2"=w1101:refnum<vi>)
            n773 = property class="TabCtl (strict)"(reference=w1103, "Value"=T6."Indentation") -> (reference out=w1105:refnum<vi>, error out=w1104:errorcluster)  [unwired: 1 in]
            n774 = property class="Bool (strict)"(reference=w1101, "Visible"=FALSE) -> (reference out=w1097:refnum<vi>, error out=w1100:errorcluster)  [unwired: 1 in]
            n775 = call "DATA ENCRYPT STRING FILE WRITE.vi"("error in (no error)"=w1106, "User Action"="User selected Indentation Mode", "main ref"=w1099) -> ("error out"=w1107:errorcluster)  [unwired: 6 in, 1 out]
            n776 = Close Reference(reference=w1105, error in (no error)=w1104) -> ()  [unwired: 1 out]
            n777 = Close Reference(reference=w1097, error in (no error)=w1100) -> ()  [unwired: 1 out]
          }
        }
      }
      frame "SSP 0.3" {
        n778 = Unbundle By Name(w1111) -> ("Loading.SSP 0.3"=w1114:refnum<vi>)
        n779 = property class="Bool (strict)"(reference=w1114, error in=w1113) -> (reference out=w1116:refnum<vi>, error out=w1115:errorcluster, "Value"=w1112:bool)
        n780 = Close Reference(reference=w1116, error in (no error)=w1115) -> (error out=w1110:errorcluster)
        n781 = case shown="True" w1112 {
          tunnel: w1111 -> [_ w1118]
          tunnel: w1110 -> [w1117 w1126]
          tunnel: [w1117 w1125] -> w1109
          frame False {
          }
          frame True {
            w1128 = FALSE ("Value")
            n782 = Unbundle By Name(w1118) -> ("Loading.Enter the Load  (N)"=w1124:refnum<vi>)
            n783 = Unbundle By Name(w1118) -> ("Loading.SSP 0.75"=w1129:refnum<vi>)
            n784 = Unbundle By Name(w1118) -> ("Loading.SSP 0.5"=w1134:refnum<vi>)
            n785 = property class="Bool (strict)"(reference=w1129, "Value"=w1128) -> (reference out=w1131:refnum<vi>, error out=w1130:errorcluster)  [unwired: 1 in]
            n786 = property class="Bool (strict)"(reference=w1134, "Value"=w1128) -> (reference out=w1132:refnum<vi>, error out=w1133:errorcluster)  [unwired: 1 in]
            n787 = property class="DigNum (strict)"(reference=w1124, "Minimum"=2.0 ("Data Entry Limits:Minimum"), "Maximum"=50.0 ("Data Entry Limits:Maximum"), "Increment"=0.1 ("Data Entry Limits:Increment")) -> (reference out=w1122:refnum<vi>, error out=w1123:errorcluster)  [unwired: 1 in]
            n788 = call "DATA ENCRYPT STRING FILE WRITE.vi"("error in (no error)"=w1126, "User Action"="User selected 0.3 SSP", "main ref"=w1118) -> ("error out"=w1125:errorcluster)  [unwired: 6 in, 1 out]
            n789 = Close Reference(reference=w1131, error in (no error)=w1130) -> ()  [unwired: 1 out]
            n790 = Close Reference(reference=w1132, error in (no error)=w1133) -> ()  [unwired: 1 out]
            n791 = Close Reference(reference=w1122, error in (no error)=w1123) -> ()  [unwired: 1 out]
          }
        }
      }
      frame "SSP 0.5" {
        n792 = Unbundle By Name(w1137) -> ("Loading.SSP 0.5"=w1140:refnum<vi>)
        n793 = property class="Bool (strict)"(reference=w1140, error in=w1139) -> (reference out=w1142:refnum<vi>, error out=w1141:errorcluster, "Value"=w1138:bool)
        n794 = Close Reference(reference=w1142, error in (no error)=w1141) -> (error out=w1136:errorcluster)
        n795 = case shown="True" w1138 {
          tunnel: w1137 -> [_ w1144]
          tunnel: w1136 -> [w1143 w1152]
          tunnel: [w1143 w1151] -> w1135
          frame False {
          }
          frame True {
            w1154 = FALSE ("Value")
            n796 = Unbundle By Name(w1144) -> ("Loading.Enter the Load  (N)"=w1150:refnum<vi>)
            n797 = Unbundle By Name(w1144) -> ("Loading.SSP 0.75"=w1160:refnum<vi>)
            n798 = Unbundle By Name(w1144) -> ("Loading.SSP 0.3"=w1155:refnum<vi>)
            n799 = property class="Bool (strict)"(reference=w1155, "Value"=w1154) -> (reference out=w1157:refnum<vi>, error out=w1156:errorcluster)  [unwired: 1 in]
            n800 = property class="Bool (strict)"(reference=w1160, "Value"=w1154) -> (reference out=w1158:refnum<vi>, error out=w1159:errorcluster)  [unwired: 1 in]
            n801 = property class="DigNum (strict)"(reference=w1150, "Minimum"=2.0 ("Data Entry Limits:Minimum"), "Maximum"=200.0 ("Data Entry Limits:Maximum"), "Increment"=0.1 ("Data Entry Limits:Increment")) -> (reference out=w1148:refnum<vi>, error out=w1149:errorcluster)  [unwired: 1 in]
            n802 = call "DATA ENCRYPT STRING FILE WRITE.vi"("error in (no error)"=w1152, "User Action"="User selected 0.5 SSP", "main ref"=w1144) -> ("error out"=w1151:errorcluster)  [unwired: 6 in, 1 out]
            n803 = Close Reference(reference=w1157, error in (no error)=w1156) -> ()  [unwired: 1 out]
            n804 = Close Reference(reference=w1158, error in (no error)=w1159) -> ()  [unwired: 1 out]
            n805 = Close Reference(reference=w1148, error in (no error)=w1149) -> ()  [unwired: 1 out]
          }
        }
      }
      frame "SSP 0.75" {
        n806 = Unbundle By Name(w1163) -> ("Loading.SSP 0.75"=w1166:refnum<vi>)
        n807 = property class="Bool (strict)"(reference=w1166, error in=w1165) -> (reference out=w1168:refnum<vi>, error out=w1167:errorcluster, "Value"=w1164:bool)
        n808 = Close Reference(reference=w1168, error in (no error)=w1167) -> (error out=w1162:errorcluster)
        n809 = case shown="True" w1164 {
          tunnel: w1163 -> [_ w1170]
          tunnel: w1162 -> [w1169 w1178]
          tunnel: [w1169 w1177] -> w1161
          frame False {
          }
          frame True {
            w1180 = FALSE ("Value")
            n810 = Unbundle By Name(w1170) -> ("Loading.SSP 0.3"=w1181:refnum<vi>)
            n811 = Unbundle By Name(w1170) -> ("Loading.SSP 0.5"=w1186:refnum<vi>)
            n812 = Unbundle By Name(w1170) -> ("Loading.Enter the Load  (N)"=w1176:refnum<vi>)
            n813 = property class="Bool (strict)"(reference=w1181, "Value"=w1180) -> (reference out=w1183:refnum<vi>, error out=w1182:errorcluster)  [unwired: 1 in]
            n814 = property class="Bool (strict)"(reference=w1186, "Value"=w1180) -> (reference out=w1184:refnum<vi>, error out=w1185:errorcluster)  [unwired: 1 in]
            n815 = property class="DigNum (strict)"(reference=w1176, "Minimum"=200.0 ("Data Entry Limits:Minimum"), "Maximum"=500.0 ("Data Entry Limits:Maximum"), "Increment"=0.1 ("Data Entry Limits:Increment")) -> (reference out=w1174:refnum<vi>, error out=w1175:errorcluster)  [unwired: 1 in]
            n816 = call "DATA ENCRYPT STRING FILE WRITE.vi"("error in (no error)"=w1178, "User Action"="User selected 0.75 SSP", "main ref"=w1170) -> ("error out"=w1177:errorcluster)  [unwired: 6 in, 1 out]
            n817 = Close Reference(reference=w1183, error in (no error)=w1182) -> ()  [unwired: 1 out]
            n818 = Close Reference(reference=w1184, error in (no error)=w1185) -> ()  [unwired: 1 out]
            n819 = Close Reference(reference=w1174, error in (no error)=w1175) -> ()  [unwired: 1 out]
          }
        }
      }
      frame "LHBack" {
        # "Back to Configure"
        n820 = Unbundle By Name(w1187) -> ("Main Home Screen.GUI"=w1193:refnum<vi>)
        n821 = Unbundle By Name(w1187) -> ("Main Home Screen.MainPage"=w1189:refnum<vi>)
        n822 = property class="TabCtl (strict)"(reference=w1189, "Value"=T5."HOME") -> (reference out=w1191:refnum<vi>, error out=w1190:errorcluster)  [unwired: 1 in]
        n823 = property class="TabCtl (strict)"(reference=w1193, "Value"=T4."Setup") -> (reference out=w1195:refnum<vi>, error out=w1194:errorcluster)  [unwired: 1 in]
        n824 = Close Reference(reference=w1191, error in (no error)=w1190) -> ()  [unwired: 1 out]
        n825 = Close Reference(reference=w1195, error in (no error)=w1194) -> ()  [unwired: 1 out]
        n826 = call "DATA ENCRYPT STRING FILE WRITE.vi"("error in (no error)"=w1196, "User Action"="User selected Back to Configure", "main ref"=w1187) -> ("error out"=w1197:errorcluster)  [unwired: 6 in, 1 out]
      }
      frame "MMBack" {
        # "Back to Configure"
        n827 = Unbundle By Name(w1199) -> ("Main Home Screen.GUI"=w1205:refnum<vi>)
        n828 = Unbundle By Name(w1199) -> ("Main Home Screen.MainPage"=w1201:refnum<vi>)
        n829 = property class="TabCtl (strict)"(reference=w1201, "Value"=T5."HOME") -> (reference out=w1203:refnum<vi>, error out=w1202:errorcluster)  [unwired: 1 in]
        n830 = property class="TabCtl (strict)"(reference=w1205, "Value"=T4."Load Head") -> (reference out=w1207:refnum<vi>, error out=w1206:errorcluster)  [unwired: 1 in]
        n831 = Close Reference(reference=w1203, error in (no error)=w1202) -> ()  [unwired: 1 out]
        n832 = Close Reference(reference=w1207, error in (no error)=w1206) -> ()  [unwired: 1 out]
        n833 = call "DATA ENCRYPT STRING FILE WRITE.vi"("error in (no error)"=w1208, "User Action"="User selected Back to Load Selection", "main ref"=w1199) -> ("error out"=w1209:errorcluster)  [unwired: 6 in, 1 out]
      }
      frame "LHNext" {
        w1241 = FALSE ("Visible")
        n834 = Unbundle By Name(w1211) -> ("Motion Module.HomeRot"=w1247:refnum<vi>)
        n835 = Unbundle By Name(w1211) -> ("Motion Module.HomeScratch"=w1242:refnum<vi>)
        n836 = Unbundle By Name(w1211) -> ("Motion Module.PlaceModule"=w1240:refnum<vi>)
        n837 = Unbundle By Name(w1211) -> ("Motion Module.Motion Mode:"=w1233:refnum<vi>)
        n838 = Unbundle By Name(w1211) -> ("Motion Module.Motion Direction:  3"=w1232:refnum<vi>)
        n839 = Unbundle By Name(w1211) -> ("Motion Module.Wear Track Diameter (mm)"=w1226:refnum<vi>)
        n840 = Unbundle By Name(w1211) -> ("Motion Module.Set WTD"=w1223:refnum<vi>)
        n841 = Unbundle By Name(w1211) -> ("Motion Module.Rotary Module Selection"=w1217:refnum<vi>)
        n842 = call "DATA ENCRYPT STRING FILE WRITE.vi"("error in (no error)"=w1256, "User Action"="User selected Select Module", "main ref"=w1211) -> ("error out"=w1220:errorcluster)  [unwired: 6 in, 1 out]
        n843 = property class="TabCtl (strict)"(reference=w1217, "Visible"=FALSE) -> (reference out=w1216:refnum<vi>, error out=w1218:errorcluster)  [unwired: 1 in]
        n844 = property class="Bool (strict)"(reference=w1247, error in=w1220, "Visible"=w1241) -> (reference out=w1245:refnum<vi>, error out=w1246:errorcluster)
        n845 = property class="Bool (strict)"(reference=w1242, error in=w1220, "Visible"=w1241) -> (reference out=w1244:refnum<vi>, error out=w1243:errorcluster)
        n846 = property class="Bool (strict)"(reference=w1240, error in=w1220, "Visible"=TRUE) -> (reference out=w1238:refnum<vi>, error out=w1239:errorcluster)
        n847 = property class="Ring (strict)"(reference=w1233, error in=w1220, "Visible"=FALSE) -> (reference out=w1235:refnum<vi>, error out=w1234:errorcluster)
        n848 = property class="Ring (strict)"(reference=w1232, error in=w1220, "Visible"=FALSE) -> (reference out=w1229:refnum<vi>, error out=w1231:errorcluster)
        n849 = property class="DigNum (strict)"(reference=w1226, "Visible"=FALSE) -> (reference out=w1225:refnum<vi>, error out=w1227:errorcluster)  [unwired: 1 in]
        n850 = property class="Bool (strict)"(reference=w1223, "Visible"=FALSE) -> (reference out=w1224:refnum<vi>, error out=w1222:errorcluster)  [unwired: 1 in]
        n851 = Close Reference(reference=w1245, error in (no error)=w1246) -> ()  [unwired: 1 out]
        n852 = Close Reference(reference=w1244, error in (no error)=w1243) -> ()  [unwired: 1 out]
        n853 = Close Reference(reference=w1238, error in (no error)=w1239) -> ()  [unwired: 1 out]
        n854 = Close Reference(reference=w1235, error in (no error)=w1234) -> ()  [unwired: 1 out]
        n855 = Close Reference(reference=w1229, error in (no error)=w1231) -> ()  [unwired: 1 out]
        n856 = Close Reference(reference=w1225, error in (no error)=w1227) -> ()  [unwired: 1 out]
        n857 = Close Reference(reference=w1216, error in (no error)=w1218) -> ()  [unwired: 1 out]
        n858 = Close Reference(reference=w1224, error in (no error)=w1222) -> ()  [unwired: 1 out]
        n859 = Unbundle By Name(w1211) -> ("Motion Module.M3 Image"=w1215:refnum<vi>)
        n860 = Unbundle By Name(w1211) -> ("Main Home Screen.GUI"=w1253:refnum<vi>)
        n861 = Unbundle By Name(w1211) -> ("Main Home Screen.MainPage"=w1249:refnum<vi>)
        n862 = property class="TabCtl (strict)"(reference=w1215, "Value"=enum32{"Page 1", "Page 2"}."Page 2") -> (reference out=w1213:refnum<vi>, error out=w1214:errorcluster)  [unwired: 1 in]
        n863 = property class="TabCtl (strict)"(reference=w1249, "Value"=T5."HOME") -> (reference out=w1251:refnum<vi>, error out=w1250:errorcluster)  [unwired: 1 in]
        n864 = property class="TabCtl (strict)"(reference=w1253, "Value"=T4."Motion Module") -> (reference out=w1255:refnum<vi>, error out=w1254:errorcluster)  [unwired: 1 in]
        n865 = Close Reference(reference=w1213, error in (no error)=w1214) -> ()  [unwired: 1 out]
        n866 = Close Reference(reference=w1251, error in (no error)=w1250) -> ()  [unwired: 1 out]
        n867 = Close Reference(reference=w1255, error in (no error)=w1254) -> ()  [unwired: 1 out]
      }
      frame "Rot Ver" {
        # "Rot Ver"
        n868 = Unbundle By Name(w1260) -> ("Motion Module.Rot Ver"=w1259:refnum<vi>)
        n869 = property class="Bool (strict)"(reference=w1259) -> (reference out=w1262:refnum<vi>, error out=w1261:errorcluster, "Value"=w1258:bool)  [unwired: 1 in]
        n870 = Close Reference(reference=w1262, error in (no error)=w1261) -> ()  [unwired: 1 out]
        n871 = case shown="True" w1258 {
          tunnel: w1276 -> [w1311 w1346]
          tunnel: [w1283 w1346] -> w1267
          tunnel: w1260 -> [w1277 w1313]
          frame True {
            n872 = Unbundle By Name(w1277) -> ("Motion Module.HomeRot"=w1310:refnum<vi>)
            n873 = Unbundle By Name(w1277) -> ("Motion Module.HomeScratch"=w1305:refnum<vi>)
            n874 = Unbundle By Name(w1277) -> ("Motion Module.PlaceModule"=w1303:refnum<vi>)
            n875 = Unbundle By Name(w1277) -> ("Motion Module.Motion Mode:"=w1296:refnum<vi>)
            n876 = Unbundle By Name(w1277) -> ("Motion Module.Motion Direction:  3"=w1295:refnum<vi>)
            n877 = Unbundle By Name(w1277) -> ("Motion Module.Wear Track Diameter (mm)"=w1289:refnum<vi>)
            n878 = Unbundle By Name(w1277) -> ("Motion Module.Set WTD"=w1286:refnum<vi>)
            n879 = Unbundle By Name(w1277) -> ("Motion Module.Rotary Module Selection"=w1280:refnum<vi>)
            n880 = call "DATA ENCRYPT STRING FILE WRITE.vi"("error in (no error)"=w1311, "User Action"="User selected Rot Vertical Module", "main ref"=w1277) -> ("error out"=w1283:errorcluster)  [unwired: 6 in, 1 out]
            n881 = property class="TabCtl (strict)"(reference=w1280, "Visible"=TRUE) -> (reference out=w1279:refnum<vi>, error out=w1281:errorcluster)  [unwired: 1 in]
            n882 = property class="Bool (strict)"(reference=w1310, error in=w1283, "Visible"=TRUE) -> (reference out=w1308:refnum<vi>, error out=w1309:errorcluster)
            n883 = property class="Bool (strict)"(reference=w1305, error in=w1283, "Visible"=FALSE) -> (reference out=w1307:refnum<vi>, error out=w1306:errorcluster)
            n884 = property class="Bool (strict)"(reference=w1303, error in=w1283, "Visible"=FALSE) -> (reference out=w1301:refnum<vi>, error out=w1302:errorcluster)
            n885 = property class="Ring (strict)"(reference=w1296, error in=w1283, "Visible"=TRUE) -> (reference out=w1298:refnum<vi>, error out=w1297:errorcluster)
            n886 = property class="Ring (strict)"(reference=w1295, error in=w1283, "Visible"=TRUE) -> (reference out=w1292:refnum<vi>, error out=w1294:errorcluster)
            n887 = property class="DigNum (strict)"(reference=w1289, "Visible"=TRUE) -> (reference out=w1288:refnum<vi>, error out=w1290:errorcluster)  [unwired: 1 in]
            n888 = property class="Bool (strict)"(reference=w1286, "Visible"=TRUE) -> (reference out=w1287:refnum<vi>, error out=w1285:errorcluster)  [unwired: 1 in]
            n889 = Close Reference(reference=w1308, error in (no error)=w1309) -> ()  [unwired: 1 out]
            n890 = Close Reference(reference=w1307, error in (no error)=w1306) -> ()  [unwired: 1 out]
            n891 = Close Reference(reference=w1301, error in (no error)=w1302) -> ()  [unwired: 1 out]
            n892 = Close Reference(reference=w1298, error in (no error)=w1297) -> ()  [unwired: 1 out]
            n893 = Close Reference(reference=w1292, error in (no error)=w1294) -> ()  [unwired: 1 out]
            n894 = Close Reference(reference=w1288, error in (no error)=w1290) -> ()  [unwired: 1 out]
            n895 = Close Reference(reference=w1279, error in (no error)=w1281) -> ()  [unwired: 1 out]
            n896 = Close Reference(reference=w1287, error in (no error)=w1285) -> ()  [unwired: 1 out]
          }
          frame False {
            n897 = Unbundle By Name(w1313) -> ("Motion Module.HomeRot"=w1345:refnum<vi>)
            n898 = Unbundle By Name(w1313) -> ("Motion Module.HomeScratch"=w1340:refnum<vi>)
            n899 = Unbundle By Name(w1313) -> ("Motion Module.PlaceModule"=w1338:refnum<vi>)
            n900 = Unbundle By Name(w1313) -> ("Motion Module.Motion Mode:"=w1331:refnum<vi>)
            n901 = Unbundle By Name(w1313) -> ("Motion Module.Motion Direction:  3"=w1330:refnum<vi>)
            n902 = Unbundle By Name(w1313) -> ("Motion Module.Wear Track Diameter (mm)"=w1324:refnum<vi>)
            n903 = Unbundle By Name(w1313) -> ("Motion Module.Set WTD"=w1321:refnum<vi>)
            n904 = Unbundle By Name(w1313) -> ("Motion Module.Rotary Module Selection"=w1316:refnum<vi>)
            n905 = property class="TabCtl (strict)"(reference=w1316, "Visible"=FALSE) -> (reference out=w1315:refnum<vi>, error out=w1317:errorcluster)  [unwired: 1 in]
            n906 = property class="Bool (strict)"(reference=w1345, error in=w1346, "Visible"=FALSE) -> (reference out=w1343:refnum<vi>, error out=w1344:errorcluster)
            n907 = property class="Bool (strict)"(reference=w1340, error in=w1346, "Visible"=FALSE) -> (reference out=w1342:refnum<vi>, error out=w1341:errorcluster)
            n908 = property class="Bool (strict)"(reference=w1338, error in=w1346, "Visible"=TRUE) -> (reference out=w1336:refnum<vi>, error out=w1337:errorcluster)
            n909 = property class="Ring (strict)"(reference=w1331, error in=w1346, "Visible"=FALSE) -> (reference out=w1333:refnum<vi>, error out=w1332:errorcluster)
            n910 = property class="Ring (strict)"(reference=w1330, error in=w1346, "Visible"=FALSE) -> (reference out=w1327:refnum<vi>, error out=w1329:errorcluster)
            n911 = property class="DigNum (strict)"(reference=w1324, "Visible"=FALSE) -> (reference out=w1323:refnum<vi>, error out=w1325:errorcluster)  [unwired: 1 in]
            n912 = property class="Bool (strict)"(reference=w1321, "Visible"=FALSE) -> (reference out=w1322:refnum<vi>, error out=w1320:errorcluster)  [unwired: 1 in]
            n913 = Close Reference(reference=w1343, error in (no error)=w1344) -> ()  [unwired: 1 out]
            n914 = Close Reference(reference=w1342, error in (no error)=w1341) -> ()  [unwired: 1 out]
            n915 = Close Reference(reference=w1336, error in (no error)=w1337) -> ()  [unwired: 1 out]
            n916 = Close Reference(reference=w1333, error in (no error)=w1332) -> ()  [unwired: 1 out]
            n917 = Close Reference(reference=w1327, error in (no error)=w1329) -> ()  [unwired: 1 out]
            n918 = Close Reference(reference=w1323, error in (no error)=w1325) -> ()  [unwired: 1 out]
            n919 = Close Reference(reference=w1315, error in (no error)=w1317) -> ()  [unwired: 1 out]
            n920 = Close Reference(reference=w1322, error in (no error)=w1320) -> ()  [unwired: 1 out]
          }
        }
        n921 = Unbundle By Name(w1260) -> ("Motion Module.M3 Image"=w1266:refnum<vi>)
        n922 = Unbundle By Name(w1260) -> ("Main Home Screen.GUI"=w1273:refnum<vi>)
        n923 = Unbundle By Name(w1260) -> ("Main Home Screen.MainPage"=w1269:refnum<vi>)
        n924 = property class="TabCtl (strict)"(reference=w1266, "Value"=enum32{"Page 1", "Page 2"}."Page 1") -> (reference out=w1264:refnum<vi>, error out=w1265:errorcluster)  [unwired: 1 in]
        n925 = property class="TabCtl (strict)"(reference=w1269, "Value"=T5."HOME") -> (reference out=w1271:refnum<vi>, error out=w1270:errorcluster)  [unwired: 1 in]
        n926 = property class="TabCtl (strict)"(reference=w1273, "Value"=T4."Motion Module") -> (reference out=w1275:refnum<vi>, error out=w1274:errorcluster)  [unwired: 1 in]
        n927 = Close Reference(reference=w1264, error in (no error)=w1265) -> ()  [unwired: 1 out]
        n928 = Close Reference(reference=w1271, error in (no error)=w1270) -> ()  [unwired: 1 out]
        n929 = Close Reference(reference=w1275, error in (no error)=w1274) -> ()  [unwired: 1 out]
      }
      frame "Scratch" {
        n930 = Unbundle By Name(w1348) -> ("Motion Module.Scratch"=w1349:refnum<vi>)
        n931 = property class="Bool (strict)"(reference=w1349) -> (reference out=w1351:refnum<vi>, error out=w1350:errorcluster, "Value"=w1347:bool)  [unwired: 1 in]
        n932 = Close Reference(reference=w1351, error in (no error)=w1350) -> ()  [unwired: 1 out]
        n933 = case shown="True" w1347 {
          tunnel: w1365 -> [w1400 w1435]
          tunnel: [w1372 w1435] -> w1356
          tunnel: w1348 -> [w1366 w1402]
          frame True {
            n934 = Unbundle By Name(w1366) -> ("Motion Module.HomeRot"=w1399:refnum<vi>)
            n935 = Unbundle By Name(w1366) -> ("Motion Module.HomeScratch"=w1394:refnum<vi>)
            n936 = Unbundle By Name(w1366) -> ("Motion Module.PlaceModule"=w1392:refnum<vi>)
            n937 = Unbundle By Name(w1366) -> ("Motion Module.Motion Mode:"=w1385:refnum<vi>)
            n938 = Unbundle By Name(w1366) -> ("Motion Module.Motion Direction:  3"=w1384:refnum<vi>)
            n939 = Unbundle By Name(w1366) -> ("Motion Module.Wear Track Diameter (mm)"=w1378:refnum<vi>)
            n940 = Unbundle By Name(w1366) -> ("Motion Module.Set WTD"=w1375:refnum<vi>)
            n941 = Unbundle By Name(w1366) -> ("Motion Module.Rotary Module Selection"=w1369:refnum<vi>)
            n942 = call "DATA ENCRYPT STRING FILE WRITE.vi"("error in (no error)"=w1400, "User Action"="User selected Scratch Module", "main ref"=w1366) -> ("error out"=w1372:errorcluster)  [unwired: 6 in, 1 out]
            n943 = property class="TabCtl (strict)"(reference=w1369, "Visible"=FALSE) -> (reference out=w1368:refnum<vi>, error out=w1370:errorcluster)  [unwired: 1 in]
            n944 = property class="Bool (strict)"(reference=w1399, error in=w1372, "Visible"=FALSE) -> (reference out=w1397:refnum<vi>, error out=w1398:errorcluster)
            n945 = property class="Bool (strict)"(reference=w1394, error in=w1372, "Visible"=TRUE) -> (reference out=w1396:refnum<vi>, error out=w1395:errorcluster)
            n946 = property class="Bool (strict)"(reference=w1392, error in=w1372, "Visible"=FALSE) -> (reference out=w1390:refnum<vi>, error out=w1391:errorcluster)
            n947 = property class="Ring (strict)"(reference=w1385, error in=w1372, "Visible"=FALSE) -> (reference out=w1387:refnum<vi>, error out=w1386:errorcluster)
            n948 = property class="Ring (strict)"(reference=w1384, error in=w1372, "Visible"=FALSE) -> (reference out=w1381:refnum<vi>, error out=w1383:errorcluster)
            n949 = property class="DigNum (strict)"(reference=w1378, "Visible"=FALSE) -> (reference out=w1377:refnum<vi>, error out=w1379:errorcluster)  [unwired: 1 in]
            n950 = property class="Bool (strict)"(reference=w1375, "Visible"=FALSE) -> (reference out=w1376:refnum<vi>, error out=w1374:errorcluster)  [unwired: 1 in]
            n951 = Close Reference(reference=w1397, error in (no error)=w1398) -> ()  [unwired: 1 out]
            n952 = Close Reference(reference=w1396, error in (no error)=w1395) -> ()  [unwired: 1 out]
            n953 = Close Reference(reference=w1390, error in (no error)=w1391) -> ()  [unwired: 1 out]
            n954 = Close Reference(reference=w1387, error in (no error)=w1386) -> ()  [unwired: 1 out]
            n955 = Close Reference(reference=w1381, error in (no error)=w1383) -> ()  [unwired: 1 out]
            n956 = Close Reference(reference=w1377, error in (no error)=w1379) -> ()  [unwired: 1 out]
            n957 = Close Reference(reference=w1368, error in (no error)=w1370) -> ()  [unwired: 1 out]
            n958 = Close Reference(reference=w1376, error in (no error)=w1374) -> ()  [unwired: 1 out]
          }
          frame False {
            n959 = Unbundle By Name(w1402) -> ("Motion Module.HomeRot"=w1434:refnum<vi>)
            n960 = Unbundle By Name(w1402) -> ("Motion Module.HomeScratch"=w1429:refnum<vi>)
            n961 = Unbundle By Name(w1402) -> ("Motion Module.PlaceModule"=w1427:refnum<vi>)
            n962 = Unbundle By Name(w1402) -> ("Motion Module.Motion Mode:"=w1420:refnum<vi>)
            n963 = Unbundle By Name(w1402) -> ("Motion Module.Motion Direction:  3"=w1419:refnum<vi>)
            n964 = Unbundle By Name(w1402) -> ("Motion Module.Wear Track Diameter (mm)"=w1413:refnum<vi>)
            n965 = Unbundle By Name(w1402) -> ("Motion Module.Set WTD"=w1410:refnum<vi>)
            n966 = Unbundle By Name(w1402) -> ("Motion Module.Rotary Module Selection"=w1405:refnum<vi>)
            n967 = property class="TabCtl (strict)"(reference=w1405, "Visible"=FALSE) -> (reference out=w1404:refnum<vi>, error out=w1406:errorcluster)  [unwired: 1 in]
            n968 = property class="Bool (strict)"(reference=w1434, error in=w1435, "Visible"=FALSE) -> (reference out=w1432:refnum<vi>, error out=w1433:errorcluster)
            n969 = property class="Bool (strict)"(reference=w1429, error in=w1435, "Visible"=FALSE) -> (reference out=w1431:refnum<vi>, error out=w1430:errorcluster)
            n970 = property class="Bool (strict)"(reference=w1427, error in=w1435, "Visible"=TRUE) -> (reference out=w1425:refnum<vi>, error out=w1426:errorcluster)
            n971 = property class="Ring (strict)"(reference=w1420, error in=w1435, "Visible"=FALSE) -> (reference out=w1422:refnum<vi>, error out=w1421:errorcluster)
            n972 = property class="Ring (strict)"(reference=w1419, error in=w1435, "Visible"=FALSE) -> (reference out=w1416:refnum<vi>, error out=w1418:errorcluster)
            n973 = property class="DigNum (strict)"(reference=w1413, "Visible"=FALSE) -> (reference out=w1412:refnum<vi>, error out=w1414:errorcluster)  [unwired: 1 in]
            n974 = property class="Bool (strict)"(reference=w1410, "Visible"=FALSE) -> (reference out=w1411:refnum<vi>, error out=w1409:errorcluster)  [unwired: 1 in]
            n975 = Close Reference(reference=w1432, error in (no error)=w1433) -> ()  [unwired: 1 out]
            n976 = Close Reference(reference=w1431, error in (no error)=w1430) -> ()  [unwired: 1 out]
            n977 = Close Reference(reference=w1425, error in (no error)=w1426) -> ()  [unwired: 1 out]
            n978 = Close Reference(reference=w1422, error in (no error)=w1421) -> ()  [unwired: 1 out]
            n979 = Close Reference(reference=w1416, error in (no error)=w1418) -> ()  [unwired: 1 out]
            n980 = Close Reference(reference=w1412, error in (no error)=w1414) -> ()  [unwired: 1 out]
            n981 = Close Reference(reference=w1404, error in (no error)=w1406) -> ()  [unwired: 1 out]
            n982 = Close Reference(reference=w1411, error in (no error)=w1409) -> ()  [unwired: 1 out]
          }
        }
        n983 = Unbundle By Name(w1348) -> ("Main Home Screen.GUI"=w1362:refnum<vi>)
        n984 = Unbundle By Name(w1348) -> ("Main Home Screen.MainPage"=w1358:refnum<vi>)
        n985 = Unbundle By Name(w1348) -> ("Motion Module.M3 Image"=w1355:refnum<vi>)
        n986 = property class="TabCtl (strict)"(reference=w1358, "Value"=T5."HOME") -> (reference out=w1360:refnum<vi>, error out=w1359:errorcluster)  [unwired: 1 in]
        n987 = property class="TabCtl (strict)"(reference=w1355, "Value"=enum32{"Page 1", "Page 2"}."Page 2") -> (reference out=w1353:refnum<vi>, error out=w1354:errorcluster)  [unwired: 1 in]
        n988 = property class="TabCtl (strict)"(reference=w1362, "Value"=T4."Motion Module") -> (reference out=w1364:refnum<vi>, error out=w1363:errorcluster)  [unwired: 1 in]
        n989 = Close Reference(reference=w1360, error in (no error)=w1359) -> ()  [unwired: 1 out]
        n990 = Close Reference(reference=w1353, error in (no error)=w1354) -> ()  [unwired: 1 out]
        n991 = Close Reference(reference=w1364, error in (no error)=w1363) -> ()  [unwired: 1 out]
      }
      frame "Motion Mode:" {
        n992 = Unbundle By Name(w1436) -> ("Motion Module.Motion Mode:"=w1438:refnum<vi>)
        n993 = property class="Ring (strict)"(reference=w1438) -> (reference out=w1440:refnum<vi>, error out=w1439:errorcluster, "Value"=w1437:u16)  [unwired: 1 in]
        n994 = Close Reference(reference=w1440, error in (no error)=w1439) -> ()  [unwired: 1 out]
        n995 = case shown="3" w1437 {
          tunnel: w1442 -> [w1451 w1460 w1469 w1478]
          tunnel: [w1450 w1459 w1468 w1477] -> w1441
          tunnel: w1436 -> [w1449 w1458 w1467 w1476]
          tunnel: w1436 -> [w1444 w1453 w1462 w1471]
          frame 0, Default {
            n996 = Unbundle By Name(w1444) -> ("Motion Module.Rotary Module Selection"=w1445:refnum<vi>)
            n997 = property class="TabCtl (strict)"(reference=w1445, "Value"=T7."Uniform Rotation") -> (reference out=w1447:refnum<vi>, error out=w1446:errorcluster)  [unwired: 1 in]
            n998 = Close Reference(reference=w1447, error in (no error)=w1446) -> ()  [unwired: 1 out]
            n999 = call "DATA ENCRYPT STRING FILE WRITE.vi"("error in (no error)"=w1451, "User Action"="User Selected Uniform Rotation", "main ref"=w1449) -> ("error out"=w1450:errorcluster)  [unwired: 6 in, 1 out]
          }
          frame 1 {
            n1000 = Unbundle By Name(w1453) -> ("Motion Module.Rotary Module Selection"=w1454:refnum<vi>)
            n1001 = property class="TabCtl (strict)"(reference=w1454, "Value"=T7."Angular Oscillation") -> (reference out=w1456:refnum<vi>, error out=w1455:errorcluster)  [unwired: 1 in]
            n1002 = Close Reference(reference=w1456, error in (no error)=w1455) -> ()  [unwired: 1 out]
            n1003 = call "DATA ENCRYPT STRING FILE WRITE.vi"("error in (no error)"=w1460, "User Action"="User Selected Angular Oscillation", "main ref"=w1458) -> ("error out"=w1459:errorcluster)  [unwired: 6 in, 1 out]
          }
          frame 2 {
            n1004 = Unbundle By Name(w1462) -> ("Motion Module.Rotary Module Selection"=w1463:refnum<vi>)
            n1005 = property class="TabCtl (strict)"(reference=w1463, "Value"=T7."Speed Ramp") -> (reference out=w1465:refnum<vi>, error out=w1464:errorcluster)  [unwired: 1 in]
            n1006 = Close Reference(reference=w1465, error in (no error)=w1464) -> ()  [unwired: 1 out]
            n1007 = call "DATA ENCRYPT STRING FILE WRITE.vi"("error in (no error)"=w1469, "User Action"="User Selected Ramp Mode", "main ref"=w1467) -> ("error out"=w1468:errorcluster)  [unwired: 6 in, 1 out]
          }
          frame 3 {
            n1008 = Unbundle By Name(w1471) -> ("Motion Module.Rotary Module Selection"=w1472:refnum<vi>)
            n1009 = property class="TabCtl (strict)"(reference=w1472, "Value"=T7."Speed Step") -> (reference out=w1474:refnum<vi>, error out=w1473:errorcluster)  [unwired: 1 in]
            n1010 = Close Reference(reference=w1474, error in (no error)=w1473) -> ()  [unwired: 1 out]
            n1011 = call "DATA ENCRYPT STRING FILE WRITE.vi"("error in (no error)"=w1478, "User Action"="User Selected Step Mode", "main ref"=w1476) -> ("error out"=w1477:errorcluster)  [unwired: 6 in, 1 out]
          }
        }
      }
      frame "MMNext" {
        n1012 = Unbundle By Name(w1479) -> ("Motion Module.MMNext"=w1486:refnum<vi>)
        n1013 = Unbundle By Name(w1479) -> ("Main Home Screen.GUI"=w1488:refnum<vi>)
        n1014 = property class="TabCtl (strict)"(reference=w1488, "Value"=T4."Environment") -> (reference out=w1490:refnum<vi>, error out=w1489:errorcluster)  [unwired: 1 in]
        n1015 = property class="Bool (strict)"(reference=w1486, "Value"=FALSE) -> (reference out=w1484:refnum<vi>, error out=w1485:errorcluster)  [unwired: 1 in]
        n1016 = Close Reference(reference=w1484, error in (no error)=w1485) -> ()  [unwired: 1 out]
        n1017 = Close Reference(reference=w1490, error in (no error)=w1489) -> ()  [unwired: 1 out]
        n1018 = call "DATA ENCRYPT STRING FILE WRITE.vi"("error in (no error)"=w1481, "User Action"="User Selected SetUp Module", "main ref"=w1479) -> ("error out"=w1480:errorcluster)  [unwired: 6 in, 1 out]
      }
      frame "APBack" {
        n1019 = Unbundle By Name(w1491) -> ("Environmental control.APBack"=w1498:refnum<vi>)
        n1020 = Unbundle By Name(w1491) -> ("Main Home Screen.GUI"=w1500:refnum<vi>)
        n1021 = property class="TabCtl (strict)"(reference=w1500, "Value"=T4."Motion Module") -> (reference out=w1502:refnum<vi>, error out=w1501:errorcluster)  [unwired: 1 in]
        n1022 = property class="Bool (strict)"(reference=w1498, "Value"=FALSE) -> (reference out=w1496:refnum<vi>, error out=w1497:errorcluster)  [unwired: 1 in]
        n1023 = Close Reference(reference=w1496, error in (no error)=w1497) -> ()  [unwired: 1 out]
        n1024 = Close Reference(reference=w1502, error in (no error)=w1501) -> ()  [unwired: 1 out]
        n1025 = call "DATA ENCRYPT STRING FILE WRITE.vi"("error in (no error)"=w1493, "User Action"="User Selected Back to Module", "main ref"=w1491) -> ("error out"=w1492:errorcluster)  [unwired: 6 in, 1 out]
      }
      frame "SNext" {
        w1511 = FALSE ("Value")
        n1026 = Unbundle By Name(w1503) -> ("Main Screen.Start Test"=w1514:refnum<vi>)
        n1027 = Unbundle By Name(w1503) -> ("Main Screen.STOP"=w1513:refnum<vi>)
        n1028 = Unbundle By Name(w1503) -> ("Environmental control.SNext"=w1523:refnum<vi>)
        n1029 = Unbundle By Name(w1503) -> ("Main Home Screen.GUI"=w1525:refnum<vi>)
        n1030 = Unbundle By Name(w1503) -> ("PID.Ramp"=w1506:refnum<vi>)
        n1031 = property class="Bool (strict)"(reference=w1506, "Value"=FALSE) -> (reference out=w1504:refnum<vi>, error out=w1507:errorcluster)  [unwired: 1 in]
        n1032 = property class="Bool (strict)"(reference=w1514, "Visible"=TRUE ("Value"), "Value"=FALSE) -> (reference out=w1509:refnum<vi>, error out=w1515:errorcluster)  [unwired: 1 in]
        n1033 = property class="Bool (strict)"(reference=w1513, "Value"=w1511, "Visible"=w1511) -> (reference out=w1508:refnum<vi>, error out=w1512:errorcluster)  [unwired: 1 in]
        n1034 = property class="TabCtl (strict)"(reference=w1525, "Value"=T4."Begin") -> (reference out=w1527:refnum<vi>, error out=w1526:errorcluster)  [unwired: 1 in]
        n1035 = property class="Bool (strict)"(reference=w1523, "Value"=FALSE) -> (reference out=w1521:refnum<vi>, error out=w1522:errorcluster)  [unwired: 1 in]
        n1036 = Close Reference(reference=w1504, error in (no error)=w1507) -> ()  [unwired: 1 out]
        n1037 = Close Reference(reference=w1509, error in (no error)=w1515) -> ()  [unwired: 1 out]
        n1038 = Close Reference(reference=w1508, error in (no error)=w1512) -> ()  [unwired: 1 out]
        n1039 = Close Reference(reference=w1521, error in (no error)=w1522) -> ()  [unwired: 1 out]
        n1040 = Close Reference(reference=w1527, error in (no error)=w1526) -> ()  [unwired: 1 out]
        n1041 = call "DATA ENCRYPT STRING FILE WRITE.vi"("error in (no error)"=w1518, "User Action"="User Pressed Setup", "main ref"=w1503) -> ("error out"=w1517:errorcluster)  [unwired: 6 in, 1 out]
      }
      frame "Enable Platform" {
        n1042 = Unbundle By Name(w1530) -> ("Heave AND Surge.Sequence ID"=w1532:refnum<vi>)
        n1043 = Unbundle By Name(w1530) -> ("Heave AND Surge.Mode Command"=w1556:refnum<vi>)
        n1044 = Unbundle By Name(w1530) -> ("Heave AND Surge.Distance"=w1553:refnum<vi>)
        n1045 = Unbundle By Name(w1530) -> ("Heave AND Surge.SPEED"=w1550:refnum<vi>)
        n1046 = Unbundle By Name(w1530) -> ("Platform Settings.Enable Platform"=w1564:refnum<vi>)
        n1047 = property class="DigNum (strict)"(reference=w1532, "Value"=u16 0) -> (reference out=w1531:refnum<vi>, error out=w1533:errorcluster)  [unwired: 1 in]
        n1048 = property class="DigNum (strict)"(reference=w1553, error in=w1548, "Value"=sgl 0.0) -> (reference out=w1554:refnum<vi>, error out=w1552:errorcluster)
        n1049 = property class="DigNum (strict)"(reference=w1550, error in=w1548, "Value"=sgl 0.0) -> (reference out=w1551:refnum<vi>, error out=w1549:errorcluster)
        n1050 = property class="DigNum (strict)"(reference=w1556, error in=w1548, "Value"=u8 1) -> (reference out=w1555:refnum<vi>, error out=w1557:errorcluster)
        n1051 = property class="Bool (strict)"(reference=w1564, "Value"=FALSE) -> (reference out=w1562:refnum<vi>, error out=w1563:errorcluster)  [unwired: 1 in]
        n1052 = Close Reference(reference=w1531, error in (no error)=w1533) -> (error out=w1529:errorcluster)
        n1053 = Close Reference(reference=w1554, error in (no error)=w1552) -> (error out=w1545:errorcluster)
        n1054 = Close Reference(reference=w1551, error in (no error)=w1549) -> (error out=w1544:errorcluster)
        n1055 = Close Reference(reference=w1555, error in (no error)=w1557) -> (error out=w1546:errorcluster)
        n1056 = Close Reference(reference=w1562, error in (no error)=w1563) -> ()  [unwired: 1 out]
        n1057 = Merge Errors(w1548, w1546, w1545, w1544, w1529) -> (w1547:errorcluster)
        n1058 = call "DATA ENCRYPT STRING FILE WRITE.vi"("error in (no error)"=w1547, "User Action"="User Pressed Enable Platform", "main ref"=w1530) -> ("error out"=w1559:errorcluster)  [unwired: 6 in, 1 out]
        n1059 = call "HEAVE WRITE FGV.vi"("Enum - Menu"=Heave_Write_enum."WRITE", "error in (no error)"=w1559, "main ref"=w1530) -> ("error out"=w1536:errorcluster)  [unwired: 8 in]
        n1060 = Unbundle By Name(w1530) -> ("Heave AND Surge.Read Heave Temp"=w1540:refnum<vi>)
        n1061 = property class="Bool (strict)"(reference=w1540, error in=w1536, "Value"=TRUE) -> (reference out=w1538:refnum<vi>, error out=w1539:errorcluster)
        n1062 = Close Reference(reference=w1538, error in (no error)=w1539) -> (error out=w1535:errorcluster)
        "HEAVE ENABLE" <- TRUE ("HEAVE ENABLE")
      }
      frame "Heave Up main" {
        n1063 = Unbundle By Name(w1565) -> ("Platform Settings.Heave Up main"=w1575:refnum<vi>)
        n1064 = call "Heave Up Main.vi"("error in (no error)"=w1567, "main ref"=w1565) -> ("error out"=w1566:errorcluster)  [unwired: 9 in]
        n1065 = property class="Bool (strict)"(reference=w1575, "Value"=FALSE) -> (reference out=w1573:refnum<vi>, error out=w1574:errorcluster)  [unwired: 1 in]
        n1066 = Close Reference(reference=w1573, error in (no error)=w1574) -> ()  [unwired: 1 out]
        n1067 = call "DATA ENCRYPT STRING FILE WRITE.vi"("error in (no error)"=w1566, "User Action"="User Pressed Heave UP", "main ref"=w1565) -> ("error out"=w1570:errorcluster)  [unwired: 6 in, 1 out]
        n1068 = call "HEAVE WRITE FGV.vi"("Enum - Menu"=Heave_Write_enum."WRITE", "error in (no error)"=w1570, "main ref"=w1565) -> ("error out"=w1569:errorcluster)  [unwired: 8 in]
      }
      frame "Heave Up MM" {
        n1069 = Unbundle By Name(w1576) -> ("Motion Module.Heave Up MM"=w1586:refnum<vi>)
        n1070 = call "Heave Up Motion Module.vi"("error in (no error)"=w1578, "main ref"=w1576) -> ("error out"=w1577:errorcluster)  [unwired: 9 in]
        n1071 = property class="Bool (strict)"(reference=w1586, "Value"=FALSE) -> (reference out=w1584:refnum<vi>, error out=w1585:errorcluster)  [unwired: 1 in]
        n1072 = Close Reference(reference=w1584, error in (no error)=w1585) -> ()  [unwired: 1 out]
        n1073 = call "DATA ENCRYPT STRING FILE WRITE.vi"("error in (no error)"=w1577, "User Action"="User Pressed Heave UP in Motion Module", "main ref"=w1576) -> ("error out"=w1581:errorcluster)  [unwired: 6 in, 1 out]
        n1074 = call "HEAVE WRITE FGV.vi"("Enum - Menu"=Heave_Write_enum."WRITE", "error in (no error)"=w1581, "main ref"=w1576) -> ("error out"=w1580:errorcluster)  [unwired: 8 in]
      }
      frame "Heave Down Main" {
        n1075 = call "Heave Down Main.vi"("error in (no error)"=w1589, "main ref"=w1587) -> ("error out"=w1588:errorcluster)  [unwired: 9 in]
        n1076 = Unbundle By Name(w1587) -> ("Platform Settings.Heave Down Main"=w1597:refnum<vi>)
        n1077 = property class="Bool (strict)"(reference=w1597, "Value"=FALSE) -> (reference out=w1595:refnum<vi>, error out=w1596:errorcluster)  [unwired: 1 in]
        n1078 = Close Reference(reference=w1595, error in (no error)=w1596) -> ()  [unwired: 1 out]
        n1079 = call "DATA ENCRYPT STRING FILE WRITE.vi"("error in (no error)"=w1588, "User Action"="User Pressed Heave DOWN", "main ref"=w1587) -> ("error out"=w1592:errorcluster)  [unwired: 6 in, 1 out]
        n1080 = call "HEAVE WRITE FGV.vi"("Enum - Menu"=Heave_Write_enum."WRITE", "error in (no error)"=w1592, "main ref"=w1587) -> ("error out"=w1591:errorcluster)  [unwired: 8 in]
      }
      frame "Heave Down MM" {
        n1081 = call "Heave Down Motion Module.vi"("error in (no error)"=w1600, "main ref"=w1598) -> ("error out"=w1599:errorcluster)  [unwired: 9 in]
        n1082 = Unbundle By Name(w1598) -> ("Motion Module.Heave Down MM"=w1608:refnum<vi>)
        n1083 = property class="Bool (strict)"(reference=w1608, "Value"=FALSE) -> (reference out=w1606:refnum<vi>, error out=w1607:errorcluster)  [unwired: 1 in]
        n1084 = Close Reference(reference=w1606, error in (no error)=w1607) -> ()  [unwired: 1 out]
        n1085 = call "DATA ENCRYPT STRING FILE WRITE.vi"("error in (no error)"=w1599, "User Action"="User Pressed Heave DOWN in Motion Module", "main ref"=w1598) -> ("error out"=w1603:errorcluster)  [unwired: 6 in, 1 out]
        n1086 = call "HEAVE WRITE FGV.vi"("Enum - Menu"=Heave_Write_enum."WRITE", "error in (no error)"=w1603, "main ref"=w1598) -> ("error out"=w1602:errorcluster)  [unwired: 8 in]
      }
      frame "Surge Backward Main" {
        n1087 = Unbundle By Name(w1609) -> ("Platform Settings.Surge Backward Main"=w1619:refnum<vi>)
        n1088 = call "Surge Backward Main.vi"("error in (no error)"=w1611, "main ref"=w1609) -> ("error out"=w1610:errorcluster)  [unwired: 9 in]
        n1089 = property class="Bool (strict)"(reference=w1619, "Value"=FALSE) -> (reference out=w1617:refnum<vi>, error out=w1618:errorcluster)  [unwired: 1 in]
        n1090 = Close Reference(reference=w1617, error in (no error)=w1618) -> ()  [unwired: 1 out]
        n1091 = call "DATA ENCRYPT STRING FILE WRITE.vi"("error in (no error)"=w1610, "User Action"="User Pressed Surge Backward", "main ref"=w1609) -> ("error out"=w1614:errorcluster)  [unwired: 6 in, 1 out]
        n1092 = call "HEAVE WRITE FGV.vi"("Enum - Menu"=Heave_Write_enum."WRITE", "error in (no error)"=w1614, "main ref"=w1609) -> ("error out"=w1613:errorcluster)  [unwired: 8 in]
      }
      frame "Surge Forward Main" {
        n1093 = Unbundle By Name(w1620) -> ("Platform Settings.Surge Forward Main"=w1630:refnum<vi>)
        n1094 = call "Surge Forward Main.vi"("error in (no error)"=w1622, "main ref"=w1620) -> ("error out"=w1621:errorcluster)  [unwired: 9 in]
        n1095 = property class="Bool (strict)"(reference=w1630, "Value"=FALSE) -> (reference out=w1628:refnum<vi>, error out=w1629:errorcluster)  [unwired: 1 in]
        n1096 = Close Reference(reference=w1628, error in (no error)=w1629) -> ()  [unwired: 1 out]
        n1097 = call "DATA ENCRYPT STRING FILE WRITE.vi"("error in (no error)"=w1621, "User Action"="User Pressed Surge Forward", "main ref"=w1620) -> ("error out"=w1625:errorcluster)  [unwired: 6 in, 1 out]
        n1098 = call "HEAVE WRITE FGV.vi"("Enum - Menu"=Heave_Write_enum."WRITE", "error in (no error)"=w1625, "main ref"=w1620) -> ("error out"=w1624:errorcluster)  [unwired: 8 in]
      }
      frame "Manual Write Heave & Surge" {
        n1099 = Unbundle By Name(w1631) -> ("Heave AND Surge.Manual Write"=w1640:refnum<vi>)
        n1100 = property class="Bool (strict)"(reference=w1640, "Value"=FALSE) -> (reference out=w1638:refnum<vi>, error out=w1639:errorcluster)  [unwired: 1 in]
        n1101 = Close Reference(reference=w1638, error in (no error)=w1639) -> ()  [unwired: 1 out]
        n1102 = call "DATA ENCRYPT STRING FILE WRITE.vi"("error in (no error)"=w1632, "User Action"="User Pressed Manual Write Heave and Surge", "main ref"=w1631) -> ("error out"=w1635:errorcluster)  [unwired: 6 in, 1 out]
        n1103 = call "HEAVE WRITE FGV.vi"("Enum - Menu"=Heave_Write_enum."WRITE", "error in (no error)"=w1635, "main ref"=w1631) -> ("error out"=w1634:errorcluster)  [unwired: 8 in]
      }
      frame "Load En" {
        n1104 = Unbundle By Name(w1642) -> ("Main Screen.Load En"=w1647:refnum<vi>)
        n1105 = property class="Bool (strict)"(reference=w1647) -> (reference out=w1645:refnum<vi>, error out=w1646:errorcluster, "Value"=w1641:bool)  [unwired: 1 in]
        n1106 = Close Reference(reference=w1645, error in (no error)=w1646) -> ()  [unwired: 1 out]
        n1107 = case shown="False" w1641 {
          tunnel: [w1654 w1661] -> w1643
          tunnel: w1644 -> [w1657 w1660]
          tunnel: w1642 -> [w1656 w1659]
          tunnel: w1642 -> [w1651 _]
          tunnel: w1642 -> [w1650 _]
          frame False {
            n1108 = call "DATA ENCRYPT STRING FILE WRITE.vi"("error in (no error)"=w1657, "User Action"="User Pressed UnLoad on Main Screen", "main ref"=w1656) -> ("error out"=w1653:errorcluster)  [unwired: 6 in, 1 out]
            n1109 = call "Stall Data Flow.vim"("value in"=w1653, "milliseconds to wait"=u32 2000) -> ("value out"=w1649:errorcluster)  [unwired: 1 out]
            n1110 = call "PID UNLOAD.vi"("error in (no error)"=w1649, "main ref"=w1650) -> ("error out"=w1652:errorcluster)  [unwired: 9 in]
            n1111 = call "HEAVE WRITE FGV.vi"("Enum - Menu"=Heave_Write_enum."WRITE", "error in (no error)"=w1652, "main ref"=w1651) -> ("error out"=w1654:errorcluster)  [unwired: 8 in]
          }
          frame True {
            n1112 = call "DATA ENCRYPT STRING FILE WRITE.vi"("error in (no error)"=w1660, "User Action"="User Pressed Load on Main Screen", "main ref"=w1659) -> ("error out"=w1661:errorcluster)  [unwired: 6 in, 1 out]
          }
        }
      }
      frame "apply load" {
        n1113 = Unbundle By Name(w1664) -> ("Main Screen.Load En"=w1669:refnum<vi>)
        n1114 = property class="Bool (strict)"(reference=w1669) -> (reference out=w1667:refnum<vi>, error out=w1668:errorcluster, "Value"=w1663:bool)  [unwired: 1 in]
        n1115 = Close Reference(reference=w1667, error in (no error)=w1668) -> ()  [unwired: 1 out]
        n1116 = case shown="False" w1663 {
          tunnel: [w1676 w1683] -> w1665
          tunnel: w1666 -> [w1679 w1682]
          tunnel: w1664 -> [w1678 w1681]
          tunnel: w1664 -> [w1673 _]
          tunnel: w1664 -> [w1672 _]
          frame False {
            n1117 = call "DATA ENCRYPT STRING FILE WRITE.vi"("error in (no error)"=w1679, "User Action"="User Pressed UnLoad on Service Screen", "main ref"=w1678) -> ("error out"=w1675:errorcluster)  [unwired: 6 in, 1 out]
            n1118 = call "Stall Data Flow.vim"("value in"=w1675, "milliseconds to wait"=u32 2000) -> ("value out"=w1671:errorcluster)  [unwired: 1 out]
            n1119 = call "PID UNLOAD.vi"("error in (no error)"=w1671, "main ref"=w1672) -> ("error out"=w1674:errorcluster)  [unwired: 9 in]
            n1120 = call "HEAVE WRITE FGV.vi"("Enum - Menu"=Heave_Write_enum."WRITE", "error in (no error)"=w1674, "main ref"=w1673) -> ("error out"=w1676:errorcluster)  [unwired: 8 in]
          }
          frame True {
            n1121 = call "DATA ENCRYPT STRING FILE WRITE.vi"("error in (no error)"=w1682, "User Action"="User Pressed Load on Service Screen", "main ref"=w1681) -> ("error out"=w1683:errorcluster)  [unwired: 6 in, 1 out]
          }
        }
      }
      frame "BACK" {
        w1689 = FALSE ("Value")
        n1122 = Unbundle By Name(w1685) -> ("Main Screen.BACK"=w1709:refnum<vi>)
        n1123 = property class="Bool (strict)"(reference=w1709, "Value"=FALSE) -> (reference out=w1707:refnum<vi>, error out=w1708:errorcluster)  [unwired: 1 in]
        n1124 = Close Reference(reference=w1707, error in (no error)=w1708) -> ()  [unwired: 1 out]
        n1125 = call "DATA ENCRYPT STRING FILE WRITE.vi"("error in (no error)"=w1706, "User Action"="User Pressed Back on Main Screen", "main ref"=w1685) -> ("error out"=w1704:errorcluster)  [unwired: 6 in, 1 out]
        n1126 = Unbundle By Name(w1685) -> ("Main Home Screen.MainPage"=w1696:refnum<vi>)
        n1127 = Unbundle By Name(w1685) -> ("Main Screen.Start Test"=w1692:refnum<vi>)
        n1128 = Unbundle By Name(w1685) -> ("Main Screen.STOP"=w1691:refnum<vi>)
        n1129 = Unbundle By Name(w1685) -> ("Main Home Screen.GUI"=w1700:refnum<vi>)
        n1130 = property class="TabCtl (strict)"(reference=w1696, "Value"=T5."HOME") -> (reference out=w1698:refnum<vi>, error out=w1697:errorcluster)  [unwired: 1 in]
        n1131 = property class="TabCtl (strict)"(reference=w1700, "Value"=T4."Setup") -> (reference out=w1702:refnum<vi>, error out=w1701:errorcluster)  [unwired: 1 in]
        n1132 = property class="Bool (strict)"(reference=w1692, "Visible"=TRUE ("Value"), "Value"=FALSE) -> (reference out=w1687:refnum<vi>, error out=w1693:errorcluster)  [unwired: 1 in]
        n1133 = property class="Bool (strict)"(reference=w1691, "Value"=w1689, "Visible"=w1689) -> (reference out=w1686:refnum<vi>, error out=w1690:errorcluster)  [unwired: 1 in]
        n1134 = Close Reference(reference=w1702, error in (no error)=w1701) -> ()  [unwired: 1 out]
        n1135 = Close Reference(reference=w1698, error in (no error)=w1697) -> ()  [unwired: 1 out]
        n1136 = Close Reference(reference=w1687, error in (no error)=w1693) -> ()  [unwired: 1 out]
        n1137 = Close Reference(reference=w1686, error in (no error)=w1690) -> ()  [unwired: 1 out]
      }
      frame "Start Test" {
        n1138 = call "DATA ENCRYPT STRING FILE WRITE.vi"("error in (no error)"=w1733, "User Action"="User Pressed Start Test on Main Screen", "main ref"=w1710) -> ("error out"=w1731:errorcluster)  [unwired: 6 in, 1 out]
        n1139 = Unbundle By Name(w1710) -> ("Loading.Loading Mode"=w1722:refnum<vi>)
        n1140 = property class="Ring (strict)"(reference=w1722) -> (reference out=w1720:refnum<vi>, error out=w1721:errorcluster, "Value"=w1719:u16)  [unwired: 1 in]
        n1141 = Close Reference(reference=w1720, error in (no error)=w1721) -> ()  [unwired: 1 out]
        n1142 = case shown="1" w1719 {
          tunnel: w1710 -> [_ w1735]
          frame 0, Default {
          }
          frame 1 {
            n1143 = Unbundle By Name(w1735) -> ("PID.Ramp"=w1736:refnum<vi>)
            n1144 = property class="Bool (strict)"(reference=w1736, "Value"=TRUE) -> (reference out=w1738:refnum<vi>, error out=w1737:errorcluster)  [unwired: 1 in]
            n1145 = Close Reference(reference=w1738, error in (no error)=w1737) -> ()  [unwired: 1 out]
          }
        }
        n1146 = Unbundle By Name(w1710) -> ("Main Screen.Start Test Temp"=w1730:refnum<vi>)
        n1147 = Unbundle By Name(w1710) -> ("Main Screen.Depthz"=w1723:refnum<vi>)
        n1148 = Unbundle By Name(w1710) -> ("Main Screen.Start Test"=w1713:refnum<vi>)
        n1149 = Unbundle By Name(w1710) -> ("Main Screen.STOP"=w1716:refnum<vi>)
        n1150 = property class="Bool (strict)"(reference=w1723, "Value"=TRUE) -> (reference out=w1725:refnum<vi>, error out=w1724:errorcluster)  [unwired: 1 in]
        n1151 = property class="Bool (strict)"(reference=w1730, "Value"=TRUE) -> (reference out=w1728:refnum<vi>, error out=w1729:errorcluster)  [unwired: 1 in]
        n1152 = property class="Bool (strict)"(reference=w1713, "Visible"=FALSE) -> (reference out=w1711:refnum<vi>, error out=w1712:errorcluster)  [unwired: 1 in]
        n1153 = property class="Bool (strict)"(reference=w1716, "Visible"=TRUE) -> (reference out=w1718:refnum<vi>, error out=w1717:errorcluster)  [unwired: 1 in]
        n1154 = Close Reference(reference=w1725, error in (no error)=w1724) -> ()  [unwired: 1 out]
        n1155 = Close Reference(reference=w1728, error in (no error)=w1729) -> ()  [unwired: 1 out]
        n1156 = Close Reference(reference=w1711, error in (no error)=w1712) -> ()  [unwired: 1 out]
        n1157 = Close Reference(reference=w1718, error in (no error)=w1717) -> ()  [unwired: 1 out]
      }
      frame "STOP" {
        n1158 = call "DATA ENCRYPT STRING FILE WRITE.vi"("error in (no error)"=w1763, "User Action"="User Pressed Stop Test on Main Screen", "main ref"=w1739) -> ("error out"=w1741:errorcluster)  [unwired: 6 in, 1 out]
        n1159 = Unbundle By Name(w1739) -> ("PID.Ramp"=w1756:refnum<vi>)
        n1160 = Unbundle By Name(w1739) -> ("Main Screen.Start Test Temp"=w1761:refnum<vi>)
        n1161 = Unbundle By Name(w1739) -> ("Main Screen.Start Test"=w1749:refnum<vi>)
        n1162 = Unbundle By Name(w1739) -> ("Main Screen.STOP"=w1752:refnum<vi>)
        n1163 = property class="Bool (strict)"(reference=w1756, "Value"=FALSE) -> (reference out=w1746:refnum<vi>, error out=w1757:errorcluster)  [unwired: 1 in]
        n1164 = call "Stall Data Flow.vim"("value in"=w1741, "milliseconds to wait"=u32 2000) -> ("value out"=w1743:errorcluster)  [unwired: 1 out]
        n1165 = property class="Bool (strict)"(reference=w1749, "Visible"=TRUE) -> (reference out=w1747:refnum<vi>, error out=w1748:errorcluster)  [unwired: 1 in]
        n1166 = property class="Bool (strict)"(reference=w1761, "Value"=FALSE) -> (reference out=w1759:refnum<vi>, error out=w1760:errorcluster)  [unwired: 1 in]
        n1167 = property class="Bool (strict)"(reference=w1752, "Visible"=FALSE) -> (reference out=w1754:refnum<vi>, error out=w1753:errorcluster)  [unwired: 1 in]
        n1168 = Close Reference(reference=w1746, error in (no error)=w1757) -> ()  [unwired: 1 out]
        n1169 = Close Reference(reference=w1747, error in (no error)=w1748) -> ()  [unwired: 1 out]
        n1170 = Close Reference(reference=w1759, error in (no error)=w1760) -> ()  [unwired: 1 out]
        n1171 = Close Reference(reference=w1754, error in (no error)=w1753) -> ()  [unwired: 1 out]
        n1172 = call "PID UNLOAD.vi"("error in (no error)"=w1743) -> ("error out"=w1744:errorcluster)  [unwired: 10 in]
        n1173 = call "HEAVE WRITE FGV.vi"("Enum - Menu"=Heave_Write_enum."WRITE", "error in (no error)"=w1744, "main ref"=w1739) -> ("error out"=w1740:errorcluster)  [unwired: 8 in]
      }
      frame "Error" {
        # "#CodeRecommended - If you ever change the name of this \"Error\" message, you'll need to update the name in the Check Loop Error.vi as well."
        # "#CodeRecommended - Consider creating a system for logging errors in some way. These errors are for notification purposes only. Handling of specific errors should be performed in the message frames that generated the error."
        # "Error - Display an error dialog. This message is sent by the \"Error Handler\" VIs at the end of other loops in this application."
        n1174 = Variant To Data(error in=w1770, type=errorcluster {"status"=FALSE, "code"=0, "source"=""} ("error constant"), Variant=w1768) -> (data=w1766:errorcluster, error out=w1765:errorcluster)
        n1175 = call <vilib>:"Simple Error Handler.vi"("error in (no error)"=w1766) -> ()  [unwired: 4 in, 5 out]
        n1176 = Merge Errors(w1765) -> (w1764:errorcluster)
      }
      frame "Confirm Quit" {
        # "#CodeNeeded - If you want to provide an \"Are you sure\" dialog (or some other notification) before the application exits, place that code here. This message is typically sent from a Panel Close? event."
        # "Confirm Quit - Message that can confirm whether or not the user wants to exit the application."
        n1177 = call-poly "Enqueue Message.vi"("Priority Message? (F)"=TRUE, "error in (no error)"=w1781, "Message"="Exit", "Message Queue"=w1778) -> ("error out"=w1779:errorcluster)  [unwired: 6 in, 1 out]
        n1178 = Merge Errors(w1779) -> (w1780:errorcluster)
        n1179 = call "LOAD CELL FGV MAIN.vi"("Enum"=T14."UNINITIAL", "error in (no error)"=w1780, "main ref"=w1771) -> ("error IO"=w1775:errorcluster)  [unwired: 8 in]
        n1180 = call "LOAD CELL FGV MAIN.vi"("Enum"=T14."DELETEHANDLE", "error in (no error)"=w1775, "main ref"=w1771) -> ("error IO"=w1773:errorcluster)  [unwired: 8 in]
      }
      frame "Exit" {
        # "Stop the VI"
        # "Release the message queue reference"
        # "#CodeNeeded - Add any required cleanup code here. Note that if 'Exit' was called as a result of an error, an error dialog will be displayed. Add any custom error handling for an 'Exit' condition here as well."
        # "Exit - Exit the application."
        n1181 = call "Fire User Event - Stop.vi"("User Event - Stop"=w1784) -> ("error out"=w1783:errorcluster)  [unwired: 10 in]
        n1182 = Release Queue(queue=w1789, error in (no error)=w1782) -> (error out=w1786:errorcluster)  [unwired: 1 in, 2 out]
        n1183 = Merge Errors(w1783, w1786) -> (w1785:errorcluster)
      }
      frame Default {
        # "'Default' case only runs if there is a message that isn't defined in any of the other cases.  Output a programming error."
        n1184 = xnode "Error Ring"("parameter 0"=w1790) -> ("error out"=w1791:errorcluster)
      }
    }
    n1185 = call "LAB-IQ Error Handler - Message Handling Loop.vi"("error in (no error)"=w785, "Message Queue"=w787) -> ("dup error in"=w786:errorcluster)  [unwired: 8 in, 1 out]
  }
  n1186 = while {
    shift-right: [w1810] -> _
    shift-left: w14 -> [w1811]
    tunnel: [w1804] -> w24
    tunnel: w23 -> [w1802]
    tunnel: w4 -> [w1801]
    tunnel: w13 -> [w1800]
    stop <- w1809 stop-if-true
    # "Load  Handling Loop"
    n1187 = call "Dequeue Message.vi"("error in (no error)"=w1801, "Message Queue"=w1802) -> ("error out"=w1808:errorcluster, "Message Data"=w1806:variant, "Message"=w1807:string, "dup Message Queue"=w1805:refnum<queue>)  [unwired: 6 in]
    n1188 = case "Message Cases" shown="\"Load Main\"" w1807 {
      selector: w1807 -> [_ _ _ _ _ w1856]
      tunnel: w1805 -> [w1812 w1824 _ w1843 w1855 _]
      tunnel: w1808 -> [w1815 w1822 w1840 w1847 w1849 _]
      tunnel: [w1816 w1825 w1834 w1845 w1851 w1857] -> w1803
      tunnel: w1811 -> [w1814 w1817 w1839 w1846 w1854 w1858]
      tunnel: [w1814 w1817 w1839 w1846 w1854 w1858] -> w1810
      tunnel: [_ _ _ _ TRUE _] -> w1809
      tunnel: w1806 -> [_ _ w1838 _ _ _]
      tunnel: w1800 -> [_ _ _ _ w1848 _]
      frame "init" {
        # "Bundle control references and a sample string value."
        # "Initialize - All initialization work should take place in this message, since other loops can potentially enqueue messages that execute immediately after this one."
        n1189 = call-poly "Enqueue Message.vi"("error in (no error)"=w1815, "Message"="Load Main", "Message Queue"=w1812) -> ("error out"=w1816:errorcluster)  [unwired: 7 in, 1 out]
      }
      frame "Load Main" {
        n1190 = call "LOAD CELL READ.vi"("error in (no error)"=w1822, "main ref"=w1817) -> ("error out"=w1818:errorcluster)  [unwired: 9 in]
        n1191 = Unbundle By Name(w1817) -> ("Main Home Screen.EXIT"=w1823:refnum<vi>)
        n1192 = property class="Bool (strict)"(reference=w1823) -> (reference out=w1820:refnum<vi>, error out=w1821:errorcluster, "Value"=w1819:bool)  [unwired: 1 in]
        n1193 = Close Reference(reference=w1820, error in (no error)=w1821) -> ()  [unwired: 1 out]
        n1194 = case shown="False" w1819 {
          tunnel: [w1828 w1832] -> w1825
          tunnel: w1824 -> [w1827 w1831]
          tunnel: w1818 -> [w1826 w1830]
          frame True {
            n1195 = call-poly "Enqueue Message.vi"("error in (no error)"=w1826, "Message"="Confirm Quit", "Message Queue"=w1827) -> ("error out"=w1828:errorcluster)  [unwired: 7 in, 1 out]
          }
          frame False {
            n1196 = call-poly "Enqueue Message.vi"("error in (no error)"=w1830, "Message"="Load Main", "Message Queue"=w1831) -> ("error out"=w1832:errorcluster)  [unwired: 7 in, 1 out]
          }
        }
      }
      frame "Error" {
        # "#CodeRecommended - If you ever change the name of this \"Error\" message, you'll need to update the name in the Check Loop Error.vi as well."
        # "#CodeRecommended - Consider creating a system for logging errors in some way. These errors are for notification purposes only. Handling of specific errors should be performed in the message frames that generated the error."
        # "Error - Display an error dialog. This message is sent by the \"Error Handler\" VIs at the end of other loops in this application."
        n1197 = Variant To Data(error in=w1840, type=errorcluster {"status"=FALSE, "code"=0, "source"=""} ("error constant"), Variant=w1838) -> (data=w1836:errorcluster, error out=w1835:errorcluster)
        n1198 = call <vilib>:"Simple Error Handler.vi"("error in (no error)"=w1836) -> ()  [unwired: 4 in, 5 out]
        n1199 = Merge Errors(w1835) -> (w1834:errorcluster)
      }
      frame "Confirm Quit" {
        # "#CodeNeeded - If you want to provide an \"Are you sure\" dialog (or some other notification) before the application exits, place that code here. This message is typically sent from a Panel Close? event."
        # "Confirm Quit - Message that can confirm whether or not the user wants to exit the application."
        n1200 = call-poly "Enqueue Message.vi"("Priority Message? (F)"=TRUE, "error in (no error)"=w1847, "Message"="Exit", "Message Queue"=w1843) -> ("error out"=w1844:errorcluster)  [unwired: 6 in, 1 out]
        n1201 = Merge Errors(w1844) -> (w1845:errorcluster)
      }
      frame "Exit" {
        # "Stop the VI"
        # "Release the message queue reference"
        # "#CodeNeeded - Add any required cleanup code here. Note that if 'Exit' was called as a result of an error, an error dialog will be displayed. Add any custom error handling for an 'Exit' condition here as well."
        # "Exit - Exit the application."
        n1202 = call "Fire User Event - Stop.vi"("User Event - Stop"=w1848) -> ("error out"=w1850:errorcluster)  [unwired: 10 in]
        n1203 = Release Queue(queue=w1855, error in (no error)=w1849) -> (error out=w1852:errorcluster)  [unwired: 1 in, 2 out]
        n1204 = Merge Errors(w1850, w1852) -> (w1851:errorcluster)
      }
      frame Default {
        # "'Default' case only runs if there is a message that isn't defined in any of the other cases.  Output a programming error."
        n1205 = xnode "Error Ring"("parameter 0"=w1856) -> ("error out"=w1857:errorcluster)
      }
    }
    n1206 = call "LAB-IQ Error Handler - Message Handling Loop.vi"("error in (no error)"=w1803, "Message Queue"=w1805) -> ("dup error in"=w1804:errorcluster)  [unwired: 8 in, 1 out]
  }
  n1207 = while {
    shift-right: [w1876] -> _
    shift-left: w14 -> [w1877]
    tunnel: [w1870] -> w21
    tunnel: w22 -> [w1868]
    tunnel: w4 -> [w1867]
    tunnel: w13 -> [w1866]
    stop <- w1875 stop-if-true
    # "Sway Motor  Handling Loop"
    n1208 = call "Dequeue Message.vi"("error in (no error)"=w1867, "Message Queue"=w1868) -> ("error out"=w1874:errorcluster, "Message Data"=w1872:variant, "Message"=w1873:string, "dup Message Queue"=w1871:refnum<queue>)  [unwired: 6 in]
    n1209 = case "Message Cases" shown="\"Sway Main\"" w1873 {
      selector: w1873 -> [_ _ _ _ _ w1955]
      tunnel: w1871 -> [w1885 w1913 _ w1942 w1954 _]
      tunnel: w1874 -> [w1887 w1891 w1939 w1946 w1948 _]
      tunnel: [w1888 w1914 w1933 w1944 w1950 w1956] -> w1869
      tunnel: w1877 -> [w1879 w1892 w1938 w1945 w1953 w1957]
      tunnel: [w1879 w1892 w1938 w1945 w1953 w1957] -> w1876
      tunnel: [_ _ _ _ TRUE _] -> w1875
      tunnel: w1872 -> [_ _ w1937 _ _ _]
      tunnel: w1866 -> [_ _ _ _ w1947 _]
      frame "init" {
        # "Bundle control references and a sample string value."
        # "Initialize - All initialization work should take place in this message, since other loops can potentially enqueue messages that execute immediately after this one."
        n1210 = call "SWAY WRITE FGV.vi"("Enum - Menu"=Sway_Write_enum."INIT", "error in (no error)"=w1887, "main ref"=w1879) -> ("error out"=w1884:errorcluster)  [unwired: 8 in]
        n1211 = call "Stall Data Flow.vim"("value in"=w1884, "milliseconds to wait"=u32 1000) -> ("value out"=w1882:errorcluster)  [unwired: 1 out]
        n1212 = call "SWAY WRITE FGV.vi"("Enum - Menu"=Sway_Write_enum."INIT", "error in (no error)"=w1882, "main ref"=w1879) -> ("error out"=w1880:errorcluster)  [unwired: 8 in]
        n1213 = call-poly "Enqueue Message.vi"("error in (no error)"=w1880, "Message"="Sway Main", "Message Queue"=w1885) -> ("error out"=w1888:errorcluster)  [unwired: 7 in, 1 out]
      }
      frame "Sway Main" {
        n1214 = Unbundle By Name(w1892) -> ("Heave AND Surge.Homed"=w1898:refnum<vi>)
        n1215 = Unbundle By Name(w1892) -> ("SWAY.Read SWAY Temp"=w1908:refnum<vi>)
        n1216 = local read "HEAVE ENABLE"() -> (w1902:bool)
        n1217 = property class="DigNum (strict)"(reference=w1898) -> (reference out=w1900:refnum<vi>, error out=w1899:errorcluster, "Value"=w1897:u8)  [unwired: 1 in]
        n1218 = property class="Bool (strict)"(reference=w1908) -> (reference out=w1906:refnum<vi>, error out=w1907:errorcluster, "Value"=w1904:bool)  [unwired: 1 in]
        n1219 = Equal?(x=w1902, y=TRUE) -> (x = y?=w1895:bool)
        n1220 = Close Reference(reference=w1900, error in (no error)=w1899) -> ()  [unwired: 1 out]
        n1221 = Equal?(x=w1897, y=u8 1 ("Value")) -> (x = y?=w1894:bool)
        n1222 = Close Reference(reference=w1906, error in (no error)=w1907) -> ()  [unwired: 1 out]
        n1223 = And(x=w1895, y=w1894) -> (x .and. y?=w1893:bool)
        n1224 = case shown="True" w1893 {
          tunnel: w1892 -> [_ w1919]
          tunnel: w1891 -> [w1915 w1918]
          tunnel: [w1915 w1916] -> w1889
          frame False {
          }
          frame True {
            n1225 = call "SWAY HOME.vi"("error in (no error)"=w1918, "Data Cluster"=w1919) -> ("error out"=w1916:errorcluster)  [unwired: 9 in]
            n1226 = local write "HEAVE ENABLE"(FALSE ("HEAVE ENABLE")) -> ()
          }
        }
        n1227 = case shown="True" w1904 {
          tunnel: w1891 -> [w1920 w1924]
          tunnel: [w1920 w1923] -> w1905
          tunnel: w1892 -> [_ w1922]
          frame False {
          }
          frame True {
            n1228 = call "SWAY READ FGV.vi"("Enum - Menu"=Sway_Right_enum."READ", "error in (no error)"=w1924, "main ref"=w1922) -> ("error out"=w1923:errorcluster)  [unwired: 7 in, 1 out]
          }
        }
        n1229 = Unbundle By Name(w1892) -> ("Main Home Screen.EXIT"=w1912:refnum<vi>)
        n1230 = property class="Bool (strict)"(reference=w1912) -> (reference out=w1910:refnum<vi>, error out=w1911:errorcluster, "Value"=w1909:bool)  [unwired: 1 in]
        n1231 = call <vilib>:"Clear Errors.vi"("error in (no error)"=w1905) -> ("error out"=w1903:errorcluster)  [unwired: 5 in, 1 out]
        n1232 = Merge Errors(w1903, w1889) -> (w1890:errorcluster)
        n1233 = Close Reference(reference=w1910, error in (no error)=w1911) -> ()  [unwired: 1 out]
        n1234 = case shown="False" w1909 {
          tunnel: [w1927 w1931] -> w1914
          tunnel: w1913 -> [w1926 w1930]
          tunnel: w1890 -> [w1925 w1929]
          frame True {
            n1235 = call-poly "Enqueue Message.vi"("error in (no error)"=w1925, "Message"="Confirm Quit", "Message Queue"=w1926) -> ("error out"=w1927:errorcluster)  [unwired: 7 in, 1 out]
          }
          frame False {
            n1236 = call-poly "Enqueue Message.vi"("error in (no error)"=w1929, "Message"="Sway Main", "Message Queue"=w1930) -> ("error out"=w1931:errorcluster)  [unwired: 7 in, 1 out]
          }
        }
      }
      frame "Error" {
        # "#CodeRecommended - If you ever change the name of this \"Error\" message, you'll need to update the name in the Check Loop Error.vi as well."
        # "#CodeRecommended - Consider creating a system for logging errors in some way. These errors are for notification purposes only. Handling of specific errors should be performed in the message frames that generated the error."
        # "Error - Display an error dialog. This message is sent by the \"Error Handler\" VIs at the end of other loops in this application."
        n1237 = Variant To Data(error in=w1939, type=errorcluster {"status"=FALSE, "code"=0, "source"=""} ("error constant"), Variant=w1937) -> (data=w1935:errorcluster, error out=w1934:errorcluster)
        n1238 = call <vilib>:"Simple Error Handler.vi"("error in (no error)"=w1935) -> ()  [unwired: 4 in, 5 out]
        n1239 = Merge Errors(w1934) -> (w1933:errorcluster)
      }
      frame "Confirm Quit" {
        # "#CodeNeeded - If you want to provide an \"Are you sure\" dialog (or some other notification) before the application exits, place that code here. This message is typically sent from a Panel Close? event."
        # "Confirm Quit - Message that can confirm whether or not the user wants to exit the application."
        n1240 = call-poly "Enqueue Message.vi"("Priority Message? (F)"=TRUE, "error in (no error)"=w1946, "Message"="Exit", "Message Queue"=w1942) -> ("error out"=w1943:errorcluster)  [unwired: 6 in, 1 out]
        n1241 = Merge Errors(w1943) -> (w1944:errorcluster)
      }
      frame "Exit" {
        # "Stop the VI"
        # "Release the message queue reference"
        # "#CodeNeeded - Add any required cleanup code here. Note that if 'Exit' was called as a result of an error, an error dialog will be displayed. Add any custom error handling for an 'Exit' condition here as well."
        # "Exit - Exit the application."
        n1242 = call "Fire User Event - Stop.vi"("User Event - Stop"=w1947) -> ("error out"=w1949:errorcluster)  [unwired: 10 in]
        n1243 = Release Queue(queue=w1954, error in (no error)=w1948) -> (error out=w1951:errorcluster)  [unwired: 1 in, 2 out]
        n1244 = Merge Errors(w1949, w1951) -> (w1950:errorcluster)
      }
      frame Default {
        # "'Default' case only runs if there is a message that isn't defined in any of the other cases.  Output a programming error."
        n1245 = xnode "Error Ring"("parameter 0"=w1955) -> ("error out"=w1956:errorcluster)
      }
    }
    n1246 = call "LAB-IQ Error Handler - Message Handling Loop.vi"("error in (no error)"=w1869, "Message Queue"=w1871) -> ("dup error in"=w1870:errorcluster)  [unwired: 8 in, 1 out]
  }
  n1247 = while {
    shift-right: [w1975] -> _
    shift-left: w14 -> [w1976]
    tunnel: [w1969] -> w19
    tunnel: w5 -> [w1967]
    tunnel: w4 -> [w1966]
    tunnel: w13 -> [w1965]
    stop <- w1974 stop-if-true
    # "Heave Motor  Handling Loop"
    n1248 = call "Dequeue Message.vi"("error in (no error)"=w1966, "Message Queue"=w1967) -> ("error out"=w1973:errorcluster, "Message Data"=w1971:variant, "Message"=w1972:string, "dup Message Queue"=w1970:refnum<queue>)  [unwired: 6 in]
    n1249 = case "Message Cases" shown="\"Heave Main\"" w1972 {
      selector: w1972 -> [_ _ _ _ _ w2056]
      tunnel: w1970 -> [w1986 w2013 _ w2044 w2055 _]
      tunnel: w1973 -> [w1979 w2011 w2034 w2047 w2049 _]
      tunnel: [w1980 w2014 w2028 w2035 w2051 w2057] -> w1968
      tunnel: w1976 -> [w1977 w2003 w2033 w2038 w2054 w2058]
      tunnel: [w1977 w2003 w2033 w2038 w2054 w2058] -> w1975
      tunnel: [_ _ _ _ TRUE _] -> w1974
      tunnel: w1971 -> [_ _ w2032 _ _ _]
      tunnel: w1965 -> [_ _ _ _ w2048 _]
      frame "init" {
        # "Initialize - All initialization work should take place in this message, since other loops can potentially enqueue messages that execute immediately after this one."
        n1250 = call "HEAVE WRITE FGV.vi"("Enum - Menu"=Heave_Write_enum."INIT", "error in (no error)"=w1979, "main ref"=w1977) -> ("error out"=w1985:errorcluster)  [unwired: 8 in]
        n1251 = call "Stall Data Flow.vim"("value in"=w1985, "milliseconds to wait"=u32 1000) -> ("value out"=w1983:errorcluster)  [unwired: 1 out]
        n1252 = disable-structure shown="Enabled" {
          disable-tunnel: w1983 -> [w1999 w2000]
          disable-tunnel: [w1998 w2000] -> w1978
          disable-tunnel: w1977 -> [w1997 _]
          frame Disabled {
            n1253 = call "Heave Init.vi"("error in (no error)"=w1999, "main ref"=w1997) -> ("error out"=w1998:errorcluster)  [unwired: 9 in]
          }
          frame Enabled {
          }
        }
        n1254 = disable-structure shown="Enabled" {
          disable-tunnel: [w1990 w1993] -> w1981
          disable-tunnel: w1978 -> [w1989 w1992]
          disable-tunnel: w1977 -> [w1988 _]
          frame Enabled {
            n1255 = call "HEAVE READ FGV.vi"("Enum - Menu"=Heave_Right_enum."INIT", "error in (no error)"=w1989, "main ref"=w1988) -> ("error out"=w1990:errorcluster)  [unwired: 7 in, 1 out]
          }
          frame Disabled {
            n1256 = UDP Open(8:w1992, 9:-1 ("timeout ms (25000)"), 10:"192.168.1.10" ("service name"), 11:u16 8889 ("port")) -> (0:w1993:errorcluster)  [unwired: 1 in, 2 out]
          }
        }
        n1257 = call-poly "Enqueue Message.vi"("error in (no error)"=w1981, "Message"="Heave Main", "Message Queue"=w1986) -> ("error out"=w1980:errorcluster)  [unwired: 7 in, 1 out]
      }
      frame "Heave Main" {
        n1258 = Unbundle By Name(w2003) -> ("Heave AND Surge.Read Heave Temp"=w2006:refnum<vi>)
        n1259 = property class="Bool (strict)"(reference=w2006) -> (reference out=w2004:refnum<vi>, error out=w2005:errorcluster, "Value"=w2002:bool)  [unwired: 1 in]
        n1260 = Close Reference(reference=w2004, error in (no error)=w2005) -> ()  [unwired: 1 out]
        n1261 = case shown="True" w2002 {
          tunnel: w2011 -> [w2015 w2019]
          tunnel: [w2015 w2018] -> w2007
          tunnel: w2003 -> [_ w2017]
          frame False {
          }
          frame True {
            n1262 = call "HEAVE READ FGV.vi"("Enum - Menu"=Heave_Right_enum."READ", "error in (no error)"=w2019, "main ref"=w2017) -> ("error out"=w2018:errorcluster)  [unwired: 7 in, 1 out]
          }
        }
        n1263 = Unbundle By Name(w2003) -> ("Main Home Screen.EXIT"=w2012:refnum<vi>)
        n1264 = property class="Bool (strict)"(reference=w2012) -> (reference out=w2009:refnum<vi>, error out=w2010:errorcluster, "Value"=w2008:bool)  [unwired: 1 in]
        n1265 = call <vilib>:"Clear Errors.vi"("error in (no error)"=w2007) -> ("error out"=w2001:errorcluster)  [unwired: 5 in, 1 out]
        n1266 = Close Reference(reference=w2009, error in (no error)=w2010) -> ()  [unwired: 1 out]
        n1267 = case shown="False" w2008 {
          tunnel: [w2022 w2026] -> w2014
          tunnel: w2013 -> [w2021 w2025]
          tunnel: w2001 -> [w2020 w2024]
          frame True {
            n1268 = call-poly "Enqueue Message.vi"("error in (no error)"=w2020, "Message"="Confirm Quit", "Message Queue"=w2021) -> ("error out"=w2022:errorcluster)  [unwired: 7 in, 1 out]
          }
          frame False {
            n1269 = call-poly "Enqueue Message.vi"("error in (no error)"=w2024, "Message"="Heave Main", "Message Queue"=w2025) -> ("error out"=w2026:errorcluster)  [unwired: 7 in, 1 out]
          }
        }
      }
      frame "Error" {
        # "#CodeRecommended - If you ever change the name of this \"Error\" message, you'll need to update the name in the Check Loop Error.vi as well."
        # "#CodeRecommended - Consider creating a system for logging errors in some way. These errors are for notification purposes only. Handling of specific errors should be performed in the message frames that generated the error."
        # "Error - Display an error dialog. This message is sent by the \"Error Handler\" VIs at the end of other loops in this application."
        n1270 = Variant To Data(error in=w2034, type=errorcluster {"status"=FALSE, "code"=0, "source"=""} ("error constant"), Variant=w2032) -> (data=w2030:errorcluster, error out=w2029:errorcluster)
        n1271 = call <vilib>:"Simple Error Handler.vi"("error in (no error)"=w2030) -> ()  [unwired: 4 in, 5 out]
        n1272 = Merge Errors(w2029) -> (w2028:errorcluster)
      }
      frame "Confirm Quit" {
        # "#CodeNeeded - If you want to provide an \"Are you sure\" dialog (or some other notification) before the application exits, place that code here. This message is typically sent from a Panel Close? event."
        # "Confirm Quit - Message that can confirm whether or not the user wants to exit the application."
        n1273 = call-poly "Enqueue Message.vi"("Priority Message? (F)"=TRUE, "error in (no error)"=w2047, "Message"="Exit", "Message Queue"=w2044) -> ("error out"=w2045:errorcluster)  [unwired: 6 in, 1 out]
        n1274 = Merge Errors(w2045) -> (w2046:errorcluster)
        n1275 = call "HEAVE READ FGV.vi"("Enum - Menu"=Heave_Right_enum."CLOSE", "error in (no error)"=w2046, "main ref"=w2038) -> ("error out"=w2041:errorcluster)  [unwired: 7 in, 1 out]
        n1276 = call <vilib>:"Clear Errors.vi"("error in (no error)"=w2041) -> ("error out"=w2036:errorcluster)  [unwired: 5 in, 1 out]
        n1277 = call "HEAVE WRITE FGV.vi"("Enum - Menu"=Heave_Write_enum."CLOSE", "error in (no error)"=w2036, "main ref"=w2038) -> ("error out"=w2039:errorcluster)  [unwired: 8 in]
        n1278 = call <vilib>:"Clear Errors.vi"("error in (no error)"=w2039) -> ("error out"=w2035:errorcluster)  [unwired: 5 in, 1 out]
      }
      frame "Exit" {
        # "Stop the VI"
        # "Release the message queue reference"
        # "#CodeNeeded - Add any required cleanup code here. Note that if 'Exit' was called as a result of an error, an error dialog will be displayed. Add any custom error handling for an 'Exit' condition here as well."
        # "Exit - Exit the application."
        n1279 = call "Fire User Event - Stop.vi"("User Event - Stop"=w2048) -> ("error out"=w2050:errorcluster)  [unwired: 10 in]
        n1280 = Release Queue(queue=w2055, error in (no error)=w2049) -> (error out=w2052:errorcluster)  [unwired: 1 in, 2 out]
        n1281 = Merge Errors(w2050, w2052) -> (w2051:errorcluster)
      }
      frame Default {
        # "'Default' case only runs if there is a message that isn't defined in any of the other cases.  Output a programming error."
        n1282 = xnode "Error Ring"("parameter 0"=w2056) -> ("error out"=w2057:errorcluster)
      }
    }
    n1283 = call "LAB-IQ Error Handler - Message Handling Loop.vi"("error in (no error)"=w1968, "Message Queue"=w1970) -> ("dup error in"=w1969:errorcluster)  [unwired: 8 in, 1 out]
  }
  n1284 = while {
    shift-right: [w2076] -> _
    shift-left: w14 -> [w2077]
    tunnel: [w2070] -> w1
    tunnel: w20 -> [w2068]
    tunnel: w4 -> [w2067]
    tunnel: w13 -> [w2066]
    stop <- w2075 stop-if-true
    # "Temperature  Handling Loop"
    n1285 = call "Dequeue Message.vi"("error in (no error)"=w2067, "Message Queue"=w2068) -> ("error out"=w2074:errorcluster, "Message Data"=w2072:variant, "Message"=w2073:string, "dup Message Queue"=w2071:refnum<queue>)  [unwired: 6 in]
    n1286 = case "Message Cases" shown="\"Temperature Main\"" w2073 {
      selector: w2073 -> [_ _ _ _ _ w2121]
      tunnel: w2071 -> [w2078 w2089 _ w2108 w2120 _]
      tunnel: w2074 -> [w2081 w2086 w2105 w2112 w2114 _]
      tunnel: [w2082 w2090 w2099 w2110 w2116 w2122] -> w2069
      tunnel: w2077 -> [w2080 w2088 w2104 w2111 w2119 w2123]
      tunnel: [w2080 w2088 w2104 w2111 w2119 w2123] -> w2076
      tunnel: [_ _ _ _ TRUE _] -> w2075
      tunnel: w2072 -> [_ _ w2103 _ _ _]
      tunnel: w2066 -> [_ _ _ _ w2113 _]
      frame "init" {
        # "Initialize - All initialization work should take place in this message, since other loops can potentially enqueue messages that execute immediately after this one."
        n1287 = call-poly "Enqueue Message.vi"("error in (no error)"=w2081, "Message"="Temperature Main", "Message Queue"=w2078) -> ("error out"=w2082:errorcluster)  [unwired: 7 in, 1 out]
      }
      frame "Temperature Main" {
        n1288 = Unbundle By Name(w2088) -> ("Main Home Screen.EXIT"=w2087:refnum<vi>)
        n1289 = property class="Bool (strict)"(reference=w2087) -> (reference out=w2084:refnum<vi>, error out=w2085:errorcluster, "Value"=w2083:bool)  [unwired: 1 in]
        n1290 = case shown="False" w2083 {
          tunnel: [w2093 w2097] -> w2090
          tunnel: w2089 -> [w2092 w2096]
          tunnel: w2086 -> [w2091 w2095]
          frame True {
            n1291 = call-poly "Enqueue Message.vi"("error in (no error)"=w2091, "Message"="Confirm Quit", "Message Queue"=w2092) -> ("error out"=w2093:errorcluster)  [unwired: 7 in, 1 out]
          }
          frame False {
            n1292 = call-poly "Enqueue Message.vi"("error in (no error)"=w2095, "Message"="Temperature Main", "Message Queue"=w2096) -> ("error out"=w2097:errorcluster)  [unwired: 7 in, 1 out]
          }
        }
        n1293 = Close Reference(reference=w2084, error in (no error)=w2085) -> ()  [unwired: 1 out]
      }
      frame "Error" {
        # "#CodeRecommended - If you ever change the name of this \"Error\" message, you'll need to update the name in the Check Loop Error.vi as well."
        # "#CodeRecommended - Consider creating a system for logging errors in some way. These errors are for notification purposes only. Handling of specific errors should be performed in the message frames that generated the error."
        # "Error - Display an error dialog. This message is sent by the \"Error Handler\" VIs at the end of other loops in this application."
        n1294 = Variant To Data(error in=w2105, type=errorcluster {"status"=FALSE, "code"=0, "source"=""} ("error constant"), Variant=w2103) -> (data=w2101:errorcluster, error out=w2100:errorcluster)
        n1295 = call <vilib>:"Simple Error Handler.vi"("error in (no error)"=w2101) -> ()  [unwired: 4 in, 5 out]
        n1296 = Merge Errors(w2100) -> (w2099:errorcluster)
      }
      frame "Confirm Quit" {
        # "#CodeNeeded - If you want to provide an \"Are you sure\" dialog (or some other notification) before the application exits, place that code here. This message is typically sent from a Panel Close? event."
        # "Confirm Quit - Message that can confirm whether or not the user wants to exit the application."
        n1297 = call-poly "Enqueue Message.vi"("Priority Message? (F)"=TRUE, "error in (no error)"=w2112, "Message"="Exit", "Message Queue"=w2108) -> ("error out"=w2109:errorcluster)  [unwired: 6 in, 1 out]
        n1298 = Merge Errors(w2109) -> (w2110:errorcluster)
      }
      frame "Exit" {
        # "Stop the VI"
        # "Release the message queue reference"
        # "#CodeNeeded - Add any required cleanup code here. Note that if 'Exit' was called as a result of an error, an error dialog will be displayed. Add any custom error handling for an 'Exit' condition here as well."
        # "Exit - Exit the application."
        n1299 = call "Fire User Event - Stop.vi"("User Event - Stop"=w2113) -> ("error out"=w2115:errorcluster)  [unwired: 10 in]
        n1300 = Release Queue(queue=w2120, error in (no error)=w2114) -> (error out=w2117:errorcluster)  [unwired: 1 in, 2 out]
        n1301 = Merge Errors(w2115, w2117) -> (w2116:errorcluster)
      }
      frame Default {
        # "'Default' case only runs if there is a message that isn't defined in any of the other cases.  Output a programming error."
        n1302 = xnode "Error Ring"("parameter 0"=w2121) -> ("error out"=w2122:errorcluster)
      }
    }
    n1303 = call "LAB-IQ Error Handler - Message Handling Loop.vi"("error in (no error)"=w2069, "Message Queue"=w2071) -> ("dup error in"=w2070:errorcluster)  [unwired: 8 in, 1 out]
  }
  n1304 = while {
    shift-right: [w2141] -> _
    shift-left: w14 -> [w2142]
    tunnel: [w2135] -> _
    tunnel: w18 -> [w2133]
    tunnel: w4 -> [w2132]
    tunnel: w13 -> [w2131]
    stop <- w2140 stop-if-true
    # "Ramp Motor  Handling Loop"
    n1305 = call "Dequeue Message.vi"("error in (no error)"=w2132, "Message Queue"=w2133) -> ("error out"=w2139:errorcluster, "Message Data"=w2137:variant, "Message"=w2138:string, "dup Message Queue"=w2136:refnum<queue>)  [unwired: 6 in]
    n1306 = case "Message Cases" shown="\"Ramp Main\"" w2138 {
      selector: w2138 -> [_ _ _ _ _ w2186]
      tunnel: w2136 -> [w2143 w2154 _ w2173 w2185 _]
      tunnel: w2139 -> [w2146 w2151 w2170 w2177 w2179 _]
      tunnel: [w2147 w2155 w2164 w2175 w2181 w2187] -> w2134
      tunnel: w2142 -> [w2145 w2153 w2169 w2176 w2184 w2188]
      tunnel: [w2145 w2153 w2169 w2176 w2184 w2188] -> w2141
      tunnel: [_ _ _ _ TRUE _] -> w2140
      tunnel: w2137 -> [_ _ w2168 _ _ _]
      tunnel: w2131 -> [_ _ _ _ w2178 _]
      frame "init" {
        # "Initialize - All initialization work should take place in this message, since other loops can potentially enqueue messages that execute immediately after this one."
        n1307 = call-poly "Enqueue Message.vi"("error in (no error)"=w2146, "Message"="Ramp Main", "Message Queue"=w2143) -> ("error out"=w2147:errorcluster)  [unwired: 7 in, 1 out]
      }
      frame "Ramp Main" {
        n1308 = Unbundle By Name(w2153) -> ("Main Home Screen.EXIT"=w2152:refnum<vi>)
        n1309 = property class="Bool (strict)"(reference=w2152) -> (reference out=w2149:refnum<vi>, error out=w2150:errorcluster, "Value"=w2148:bool)  [unwired: 1 in]
        n1310 = case shown="False" w2148 {
          tunnel: [w2158 w2162] -> w2155
          tunnel: w2154 -> [w2157 w2161]
          tunnel: w2151 -> [w2156 w2160]
          frame True {
            n1311 = call-poly "Enqueue Message.vi"("error in (no error)"=w2156, "Message"="Confirm Quit", "Message Queue"=w2157) -> ("error out"=w2158:errorcluster)  [unwired: 7 in, 1 out]
          }
          frame False {
            n1312 = call-poly "Enqueue Message.vi"("error in (no error)"=w2160, "Message"="Ramp Main", "Message Queue"=w2161) -> ("error out"=w2162:errorcluster)  [unwired: 7 in, 1 out]
          }
        }
        n1313 = Close Reference(reference=w2149, error in (no error)=w2150) -> ()  [unwired: 1 out]
      }
      frame "Error" {
        # "#CodeRecommended - If you ever change the name of this \"Error\" message, you'll need to update the name in the Check Loop Error.vi as well."
        # "#CodeRecommended - Consider creating a system for logging errors in some way. These errors are for notification purposes only. Handling of specific errors should be performed in the message frames that generated the error."
        # "Error - Display an error dialog. This message is sent by the \"Error Handler\" VIs at the end of other loops in this application."
        n1314 = Variant To Data(error in=w2170, type=errorcluster {"status"=FALSE, "code"=0, "source"=""} ("error constant"), Variant=w2168) -> (data=w2166:errorcluster, error out=w2165:errorcluster)
        n1315 = call <vilib>:"Simple Error Handler.vi"("error in (no error)"=w2166) -> ()  [unwired: 4 in, 5 out]
        n1316 = Merge Errors(w2165) -> (w2164:errorcluster)
      }
      frame "Confirm Quit" {
        # "#CodeNeeded - If you want to provide an \"Are you sure\" dialog (or some other notification) before the application exits, place that code here. This message is typically sent from a Panel Close? event."
        # "Confirm Quit - Message that can confirm whether or not the user wants to exit the application."
        n1317 = call-poly "Enqueue Message.vi"("Priority Message? (F)"=TRUE, "error in (no error)"=w2177, "Message"="Exit", "Message Queue"=w2173) -> ("error out"=w2174:errorcluster)  [unwired: 6 in, 1 out]
        n1318 = Merge Errors(w2174) -> (w2175:errorcluster)
      }
      frame "Exit" {
        # "Stop the VI"
        # "Release the message queue reference"
        # "#CodeNeeded - Add any required cleanup code here. Note that if 'Exit' was called as a result of an error, an error dialog will be displayed. Add any custom error handling for an 'Exit' condition here as well."
        # "Exit - Exit the application."
        n1319 = call "Fire User Event - Stop.vi"("User Event - Stop"=w2178) -> ("error out"=w2180:errorcluster)  [unwired: 10 in]
        n1320 = Release Queue(queue=w2185, error in (no error)=w2179) -> (error out=w2182:errorcluster)  [unwired: 1 in, 2 out]
        n1321 = Merge Errors(w2180, w2182) -> (w2181:errorcluster)
      }
      frame Default {
        # "'Default' case only runs if there is a message that isn't defined in any of the other cases.  Output a programming error."
        n1322 = xnode "Error Ring"("parameter 0"=w2186) -> ("error out"=w2187:errorcluster)
      }
    }
    n1323 = call "LAB-IQ Error Handler - Message Handling Loop.vi"("error in (no error)"=w2134, "Message Queue"=w2136) -> ("dup error in"=w2135:errorcluster)  [unwired: 8 in, 1 out]
  }
  n1324 = while {
    shift-right: [w2206] -> _
    shift-left: w14 -> [w2207]
    tunnel: [w2200] -> _
    tunnel: w17 -> [w2198]
    tunnel: w4 -> [w2197]
    tunnel: w13 -> [w2196]
    stop <- w2205 stop-if-true
    # "ECR  Handling Loop"
    n1325 = call "Dequeue Message.vi"("error in (no error)"=w2197, "Message Queue"=w2198) -> ("error out"=w2204:errorcluster, "Message Data"=w2202:variant, "Message"=w2203:string, "dup Message Queue"=w2201:refnum<queue>)  [unwired: 6 in]
    n1326 = case "Message Cases" shown="\"ECR Main\"" w2203 {
      selector: w2203 -> [_ _ _ _ _ w2251]
      tunnel: w2201 -> [w2208 w2219 _ w2238 w2250 _]
      tunnel: w2204 -> [w2211 w2216 w2235 w2242 w2244 _]
      tunnel: [w2212 w2220 w2229 w2240 w2246 w2252] -> w2199
      tunnel: w2207 -> [w2210 w2218 w2234 w2241 w2249 w2253]
      tunnel: [w2210 w2218 w2234 w2241 w2249 w2253] -> w2206
      tunnel: [_ _ _ _ TRUE _] -> w2205
      tunnel: w2202 -> [_ _ w2233 _ _ _]
      tunnel: w2196 -> [_ _ _ _ w2243 _]
      frame "init" {
        # "Initialize - All initialization work should take place in this message, since other loops can potentially enqueue messages that execute immediately after this one."
        n1327 = call-poly "Enqueue Message.vi"("error in (no error)"=w2211, "Message"="ECR Main", "Message Queue"=w2208) -> ("error out"=w2212:errorcluster)  [unwired: 7 in, 1 out]
      }
      frame "ECR Main" {
        n1328 = Unbundle By Name(w2218) -> ("Main Home Screen.EXIT"=w2217:refnum<vi>)
        n1329 = property class="Bool (strict)"(reference=w2217) -> (reference out=w2214:refnum<vi>, error out=w2215:errorcluster, "Value"=w2213:bool)  [unwired: 1 in]
        n1330 = case shown="False" w2213 {
          tunnel: [w2223 w2227] -> w2220
          tunnel: w2219 -> [w2222 w2226]
          tunnel: w2216 -> [w2221 w2225]
          frame True {
            n1331 = call-poly "Enqueue Message.vi"("error in (no error)"=w2221, "Message"="Confirm Quit", "Message Queue"=w2222) -> ("error out"=w2223:errorcluster)  [unwired: 7 in, 1 out]
          }
          frame False {
            n1332 = call-poly "Enqueue Message.vi"("error in (no error)"=w2225, "Message"="ECR Main", "Message Queue"=w2226) -> ("error out"=w2227:errorcluster)  [unwired: 7 in, 1 out]
          }
        }
        n1333 = Close Reference(reference=w2214, error in (no error)=w2215) -> ()  [unwired: 1 out]
      }
      frame "Error" {
        # "#CodeRecommended - If you ever change the name of this \"Error\" message, you'll need to update the name in the Check Loop Error.vi as well."
        # "#CodeRecommended - Consider creating a system for logging errors in some way. These errors are for notification purposes only. Handling of specific errors should be performed in the message frames that generated the error."
        # "Error - Display an error dialog. This message is sent by the \"Error Handler\" VIs at the end of other loops in this application."
        n1334 = Variant To Data(error in=w2235, type=errorcluster {"status"=FALSE, "code"=0, "source"=""} ("error constant"), Variant=w2233) -> (data=w2231:errorcluster, error out=w2230:errorcluster)
        n1335 = call <vilib>:"Simple Error Handler.vi"("error in (no error)"=w2231) -> ()  [unwired: 4 in, 5 out]
        n1336 = Merge Errors(w2230) -> (w2229:errorcluster)
      }
      frame "Confirm Quit" {
        # "#CodeNeeded - If you want to provide an \"Are you sure\" dialog (or some other notification) before the application exits, place that code here. This message is typically sent from a Panel Close? event."
        # "Confirm Quit - Message that can confirm whether or not the user wants to exit the application."
        n1337 = call-poly "Enqueue Message.vi"("Priority Message? (F)"=TRUE, "error in (no error)"=w2242, "Message"="Exit", "Message Queue"=w2238) -> ("error out"=w2239:errorcluster)  [unwired: 6 in, 1 out]
        n1338 = Merge Errors(w2239) -> (w2240:errorcluster)
      }
      frame "Exit" {
        # "Stop the VI"
        # "Release the message queue reference"
        # "#CodeNeeded - Add any required cleanup code here. Note that if 'Exit' was called as a result of an error, an error dialog will be displayed. Add any custom error handling for an 'Exit' condition here as well."
        # "Exit - Exit the application."
        n1339 = call "Fire User Event - Stop.vi"("User Event - Stop"=w2243) -> ("error out"=w2245:errorcluster)  [unwired: 10 in]
        n1340 = Release Queue(queue=w2250, error in (no error)=w2244) -> (error out=w2247:errorcluster)  [unwired: 1 in, 2 out]
        n1341 = Merge Errors(w2245, w2247) -> (w2246:errorcluster)
      }
      frame Default {
        # "'Default' case only runs if there is a message that isn't defined in any of the other cases.  Output a programming error."
        n1342 = xnode "Error Ring"("parameter 0"=w2251) -> ("error out"=w2252:errorcluster)
      }
    }
    n1343 = call "LAB-IQ Error Handler - Message Handling Loop.vi"("error in (no error)"=w2199, "Message Queue"=w2201) -> ("dup error in"=w2200:errorcluster)  [unwired: 8 in, 1 out]
  }
  n1344 = while {
    shift-right: [w2271] -> _
    shift-left: w14 -> [w2272]
    tunnel: [w2265] -> _
    tunnel: w16 -> [w2263]
    tunnel: w4 -> [w2262]
    tunnel: w13 -> [w2261]
    stop <- w2270 stop-if-true
    # "Humidity  Handling Loop"
    n1345 = call "Dequeue Message.vi"("error in (no error)"=w2262, "Message Queue"=w2263) -> ("error out"=w2269:errorcluster, "Message Data"=w2267:variant, "Message"=w2268:string, "dup Message Queue"=w2266:refnum<queue>)  [unwired: 6 in]
    n1346 = case "Message Cases" shown="\"Humidity Main\"" w2268 {
      selector: w2268 -> [_ _ _ _ _ w2316]
      tunnel: w2266 -> [w2273 w2284 _ w2303 w2315 _]
      tunnel: w2269 -> [w2276 w2281 w2300 w2307 w2309 _]
      tunnel: [w2277 w2285 w2294 w2305 w2311 w2317] -> w2264
      tunnel: w2272 -> [w2275 w2283 w2299 w2306 w2314 w2318]
      tunnel: [w2275 w2283 w2299 w2306 w2314 w2318] -> w2271
      tunnel: [_ _ _ _ TRUE _] -> w2270
      tunnel: w2267 -> [_ _ w2298 _ _ _]
      tunnel: w2261 -> [_ _ _ _ w2308 _]
      frame "init" {
        # "Initialize - All initialization work should take place in this message, since other loops can potentially enqueue messages that execute immediately after this one."
        n1347 = call-poly "Enqueue Message.vi"("error in (no error)"=w2276, "Message"="Humidity Main", "Message Queue"=w2273) -> ("error out"=w2277:errorcluster)  [unwired: 7 in, 1 out]
      }
      frame "Humidity Main" {
        n1348 = Unbundle By Name(w2283) -> ("Main Home Screen.EXIT"=w2282:refnum<vi>)
        n1349 = property class="Bool (strict)"(reference=w2282) -> (reference out=w2279:refnum<vi>, error out=w2280:errorcluster, "Value"=w2278:bool)  [unwired: 1 in]
        n1350 = case shown="False" w2278 {
          tunnel: [w2288 w2292] -> w2285
          tunnel: w2284 -> [w2287 w2291]
          tunnel: w2281 -> [w2286 w2290]
          frame True {
            n1351 = call-poly "Enqueue Message.vi"("error in (no error)"=w2286, "Message"="Confirm Quit", "Message Queue"=w2287) -> ("error out"=w2288:errorcluster)  [unwired: 7 in, 1 out]
          }
          frame False {
            n1352 = call-poly "Enqueue Message.vi"("error in (no error)"=w2290, "Message"="Humidity Main", "Message Queue"=w2291) -> ("error out"=w2292:errorcluster)  [unwired: 7 in, 1 out]
          }
        }
        n1353 = Close Reference(reference=w2279, error in (no error)=w2280) -> ()  [unwired: 1 out]
      }
      frame "Error" {
        # "#CodeRecommended - If you ever change the name of this \"Error\" message, you'll need to update the name in the Check Loop Error.vi as well."
        # "#CodeRecommended - Consider creating a system for logging errors in some way. These errors are for notification purposes only. Handling of specific errors should be performed in the message frames that generated the error."
        # "Error - Display an error dialog. This message is sent by the \"Error Handler\" VIs at the end of other loops in this application."
        n1354 = Variant To Data(error in=w2300, type=errorcluster {"status"=FALSE, "code"=0, "source"=""} ("error constant"), Variant=w2298) -> (data=w2296:errorcluster, error out=w2295:errorcluster)
        n1355 = call <vilib>:"Simple Error Handler.vi"("error in (no error)"=w2296) -> ()  [unwired: 4 in, 5 out]
        n1356 = Merge Errors(w2295) -> (w2294:errorcluster)
      }
      frame "Confirm Quit" {
        # "#CodeNeeded - If you want to provide an \"Are you sure\" dialog (or some other notification) before the application exits, place that code here. This message is typically sent from a Panel Close? event."
        # "Confirm Quit - Message that can confirm whether or not the user wants to exit the application."
        n1357 = call-poly "Enqueue Message.vi"("Priority Message? (F)"=TRUE, "error in (no error)"=w2307, "Message"="Exit", "Message Queue"=w2303) -> ("error out"=w2304:errorcluster)  [unwired: 6 in, 1 out]
        n1358 = Merge Errors(w2304) -> (w2305:errorcluster)
      }
      frame "Exit" {
        # "Stop the VI"
        # "Release the message queue reference"
        # "#CodeNeeded - Add any required cleanup code here. Note that if 'Exit' was called as a result of an error, an error dialog will be displayed. Add any custom error handling for an 'Exit' condition here as well."
        # "Exit - Exit the application."
        n1359 = call "Fire User Event - Stop.vi"("User Event - Stop"=w2308) -> ("error out"=w2310:errorcluster)  [unwired: 10 in]
        n1360 = Release Queue(queue=w2315, error in (no error)=w2309) -> (error out=w2312:errorcluster)  [unwired: 1 in, 2 out]
        n1361 = Merge Errors(w2310, w2312) -> (w2311:errorcluster)
      }
      frame Default {
        # "'Default' case only runs if there is a message that isn't defined in any of the other cases.  Output a programming error."
        n1362 = xnode "Error Ring"("parameter 0"=w2316) -> ("error out"=w2317:errorcluster)
      }
    }
    n1363 = call "LAB-IQ Error Handler - Message Handling Loop.vi"("error in (no error)"=w2264, "Message Queue"=w2266) -> ("dup error in"=w2265:errorcluster)  [unwired: 8 in, 1 out]
  }
  n1364 = while {
    shift-right: [w2336] -> _
    shift-left: w14 -> [w2337]
    tunnel: [w2330] -> _
    tunnel: w15 -> [w2328]
    tunnel: w4 -> [w2327]
    tunnel: w13 -> [w2326]
    stop <- w2335 stop-if-true
    # "Program  Handling Loop"
    n1365 = call "Dequeue Message.vi"("error in (no error)"=w2327, "Message Queue"=w2328) -> ("error out"=w2334:errorcluster, "Message Data"=w2332:variant, "Message"=w2333:string, "dup Message Queue"=w2331:refnum<queue>)  [unwired: 6 in]
    n1366 = case "Message Cases" shown="\"Program Main\"" w2333 {
      selector: w2333 -> [_ _ _ _ _ w2384]
      tunnel: w2331 -> [w2338 w2352 _ w2371 w2383 _]
      tunnel: w2334 -> [w2341 w2345 w2368 w2375 w2377 _]
      tunnel: [w2342 w2353 w2362 w2373 w2379 w2385] -> w2329
      tunnel: w2337 -> [w2340 w2346 w2367 w2374 w2382 w2386]
      tunnel: [w2340 w2346 w2367 w2374 w2382 w2386] -> w2336
      tunnel: [_ _ _ _ TRUE _] -> w2335
      tunnel: w2332 -> [_ _ w2366 _ _ _]
      tunnel: w2326 -> [_ _ _ _ w2376 _]
      frame "init" {
        # "Initialize - All initialization work should take place in this message, since other loops can potentially enqueue messages that execute immediately after this one."
        n1367 = call-poly "Enqueue Message.vi"("error in (no error)"=w2341, "Message"="Program Main", "Message Queue"=w2338) -> ("error out"=w2342:errorcluster)  [unwired: 7 in, 1 out]
      }
      frame "Program Main" {
        n1368 = call "LOAD SELECTION MAIN CODE.vi"("error in (no error)"=w2345, "main ref"=w2346) -> ("error out"=w2347:errorcluster)  [unwired: 9 in]
        n1369 = call "STEP LOAD SEQUENCE.vi"("error in (no error)"=w2345, "main ref"=w2346) -> ("error out"=w2343:errorcluster)  [unwired: 9 in]
        n1370 = Merge Errors(w2347, w2343) -> (w2344:errorcluster)
        n1371 = Unbundle By Name(w2346) -> ("Main Home Screen.EXIT"=w2351:refnum<vi>)
        n1372 = property class="Bool (strict)"(reference=w2351) -> (reference out=w2349:refnum<vi>, error out=w2350:errorcluster, "Value"=w2348:bool)  [unwired: 1 in]
        n1373 = case shown="False" w2348 {
          tunnel: [w2356 w2360] -> w2353
          tunnel: w2352 -> [w2355 w2359]
          tunnel: w2344 -> [w2354 w2358]
          frame True {
            n1374 = call-poly "Enqueue Message.vi"("error in (no error)"=w2354, "Message"="Confirm Quit", "Message Queue"=w2355) -> ("error out"=w2356:errorcluster)  [unwired: 7 in, 1 out]
          }
          frame False {
            n1375 = call-poly "Enqueue Message.vi"("error in (no error)"=w2358, "Message"="Program Main", "Message Queue"=w2359) -> ("error out"=w2360:errorcluster)  [unwired: 7 in, 1 out]
          }
        }
        n1376 = Close Reference(reference=w2349, error in (no error)=w2350) -> ()  [unwired: 1 out]
      }
      frame "Error" {
        # "#CodeRecommended - If you ever change the name of this \"Error\" message, you'll need to update the name in the Check Loop Error.vi as well."
        # "#CodeRecommended - Consider creating a system for logging errors in some way. These errors are for notification purposes only. Handling of specific errors should be performed in the message frames that generated the error."
        # "Error - Display an error dialog. This message is sent by the \"Error Handler\" VIs at the end of other loops in this application."
        n1377 = Variant To Data(error in=w2368, type=errorcluster {"status"=FALSE, "code"=0, "source"=""} ("error constant"), Variant=w2366) -> (data=w2364:errorcluster, error out=w2363:errorcluster)
        n1378 = call <vilib>:"Simple Error Handler.vi"("error in (no error)"=w2364) -> ()  [unwired: 4 in, 5 out]
        n1379 = Merge Errors(w2363) -> (w2362:errorcluster)
      }
      frame "Confirm Quit" {
        # "#CodeNeeded - If you want to provide an \"Are you sure\" dialog (or some other notification) before the application exits, place that code here. This message is typically sent from a Panel Close? event."
        # "Confirm Quit - Message that can confirm whether or not the user wants to exit the application."
        n1380 = call-poly "Enqueue Message.vi"("Priority Message? (F)"=TRUE, "error in (no error)"=w2375, "Message"="Exit", "Message Queue"=w2371) -> ("error out"=w2372:errorcluster)  [unwired: 6 in, 1 out]
        n1381 = Merge Errors(w2372) -> (w2373:errorcluster)
      }
      frame "Exit" {
        # "Stop the VI"
        # "Release the message queue reference"
        # "#CodeNeeded - Add any required cleanup code here. Note that if 'Exit' was called as a result of an error, an error dialog will be displayed. Add any custom error handling for an 'Exit' condition here as well."
        # "Exit - Exit the application."
        n1382 = call "Fire User Event - Stop.vi"("User Event - Stop"=w2376) -> ("error out"=w2378:errorcluster)  [unwired: 10 in]
        n1383 = Release Queue(queue=w2383, error in (no error)=w2377) -> (error out=w2380:errorcluster)  [unwired: 1 in, 2 out]
        n1384 = Merge Errors(w2378, w2380) -> (w2379:errorcluster)
      }
      frame Default {
        # "'Default' case only runs if there is a message that isn't defined in any of the other cases.  Output a programming error."
        n1385 = xnode "Error Ring"("parameter 0"=w2384) -> ("error out"=w2385:errorcluster)
      }
    }
    n1386 = call "LAB-IQ Error Handler - Message Handling Loop.vi"("error in (no error)"=w2329, "Message Queue"=w2331) -> ("dup error in"=w2330:errorcluster)  [unwired: 8 in, 1 out]
  }
  n1387 = while {
    shift-right: [w2404] -> _
    shift-left: w14 -> [w2405]
    tunnel: [w2398] -> _
    tunnel: w12 -> [w2396]
    tunnel: w4 -> [w2395]
    tunnel: w13 -> [w2394]
    stop <- w2403 stop-if-true
    # "Monitor  Handling Loop"
    n1388 = call "Dequeue Message.vi"("error in (no error)"=w2395, "Message Queue"=w2396) -> ("error out"=w2402:errorcluster, "Message Data"=w2400:variant, "Message"=w2401:string, "dup Message Queue"=w2399:refnum<queue>)  [unwired: 6 in]
    n1389 = case "Message Cases" shown="\"Monitor Main\"" w2401 {
      selector: w2401 -> [_ _ _ _ _ w2450]
      tunnel: w2399 -> [w2406 w2418 _ w2437 w2449 _]
      tunnel: w2402 -> [w2409 w2416 w2434 w2441 w2443 _]
      tunnel: [w2410 w2419 w2428 w2439 w2445 w2451] -> w2397
      tunnel: w2405 -> [w2408 w2411 w2433 w2440 w2448 w2452]
      tunnel: [w2408 w2411 w2433 w2440 w2448 w2452] -> w2404
      tunnel: [_ _ _ _ TRUE _] -> w2403
      tunnel: w2400 -> [_ _ w2432 _ _ _]
      tunnel: w2394 -> [_ _ _ _ w2442 _]
      frame "init" {
        # "Initialize - All initialization work should take place in this message, since other loops can potentially enqueue messages that execute immediately after this one."
        n1390 = call-poly "Enqueue Message.vi"("error in (no error)"=w2409, "Message"="Monitor Main", "Message Queue"=w2406) -> ("error out"=w2410:errorcluster)  [unwired: 7 in, 1 out]
      }
      frame "Monitor Main" {
        n1391 = call "Main Monitor Loop.vi"("error in (no error)"=w2416, "main ref"=w2411) -> ("error out"=w2412:errorcluster)  [unwired: 9 in]
        n1392 = Unbundle By Name(w2411) -> ("Main Home Screen.EXIT"=w2417:refnum<vi>)
        n1393 = property class="Bool (strict)"(reference=w2417) -> (reference out=w2414:refnum<vi>, error out=w2415:errorcluster, "Value"=w2413:bool)  [unwired: 1 in]
        n1394 = case shown="False" w2413 {
          tunnel: [w2422 w2426] -> w2419
          tunnel: w2418 -> [w2421 w2425]
          tunnel: w2412 -> [w2420 w2424]
          frame True {
            n1395 = call-poly "Enqueue Message.vi"("error in (no error)"=w2420, "Message"="Confirm Quit", "Message Queue"=w2421) -> ("error out"=w2422:errorcluster)  [unwired: 7 in, 1 out]
          }
          frame False {
            n1396 = call-poly "Enqueue Message.vi"("error in (no error)"=w2424, "Message"="Monitor Main", "Message Queue"=w2425) -> ("error out"=w2426:errorcluster)  [unwired: 7 in, 1 out]
          }
        }
        n1397 = Close Reference(reference=w2414, error in (no error)=w2415) -> ()  [unwired: 1 out]
      }
      frame "Error" {
        # "#CodeRecommended - If you ever change the name of this \"Error\" message, you'll need to update the name in the Check Loop Error.vi as well."
        # "#CodeRecommended - Consider creating a system for logging errors in some way. These errors are for notification purposes only. Handling of specific errors should be performed in the message frames that generated the error."
        # "Error - Display an error dialog. This message is sent by the \"Error Handler\" VIs at the end of other loops in this application."
        n1398 = Variant To Data(error in=w2434, type=errorcluster {"status"=FALSE, "code"=0, "source"=""} ("error constant"), Variant=w2432) -> (data=w2430:errorcluster, error out=w2429:errorcluster)
        n1399 = call <vilib>:"Simple Error Handler.vi"("error in (no error)"=w2430) -> ()  [unwired: 4 in, 5 out]
        n1400 = Merge Errors(w2429) -> (w2428:errorcluster)
      }
      frame "Confirm Quit" {
        # "#CodeNeeded - If you want to provide an \"Are you sure\" dialog (or some other notification) before the application exits, place that code here. This message is typically sent from a Panel Close? event."
        # "Confirm Quit - Message that can confirm whether or not the user wants to exit the application."
        n1401 = call-poly "Enqueue Message.vi"("Priority Message? (F)"=TRUE, "error in (no error)"=w2441, "Message"="Exit", "Message Queue"=w2437) -> ("error out"=w2438:errorcluster)  [unwired: 6 in, 1 out]
        n1402 = Merge Errors(w2438) -> (w2439:errorcluster)
      }
      frame "Exit" {
        # "Stop the VI"
        # "Release the message queue reference"
        # "#CodeNeeded - Add any required cleanup code here. Note that if 'Exit' was called as a result of an error, an error dialog will be displayed. Add any custom error handling for an 'Exit' condition here as well."
        # "Exit - Exit the application."
        n1403 = call "Fire User Event - Stop.vi"("User Event - Stop"=w2442) -> ("error out"=w2444:errorcluster)  [unwired: 10 in]
        n1404 = Release Queue(queue=w2449, error in (no error)=w2443) -> (error out=w2446:errorcluster)  [unwired: 1 in, 2 out]
        n1405 = Merge Errors(w2444, w2446) -> (w2445:errorcluster)
      }
      frame Default {
        # "'Default' case only runs if there is a message that isn't defined in any of the other cases.  Output a programming error."
        n1406 = xnode "Error Ring"("parameter 0"=w2450) -> ("error out"=w2451:errorcluster)
      }
    }
    n1407 = call "LAB-IQ Error Handler - Message Handling Loop.vi"("error in (no error)"=w2397, "Message Queue"=w2399) -> ("dup error in"=w2398:errorcluster)  [unwired: 8 in, 1 out]
  }
  n1408 = while {
    shift-right: [w2470] -> _
    shift-left: w14 -> [w2471]
    tunnel: [w2464] -> _
    tunnel: w11 -> [w2462]
    tunnel: w4 -> [w2461]
    tunnel: w13 -> [w2460]
    stop <- w2469 stop-if-true
    # "Load Pid  Handling Loop"
    n1409 = call "Dequeue Message.vi"("error in (no error)"=w2461, "Message Queue"=w2462) -> ("error out"=w2468:errorcluster, "Message Data"=w2466:variant, "Message"=w2467:string, "dup Message Queue"=w2465:refnum<queue>)  [unwired: 6 in]
    n1410 = case "Message Cases" shown="\"Load Pid Main\"" w2467 {
      selector: w2467 -> [_ _ _ _ _ w2536]
      tunnel: w2465 -> [w2472 w2493 _ w2523 w2535 _]
      tunnel: w2468 -> [w2475 w2491 w2520 w2527 w2529 _]
      tunnel: [w2476 w2494 w2514 w2525 w2531 w2537] -> w2463
      tunnel: w2471 -> [w2474 w2480 w2519 w2526 w2534 w2538]
      tunnel: [w2474 w2480 w2519 w2526 w2534 w2538] -> w2470
      tunnel: [_ _ _ _ TRUE _] -> w2469
      tunnel: w2466 -> [_ _ w2518 _ _ _]
      tunnel: w2460 -> [_ _ _ _ w2528 _]
      frame "init" {
        # "Initialize - All initialization work should take place in this message, since other loops can potentially enqueue messages that execute immediately after this one."
        n1411 = call-poly "Enqueue Message.vi"("error in (no error)"=w2475, "Message"="Load Pid Main", "Message Queue"=w2472) -> ("error out"=w2476:errorcluster)  [unwired: 7 in, 1 out]
      }
      frame "Load Pid Main" {
        n1412 = Unbundle By Name(w2480) -> ("Main Screen.Load En"=w2486:refnum<vi>)
        n1413 = Unbundle By Name(w2480) -> ("PID.apply load"=w2481:refnum<vi>)
        n1414 = property class="Bool (strict)"(reference=w2486) -> (reference out=w2484:refnum<vi>, error out=w2485:errorcluster, "Value"=w2479:bool)  [unwired: 1 in]
        n1415 = property class="Bool (strict)"(reference=w2481) -> (reference out=w2483:refnum<vi>, error out=w2482:errorcluster, "Value"=w2478:bool)  [unwired: 1 in]
        n1416 = Close Reference(reference=w2484, error in (no error)=w2485) -> ()  [unwired: 1 out]
        n1417 = Close Reference(reference=w2483, error in (no error)=w2482) -> ()  [unwired: 1 out]
        n1418 = Or(x=w2479, y=w2478) -> (x .or. y?=w2477:bool)
        n1419 = case shown="True" w2477 {
          tunnel: w2491 -> [w2495 w2498]
          tunnel: [w2495 w2497] -> w2487
          tunnel: w2480 -> [_ w2496]
          frame False {
          }
          frame True {
            n1420 = disable-structure shown="Disabled" {
              disable-tunnel: w2498 -> [w2501 w2505]
              disable-tunnel: [w2500 w2504] -> w2497
              disable-tunnel: w2496 -> [w2499 w2503]
              frame Disabled {
                n1421 = call "load pid.vi"("error in (no error)"=w2501, "main ref"=w2499) -> ("error out"=w2500:errorcluster)  [unwired: 9 in]
              }
              frame Enabled {
                n1422 = call "NEW LOAD CELL PID.vi"("error in (no error)"=w2505, "Checkbox"=TRUE, "main ref"=w2503) -> ("error out"=w2504:errorcluster)  [unwired: 8 in]
              }
            }
          }
        }
        n1423 = Unbundle By Name(w2480) -> ("Main Home Screen.EXIT"=w2492:refnum<vi>)
        n1424 = property class="Bool (strict)"(reference=w2492) -> (reference out=w2489:refnum<vi>, error out=w2490:errorcluster, "Value"=w2488:bool)  [unwired: 1 in]
        n1425 = case shown="False" w2488 {
          tunnel: [w2508 w2512] -> w2494
          tunnel: w2493 -> [w2507 w2511]
          tunnel: w2487 -> [w2506 w2510]
          frame True {
            n1426 = call-poly "Enqueue Message.vi"("error in (no error)"=w2506, "Message"="Confirm Quit", "Message Queue"=w2507) -> ("error out"=w2508:errorcluster)  [unwired: 7 in, 1 out]
          }
          frame False {
            n1427 = call-poly "Enqueue Message.vi"("error in (no error)"=w2510, "Message"="Load Pid Main", "Message Queue"=w2511) -> ("error out"=w2512:errorcluster)  [unwired: 7 in, 1 out]
          }
        }
        n1428 = Close Reference(reference=w2489, error in (no error)=w2490) -> ()  [unwired: 1 out]
      }
      frame "Error" {
        # "#CodeRecommended - If you ever change the name of this \"Error\" message, you'll need to update the name in the Check Loop Error.vi as well."
        # "#CodeRecommended - Consider creating a system for logging errors in some way. These errors are for notification purposes only. Handling of specific errors should be performed in the message frames that generated the error."
        # "Error - Display an error dialog. This message is sent by the \"Error Handler\" VIs at the end of other loops in this application."
        n1429 = Variant To Data(error in=w2520, type=errorcluster {"status"=FALSE, "code"=0, "source"=""} ("error constant"), Variant=w2518) -> (data=w2516:errorcluster, error out=w2515:errorcluster)
        n1430 = call <vilib>:"Simple Error Handler.vi"("error in (no error)"=w2516) -> ()  [unwired: 4 in, 5 out]
        n1431 = Merge Errors(w2515) -> (w2514:errorcluster)
      }
      frame "Confirm Quit" {
        # "#CodeNeeded - If you want to provide an \"Are you sure\" dialog (or some other notification) before the application exits, place that code here. This message is typically sent from a Panel Close? event."
        # "Confirm Quit - Message that can confirm whether or not the user wants to exit the application."
        n1432 = call-poly "Enqueue Message.vi"("Priority Message? (F)"=TRUE, "error in (no error)"=w2527, "Message"="Exit", "Message Queue"=w2523) -> ("error out"=w2524:errorcluster)  [unwired: 6 in, 1 out]
        n1433 = Merge Errors(w2524) -> (w2525:errorcluster)
      }
      frame "Exit" {
        # "Stop the VI"
        # "Release the message queue reference"
        # "#CodeNeeded - Add any required cleanup code here. Note that if 'Exit' was called as a result of an error, an error dialog will be displayed. Add any custom error handling for an 'Exit' condition here as well."
        # "Exit - Exit the application."
        n1434 = call "Fire User Event - Stop.vi"("User Event - Stop"=w2528) -> ("error out"=w2530:errorcluster)  [unwired: 10 in]
        n1435 = Release Queue(queue=w2535, error in (no error)=w2529) -> (error out=w2532:errorcluster)  [unwired: 1 in, 2 out]
        n1436 = Merge Errors(w2530, w2532) -> (w2531:errorcluster)
      }
      frame Default {
        # "'Default' case only runs if there is a message that isn't defined in any of the other cases.  Output a programming error."
        n1437 = xnode "Error Ring"("parameter 0"=w2536) -> ("error out"=w2537:errorcluster)
      }
    }
    n1438 = call "LAB-IQ Error Handler - Message Handling Loop.vi"("error in (no error)"=w2463, "Message Queue"=w2465) -> ("dup error in"=w2464:errorcluster)  [unwired: 8 in, 1 out]
  }
  n1439 = while {
    shift-right: [w2556] -> _
    shift-left: w14 -> [w2557]
    tunnel: [w2550] -> _
    tunnel: w10 -> [w2548]
    tunnel: w4 -> [w2547]
    tunnel: w13 -> [w2546]
    stop <- w2555 stop-if-true
    # "Report  Handling Loop"
    n1440 = call "Dequeue Message.vi"("error in (no error)"=w2547, "Message Queue"=w2548) -> ("error out"=w2554:errorcluster, "Message Data"=w2552:variant, "Message"=w2553:string, "dup Message Queue"=w2551:refnum<queue>)  [unwired: 6 in]
    n1441 = case "Message Cases" shown="\"Report Main\"" w2553 {
      selector: w2553 -> [_ _ _ _ _ w2601]
      tunnel: w2551 -> [w2558 w2569 _ w2588 w2600 _]
      tunnel: w2554 -> [w2561 w2566 w2585 w2592 w2594 _]
      tunnel: [w2562 w2570 w2579 w2590 w2596 w2602] -> w2549
      tunnel: w2557 -> [w2560 w2568 w2584 w2591 w2599 w2603]
      tunnel: [w2560 w2568 w2584 w2591 w2599 w2603] -> w2556
      tunnel: [_ _ _ _ TRUE _] -> w2555
      tunnel: w2552 -> [_ _ w2583 _ _ _]
      tunnel: w2546 -> [_ _ _ _ w2593 _]
      frame "init" {
        # "Initialize - All initialization work should take place in this message, since other loops can potentially enqueue messages that execute immediately after this one."
        n1442 = call-poly "Enqueue Message.vi"("error in (no error)"=w2561, "Message"="Report Main", "Message Queue"=w2558) -> ("error out"=w2562:errorcluster)  [unwired: 7 in, 1 out]
      }
      frame "Report Main" {
        n1443 = Unbundle By Name(w2568) -> ("Main Home Screen.EXIT"=w2567:refnum<vi>)
        n1444 = property class="Bool (strict)"(reference=w2567) -> (reference out=w2564:refnum<vi>, error out=w2565:errorcluster, "Value"=w2563:bool)  [unwired: 1 in]
        n1445 = case shown="False" w2563 {
          tunnel: [w2573 w2577] -> w2570
          tunnel: w2569 -> [w2572 w2576]
          tunnel: w2566 -> [w2571 w2575]
          frame True {
            n1446 = call-poly "Enqueue Message.vi"("error in (no error)"=w2571, "Message"="Confirm Quit", "Message Queue"=w2572) -> ("error out"=w2573:errorcluster)  [unwired: 7 in, 1 out]
          }
          frame False {
            n1447 = call-poly "Enqueue Message.vi"("error in (no error)"=w2575, "Message"="Report Main", "Message Queue"=w2576) -> ("error out"=w2577:errorcluster)  [unwired: 7 in, 1 out]
          }
        }
        n1448 = Close Reference(reference=w2564, error in (no error)=w2565) -> ()  [unwired: 1 out]
      }
      frame "Error" {
        # "#CodeRecommended - If you ever change the name of this \"Error\" message, you'll need to update the name in the Check Loop Error.vi as well."
        # "#CodeRecommended - Consider creating a system for logging errors in some way. These errors are for notification purposes only. Handling of specific errors should be performed in the message frames that generated the error."
        # "Error - Display an error dialog. This message is sent by the \"Error Handler\" VIs at the end of other loops in this application."
        n1449 = Variant To Data(error in=w2585, type=errorcluster {"status"=FALSE, "code"=0, "source"=""} ("error constant"), Variant=w2583) -> (data=w2581:errorcluster, error out=w2580:errorcluster)
        n1450 = call <vilib>:"Simple Error Handler.vi"("error in (no error)"=w2581) -> ()  [unwired: 4 in, 5 out]
        n1451 = Merge Errors(w2580) -> (w2579:errorcluster)
      }
      frame "Confirm Quit" {
        # "#CodeNeeded - If you want to provide an \"Are you sure\" dialog (or some other notification) before the application exits, place that code here. This message is typically sent from a Panel Close? event."
        # "Confirm Quit - Message that can confirm whether or not the user wants to exit the application."
        n1452 = call-poly "Enqueue Message.vi"("Priority Message? (F)"=TRUE, "error in (no error)"=w2592, "Message"="Exit", "Message Queue"=w2588) -> ("error out"=w2589:errorcluster)  [unwired: 6 in, 1 out]
        n1453 = Merge Errors(w2589) -> (w2590:errorcluster)
      }
      frame "Exit" {
        # "Stop the VI"
        # "Release the message queue reference"
        # "#CodeNeeded - Add any required cleanup code here. Note that if 'Exit' was called as a result of an error, an error dialog will be displayed. Add any custom error handling for an 'Exit' condition here as well."
        # "Exit - Exit the application."
        n1454 = call "Fire User Event - Stop.vi"("User Event - Stop"=w2593) -> ("error out"=w2595:errorcluster)  [unwired: 10 in]
        n1455 = Release Queue(queue=w2600, error in (no error)=w2594) -> (error out=w2597:errorcluster)  [unwired: 1 in, 2 out]
        n1456 = Merge Errors(w2595, w2597) -> (w2596:errorcluster)
      }
      frame Default {
        # "'Default' case only runs if there is a message that isn't defined in any of the other cases.  Output a programming error."
        n1457 = xnode "Error Ring"("parameter 0"=w2601) -> ("error out"=w2602:errorcluster)
      }
    }
    n1458 = call "LAB-IQ Error Handler - Message Handling Loop.vi"("error in (no error)"=w2549, "Message Queue"=w2551) -> ("dup error in"=w2550:errorcluster)  [unwired: 8 in, 1 out]
  }
  n1459 = Unregister For Events(event registration refnum=w48, error in=w46) -> (error out=w49:errorcluster)
  n1460 = Merge Errors(w49, w52, w24, w21, w19, w1) -> (w50:errorcluster)
  n1461 = call "Destroy User Event - Stop.vi"("error in (no error)"=w50, "User Event - Stop"=w13) -> ("error out"=w47:errorcluster)  [unwired: 9 in]
  n1462 = disable-structure shown="RUN_TIME_ENGINE==True" {
    disable-tunnel: w47 -> [_ _]
    frame condition #0 (active) {
    }
    frame condition #1 {
      # "Call Quit LabVIEW if running as a built application."
      n1463 = Quit LabVIEW() -> ()  [unwired: 1 in]
    }
  }
